vi "Two Parameter.vi"() -> ()   [LabVIEW 2015]
uses:
  <vilib>/Platform/TimedLoop/XDataNode/timing_clust.ctl
  <vilib>/Platform/TimedLoop/XDataNode/nitl_modes.ctl
  <vilib>/Platform/TimedLoop/XDataNode/wakeup.ctl
  <vilib>/DAQmx/read.llb/DAQmx Read (Analog DBL 1Chan 1Samp).vi
  <vilib>/DAQmx/read.llb/DAQmx Read (Analog 1D DBL NChan 1Samp).vi
  <vilib>/DAQmx/create/channels.llb/DAQmx Create Channel (AI-Voltage-Basic).vi
  <vilib>/Enthought/Python Integration Toolkit/api/Unpack Double.vi
  <vilib>/DAQmx/miscellaneous.llb/DAQmx Fill In Error Info.vi
  <vilib>/Platform/TimedLoop/XDataNode/XDataNode.xnode
  Program Files/neMESYS_SDK/neMESYS LabVIEW Kit/neMESYS LabVIEW Integration Kit.lvlib
  <vilib>/Platform/TimedLoop/XDataNode/XDNodeRunTimeDep.lvlib
  Conor/Temp CN7500/Omega CN7500/Omega CN7500.lvlib
  <vilib>/Enthought/Python Integration Toolkit/Python Integration Toolkit.lvlib
panel:
  out "Exp 2":bool
  out "C EB 1":dbl
  out "C BAcid 1":dbl
  out "t ref 8":dbl
  out "t 2 8":dbl
  out "t 1 8":dbl
  out "t ref 7":dbl
  out "t 2 7":dbl
  out "t 1 7":dbl
  out "t ref 6":dbl
  out "t 2 6":dbl
  out "t 1 6":dbl
  out "t ref 5":dbl
  out "t 2 5":dbl
  out "t 1 5":dbl
  out "t ref 4":dbl
  out "t 2 4":dbl
  out "t 1 4":dbl
  out "t ref 3":dbl
  out "t 2 3":dbl
  out "t 1 3":dbl
  out "t ref 2":dbl
  out "t 2 2":dbl
  out "t 1 2":dbl
  out "Exp 9":bool
  out "Liquid Inlet Pressure (bar g)":dbl
  in  "Liquid P sensor Terminal Configuration":i32(ring)=-1 items=["default"=-1, "RSE"=10083, "NRSE"=10078, "Differential"=10106, "Pseudodifferential"=12529]
  in  "Liquid P sensor Physical Channel":tag="Dev1/ai0"
  in  "Temp 2":dbl
  in  "Conc 2":dbl
  in  "Flow 2":dbl
  out "C Int 2 8":dbl
  out "C Int 1 8":dbl
  out "C Int 2 7":dbl
  out "C Int 1 7":dbl
  out "C Int 2 6":dbl
  out "C Int 1 6":dbl
  out "C Int 2 5":dbl
  out "C Int 1 5":dbl
  out "C Int 2 4":dbl
  out "C Int 1 4":dbl
  out "C Int 2 3":dbl
  out "C Int 1 3":dbl
  out "C Int 2 2":dbl
  out "C Int 1 2":dbl
  out "Exp 8":bool
  out "Exp 7":bool
  out "Exp 6":bool
  out "Exp 5":bool
  out "Exp 4":bool
  out "Exp 3":bool
  out "Exp 1":bool
  out "Exp 0":bool
  out "Number Read":dbl
  out "Param 1 8":dbl
  out "Param 2 8":dbl
  out "Chi  8":dbl
  out "Chi ref 8":dbl
  out "C BAcid 8":dbl
  out "C EB 8":dbl
  in  "Flow 8":dbl
  in  "Conc 8":dbl
  in  "Temp 8":dbl
  out "Temp 8":dbl
  out "Flow 8":dbl
  out "Conc 8":dbl
  out "Param 1 7":dbl
  out "Param 2 7":dbl
  out "Chi  7":dbl
  out "Chi ref 7":dbl
  out "C BAcid 7":dbl
  out "C EB 7":dbl
  in  "Flow 7":dbl
  in  "Conc 7":dbl
  in  "Temp 7":dbl
  out "Temp 7":dbl
  out "Flow 7":dbl
  out "Conc 7":dbl
  out "Param 1 6":dbl
  out "Param 2 6":dbl
  out "Chi  6":dbl
  out "Chi ref 6":dbl
  out "C BAcid 6":dbl
  out "C EB 6":dbl
  in  "Flow 6":dbl
  in  "Conc 6":dbl
  in  "Temp 6":dbl
  out "Temp 6":dbl
  out "Flow 6":dbl
  out "Conc 6":dbl
  out "Param 1 5":dbl
  out "Param 2 5":dbl
  out "Chi  5":dbl
  out "Chi ref 5":dbl
  out "C BAcid 5":dbl
  out "C EB 5":dbl
  in  "Flow 5":dbl
  in  "Conc 5":dbl
  in  "Temp 5":dbl
  out "Temp 5":dbl
  out "Flow 5":dbl
  out "Conc 5":dbl
  out "Param 1 4":dbl
  out "Param 2 4":dbl
  out "Chi  4":dbl
  out "Chi ref 4":dbl
  out "C BAcid 4":dbl
  out "C EB 4":dbl
  out "Conc 1":dbl
  out "Flow 1":dbl
  out "Temp 1":dbl
  out "Conc 2":dbl
  out "Flow 2":dbl
  out "Temp 2":dbl
  in  "Flow 4":dbl
  in  "Conc 4":dbl
  in  "Temp 4":dbl
  out "Temp 4":dbl
  out "Flow 4":dbl
  out "Conc 4":dbl
  out "Param 1 3":dbl
  out "Param 2 3":dbl
  out "Chi  3":dbl
  out "Chi ref 3":dbl
  out "C BAcid 3":dbl
  out "C EB 3":dbl
  out "Conc 3":dbl
  out "Flow 3":dbl
  out "Temp 3":dbl
  out "Param 1 2":dbl
  out "Param 2 2":dbl
  out "Chi 2":dbl
  out "Chi ref 2":dbl
  out "C BAcid 2":dbl
  out "C EB 2":dbl
  in  "Temp 3":dbl
  in  "Conc 3":dbl
  in  "Flow 3":dbl
  in  "Result file name - dont need path but need extension .xlsx":string
  in  "HPLC file Name -dont need path, dont need extension":string
  out "Desired Conc Not Possible":bool
  in  "Safety or Emergency Syringe Control":bool
  in  "List or MBDoE":bool
  out "Feed Concentration (M)":dbl
  out "Total Flowrate (uL/min)":dbl
  out "Gas Back Pressure (barg)":dbl
  in  "Shut down in empty?\nLeft off, right on":bool
  out "Text Read From Clipboard 4":string
  out "Read error out 4":errorcluster
  out "Write Set Point Status":string
  out "Error Out 4":i32
  out "Write error out 4":errorcluster
  out "Text Read From Clipboard 3":string
  out "Read error out 3":errorcluster
  out "Read Set Point Status":string
  out "Error Out 3":i32
  out "Write error out 3":errorcluster
  in  "Test Gas Communication":bool
  in  "Change New Set Points":bool
  in  "Read Set Points":bool
  out "Text Read From Clipboard 5":string
  out "Read error out 5":cluster{"source":string}
  out "Write Set Point Status 2":string
  in  "Set Point 1":dbl
  in  "Set Point 2":dbl
  in  "Set Point 3":dbl
  in  "Set Point 4":dbl
  out "Text Read From Clipboard":string
  out "Read error out":errorcluster
  out "Test Status":string
  out "Error Out":i32
  out "Write error out":errorcluster
  out "Text Read From Clipboard 2":string
  out "Read error out 2":errorcluster
  out "Read Flow Status":string
  out "Gas Flow 1":dbl
  out "Gas Flow 2":dbl
  out "Gas Flow 3":dbl
  out "Gas Flow 4":dbl
  out "First waste string":string
  out "Rest of string 1":string
  out "Second Number 2":string
  out "Rest of string 3":string
  out "Third Number 3":string
  out "Rest of string 4":string
  out "Fourth Number 3":string
  out "Rest of string 5":string
  out "Error Out 2":i32
  out "Write error out 2":errorcluster
  in  "Clear":bool
  out "Safety Shut Down Pressure (barg)":dbl
  out "Calculated Pressure":dbl[](graph)
  out "Safety Shut Down Temp":dbl
  out "Actual Temp (oC)":dbl
  out "Temperature":dynamicdata(graph)
  out "Temp Set Point (oC)":dbl
  in  "Temp 1":dbl
  in  "Temp 0":dbl
  in  "Update Temperature Set Point":bool
  in  "Automated Experiments or Direct Control":bool
  in  "Set Point (oC)":dbl
  out "loop ind":dbl
  in  "Stop everything":bool
  in  "Skip Exp":bool
  in  "Minutes between Exp":dbl min=0.0 step=0.05
  in  "Refill 4":bool
  in  "Refill 3":bool
  in  "Refill 2":bool
  in  "Refill 1":bool
  in  "Empty 4":bool
  in  "Empty 3":bool
  in  "Empty 2":bool
  in  "Empty 1":bool
  in  "Calibrate 4":bool
  in  "Calibrate 3":bool
  in  "Calibrate 2":bool
  in  "Calibrate 1":bool
  in  "Stop Dose 4":bool
  in  "Stop Dose 3":bool
  in  "Stop Dose 2":bool
  in  "Stop Dose 1":bool
  in  "Flow 1":dbl
  in  "Conc 1":dbl
  in  "Flow 0":dbl
  in  "Conc 0":dbl
  in  "Generate Flow":bool
  in  "Set Flowrate 1":dbl
  in  "Set Flowrate 2":dbl
  in  "Set Flowrate 3":dbl
  in  "Set Flowrate 4":dbl
  in  "High Conc":dbl min=0.0 max=2.0
  in  "Low Conc":dbl min=0.0 max=2.0
  out "Volumetric Fraction Acid":dbl min=0.0 max=1.0
  out "Syringe Level 4":dbl(slide) scale=0.0..5500.0
  out "Syringe Level 3":dbl(slide) scale=0.0..5500.0
  out "Syringe Level 2":dbl(slide) scale=0.0..5500.0
  out "Syringe Level 1":dbl(slide) scale=0.0..5500.0
  out "Flowrate 4 Ethanol":dbl
  out "Flowrate 3 Acid":dbl
  out "Flowrate 2 High":dbl
  out "Flowrate 1 Low":dbl
  # "Pre Planned Experiments"
  # "Conducted Experiments Set Points"
  # "Safety (start and end)"
  # "Current Conditions"
  # "1 & 2 chosen in advance"
  # "(uL/min)"
  # "3 onwards MBDoE"
  # "Coerced to nearest possible"
  # "Reported Values are set point no actual\nso if set point is not possible\ncoercion takes place\nbut actual is not recorded"
  # "Experimental Info"
  # "Acid must be between 0 and 1, normally 0.1 for 10%"
  # "example file name to show correct format is..."
  # "Direct Control"
  # "MBDoE\nC:\\\\Users\\\\User\\\\Documents\\\\LabVIEW Data\\\\2015 Projects\\\\Combined\\Record.xlsx"
  # "Unit of Gas Flow NmL/min"
  # "I swapped syringe 1 and 2, so now 2 is high and 1 is low"
  # "Emergency Syringe Control Below"
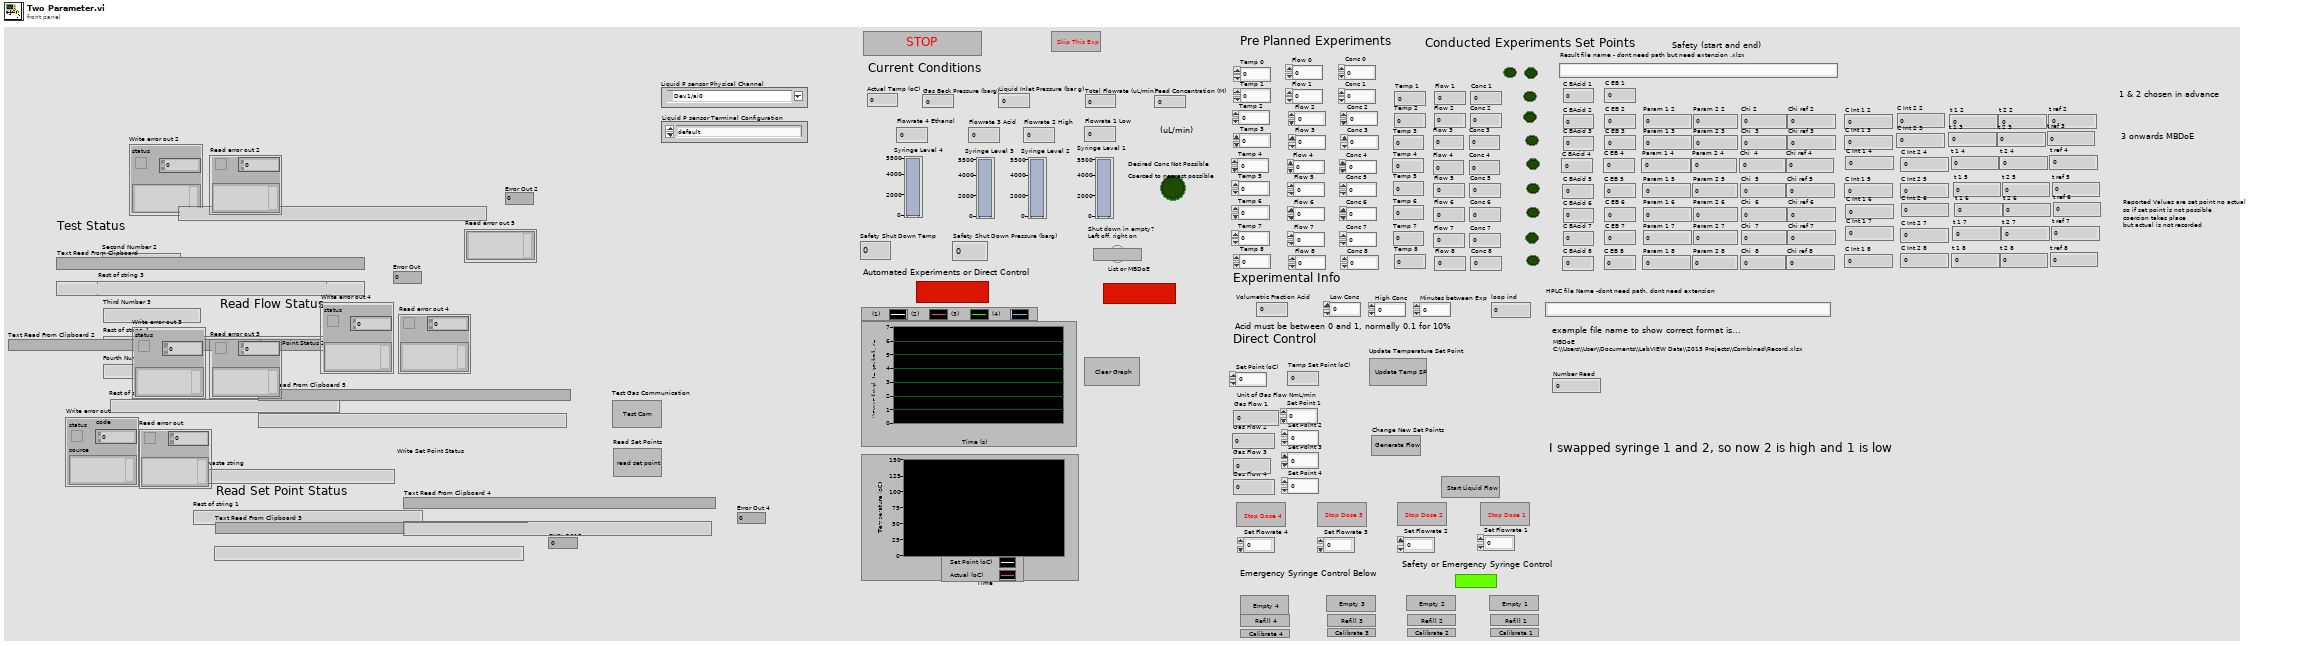
[diagram p1: front panel]
types:
  T1 = typedef "XDNodeRunTimeDep.lvlib/timing_clust.ctl" = cluster{"Expected End [f-1]":u64, "Actual End [f-1]":u64, "Finished Late? [f-1]":bool, "Expected End [i-1]":u64, "Actual End [i-1]":u64, "Finished Late? [i-1]":bool, "Expected Start [i]":u64, "Actual Start [i]":u64, "Expected Start [f]":u64, "Actual Start [f]":u64, "Source Name":string, "Structure Name":string, "Period":i64, "Deadline":i64, "Offset":i64, "Start":i64, "Priority":i32, "Timeout":i32, "Mode":T2, "Wakeup Reason":T3, "Error":errorcluster, "Source Type":string, "Secondary Source Type":string, "Global End Time":u64, "Global Start Time":u64, "Frame Duration":u64, "Iteration Duration":u64, "Assigned CPU":i32, "I/O Scan Engine Mode":u32}
  T2 = typedef "XDNodeRunTimeDep.lvlib/nitl_modes.ctl" = enum32{"No Change", "Process missed periods, maintain original phase", "Discard missed periods, maintain original phase", "Process missed periods, ignore original phase", "Discard missed periods, ignore original phase"}
  T3 = typedef "XDNodeRunTimeDep.lvlib/wakeup.ctl" = enum32{"Normal", "Aborted", "Asynchronous wakeup", "Timing source error", "Timed loop error", "Timeout"}
  T4 = typedef "Python Integration Toolkit.lvlib/Session ID.ctl" = u64
  T5 = typedef "Python Integration Toolkit.lvlib/Python Objects.ctl" = variant
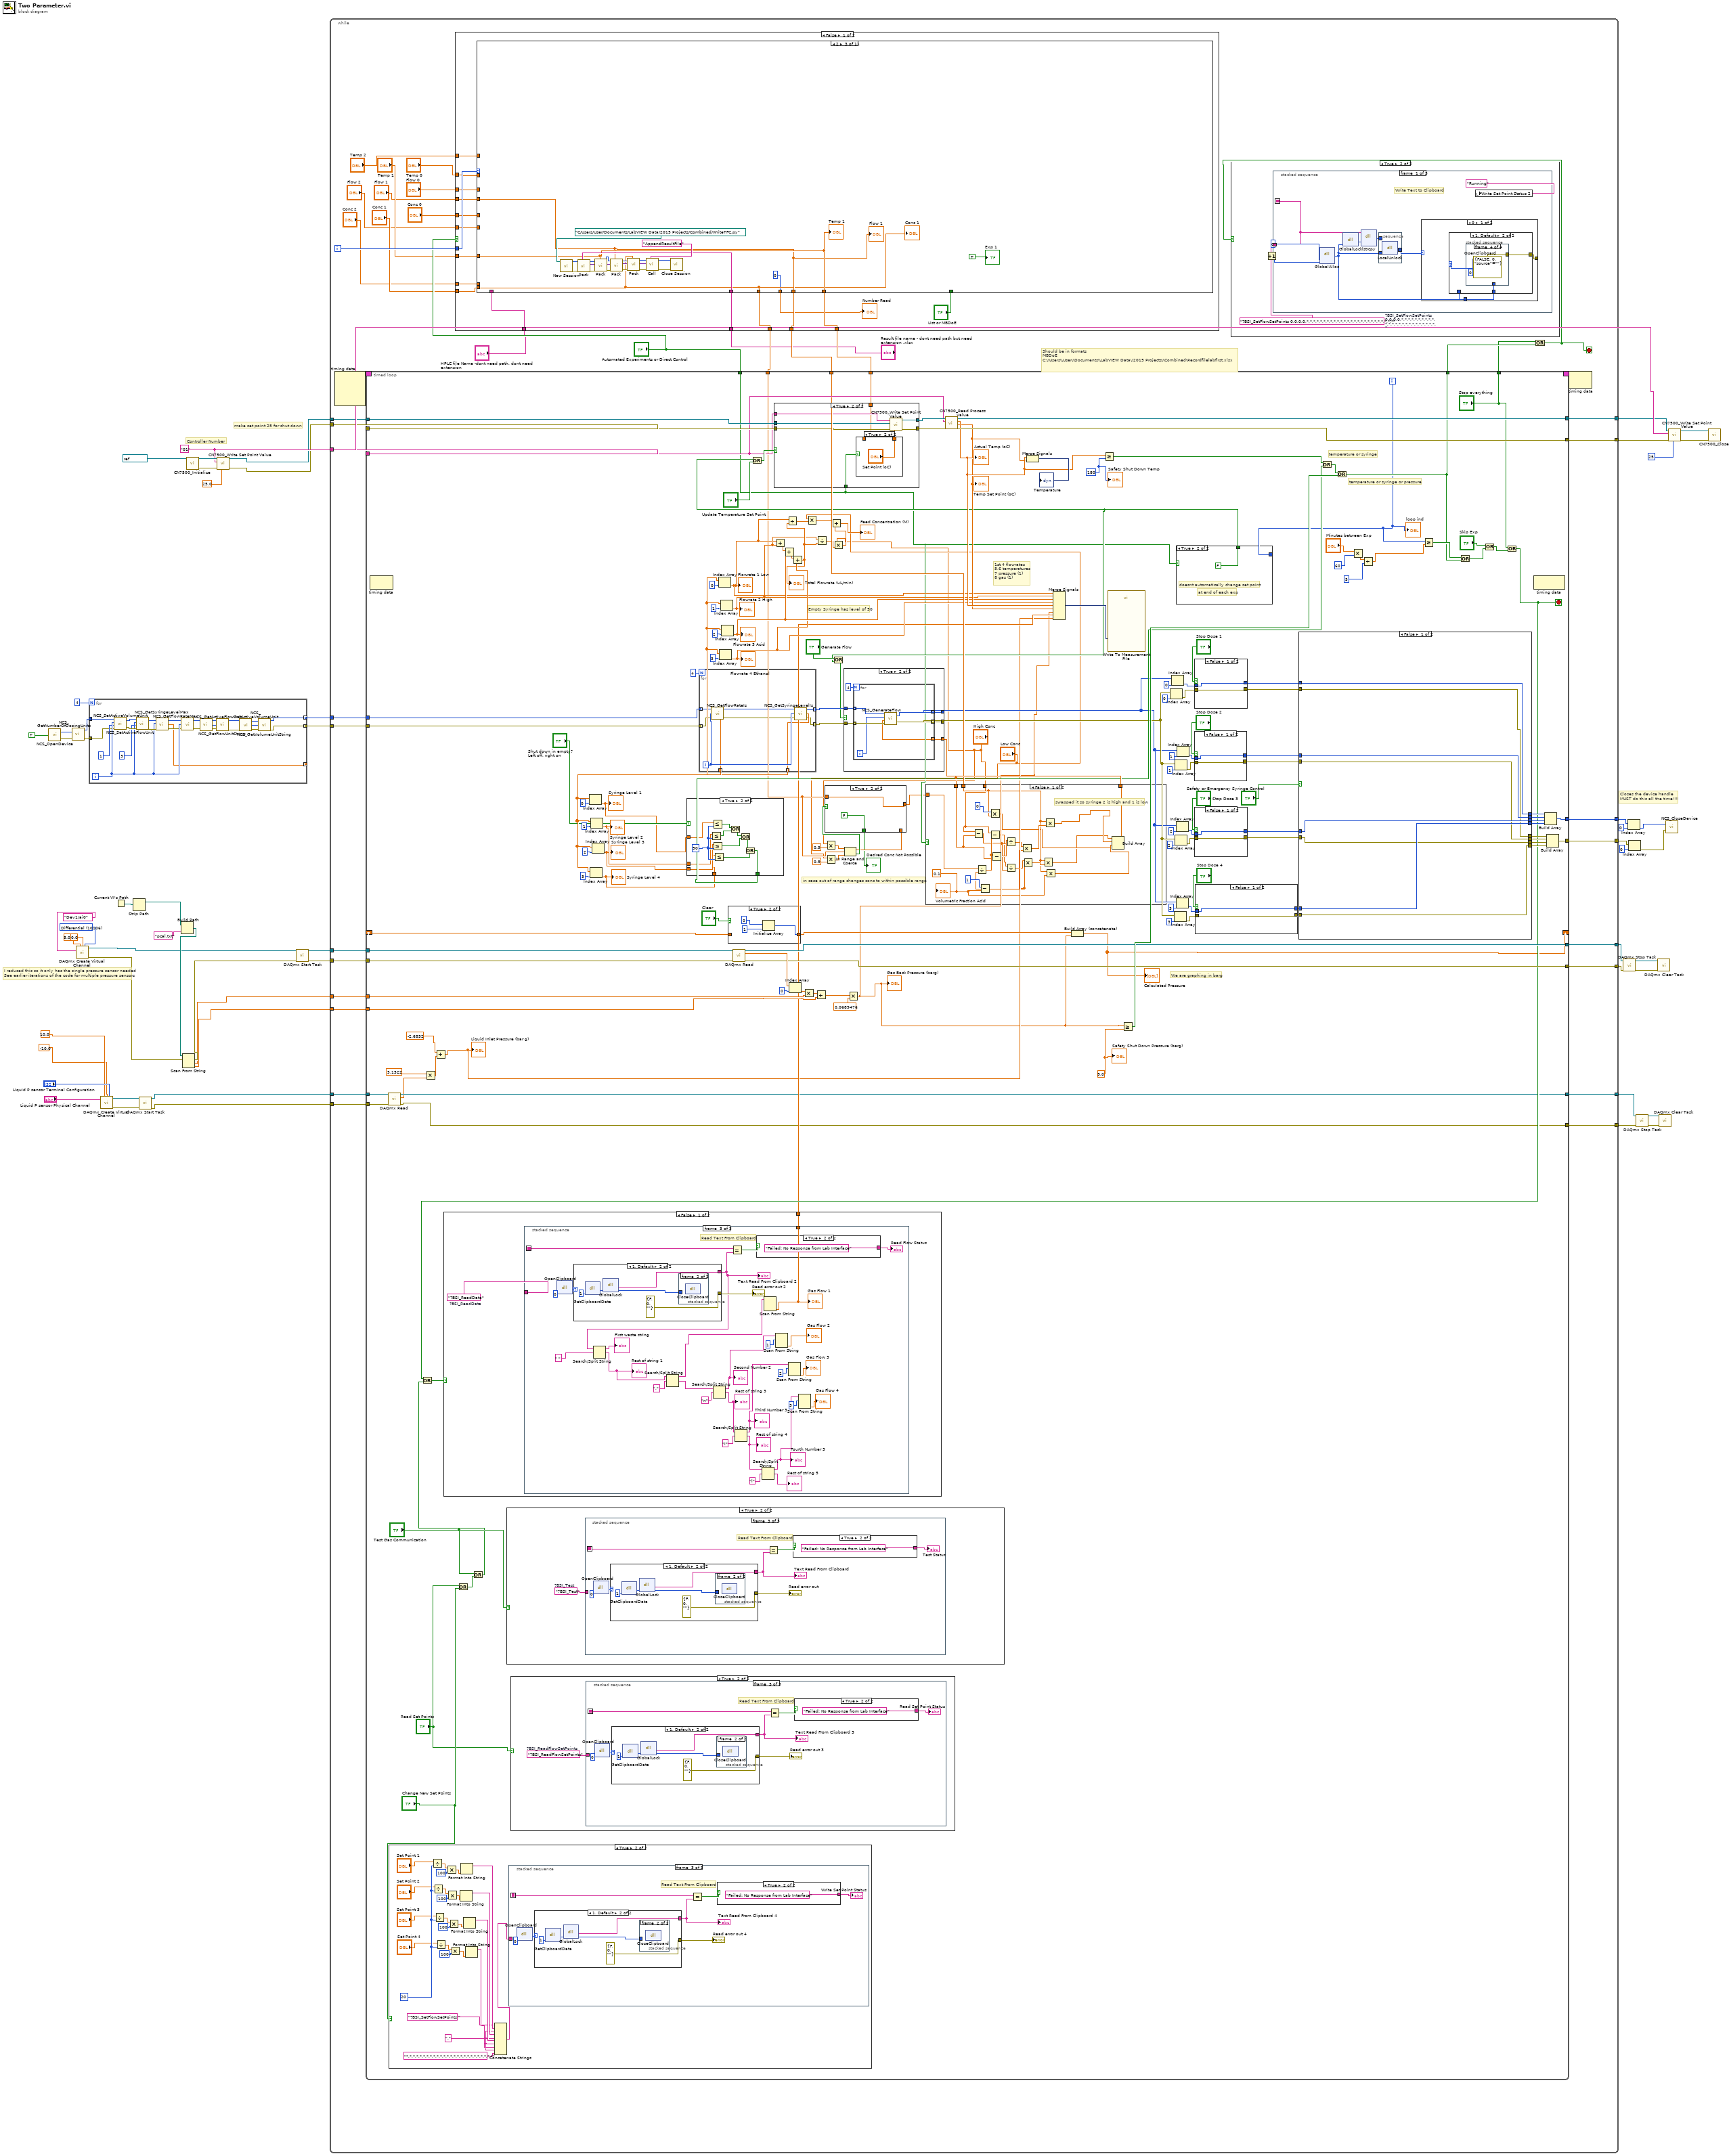
[diagram p0: block diagram]
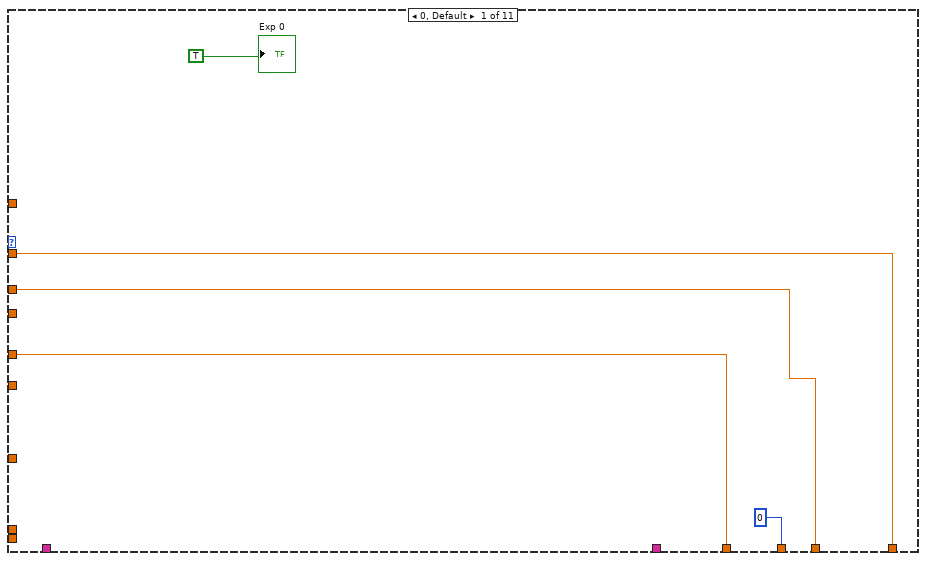
[diagram p2: hidden frame]
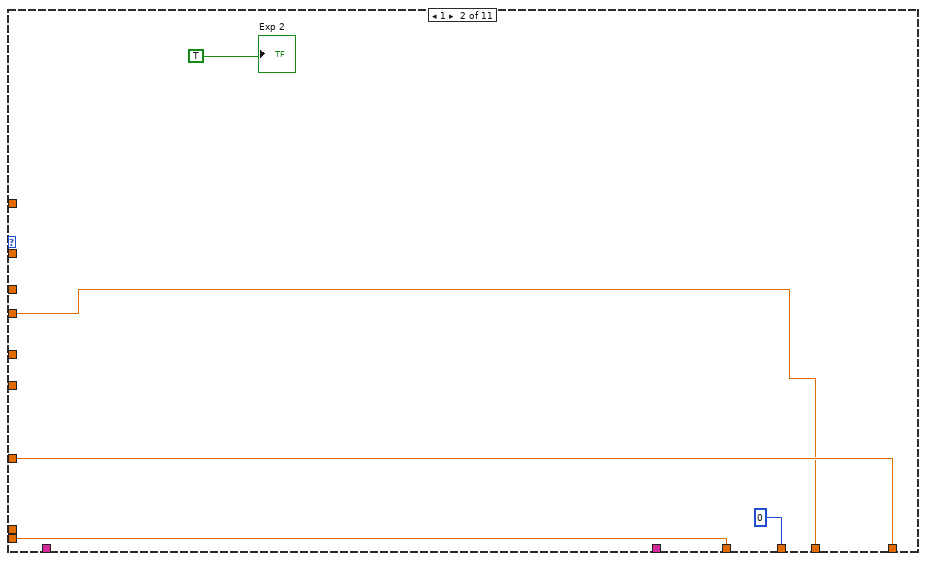
[diagram p3: hidden frame]
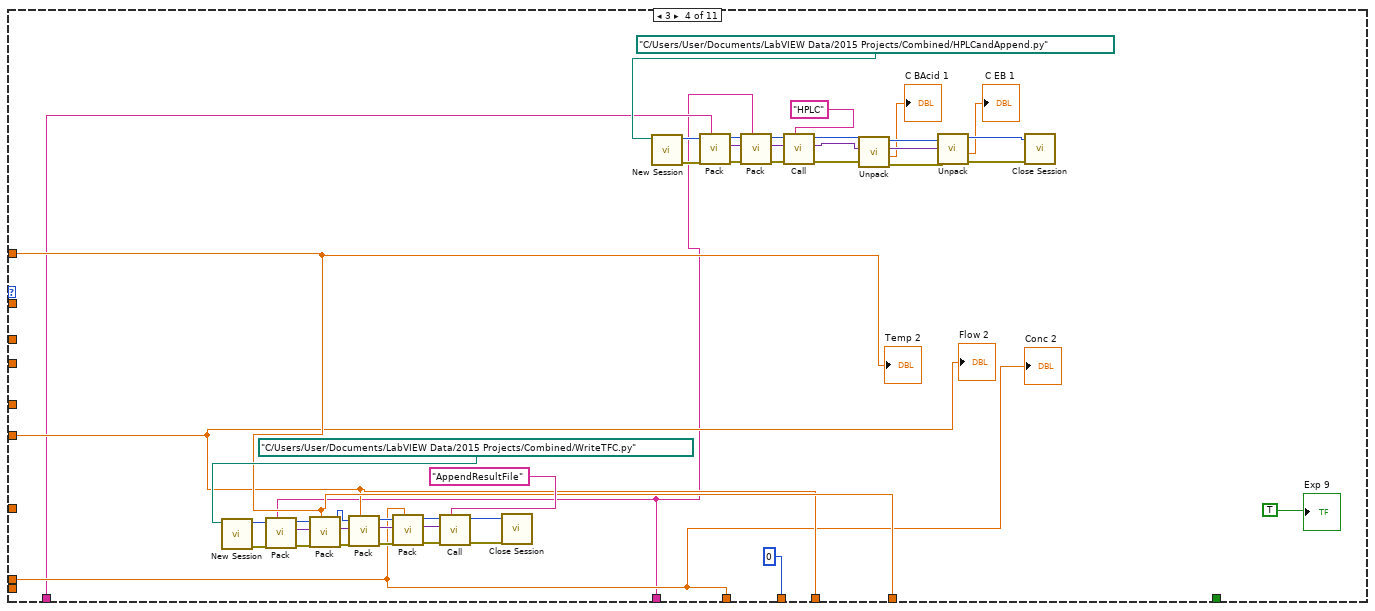
[diagram p4: hidden frame]
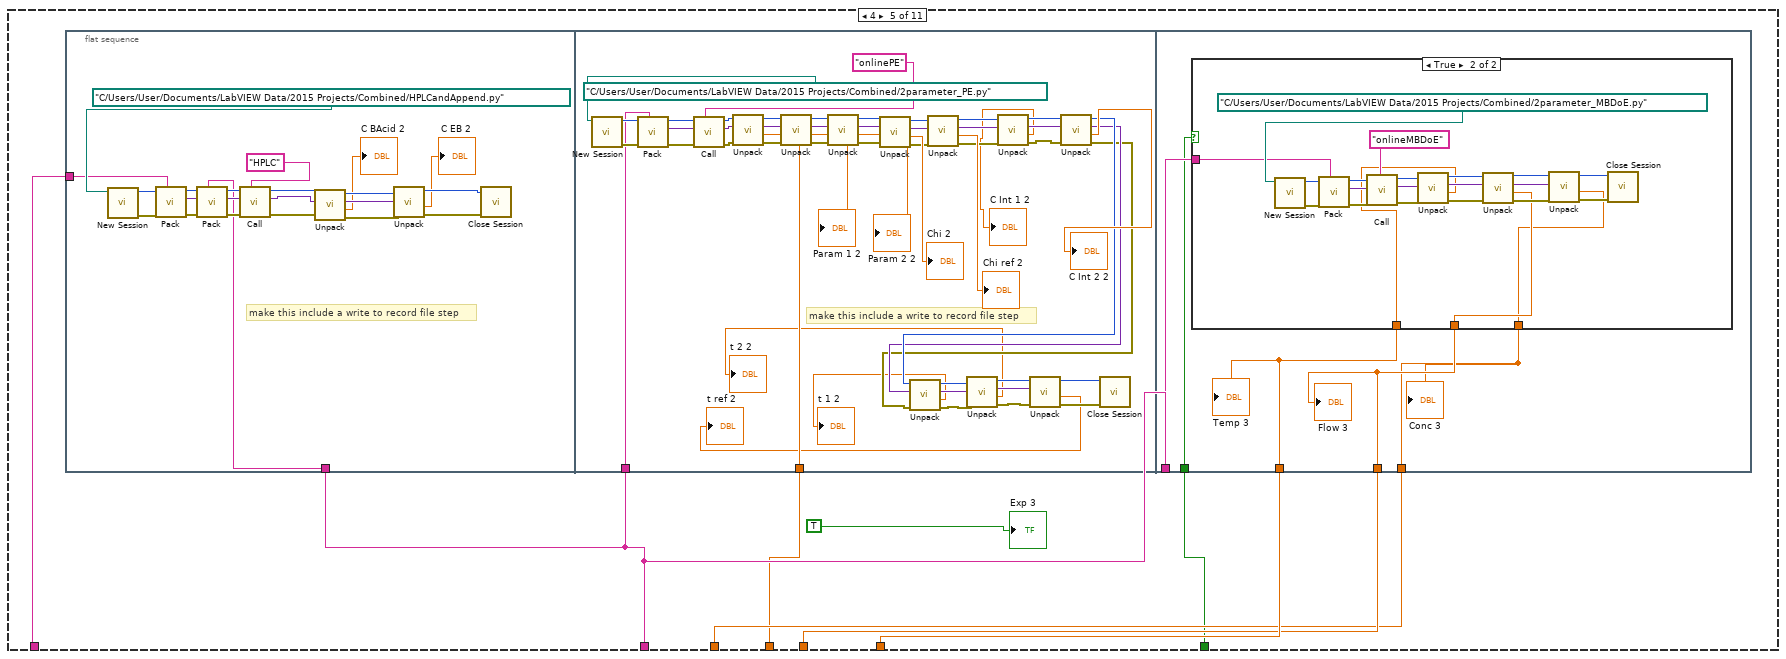
[diagram p5: hidden frame]
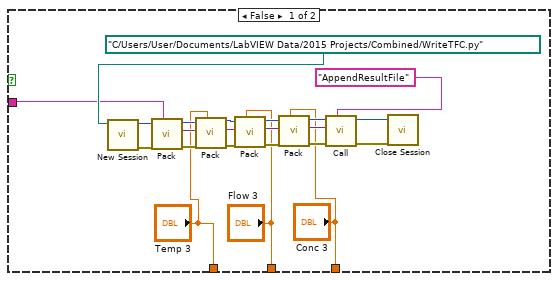
[diagram p6: hidden frame]
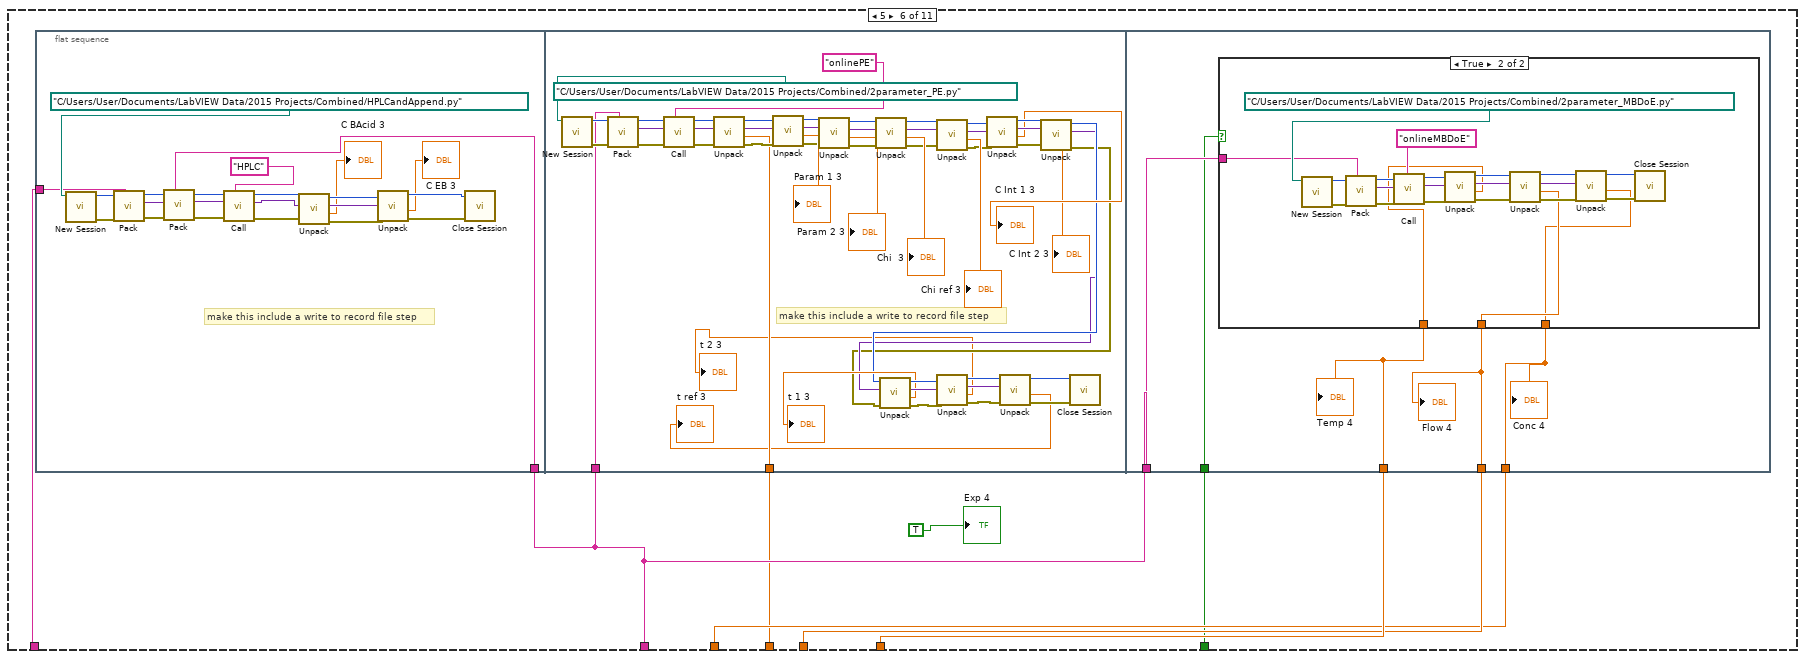
[diagram p7: hidden frame]
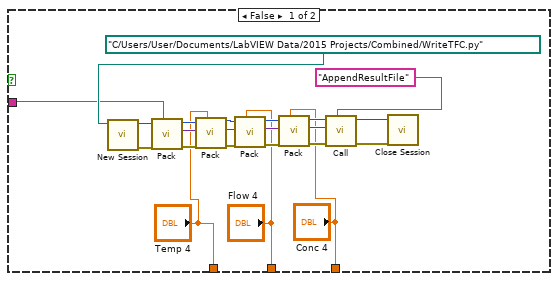
[diagram p8: hidden frame]
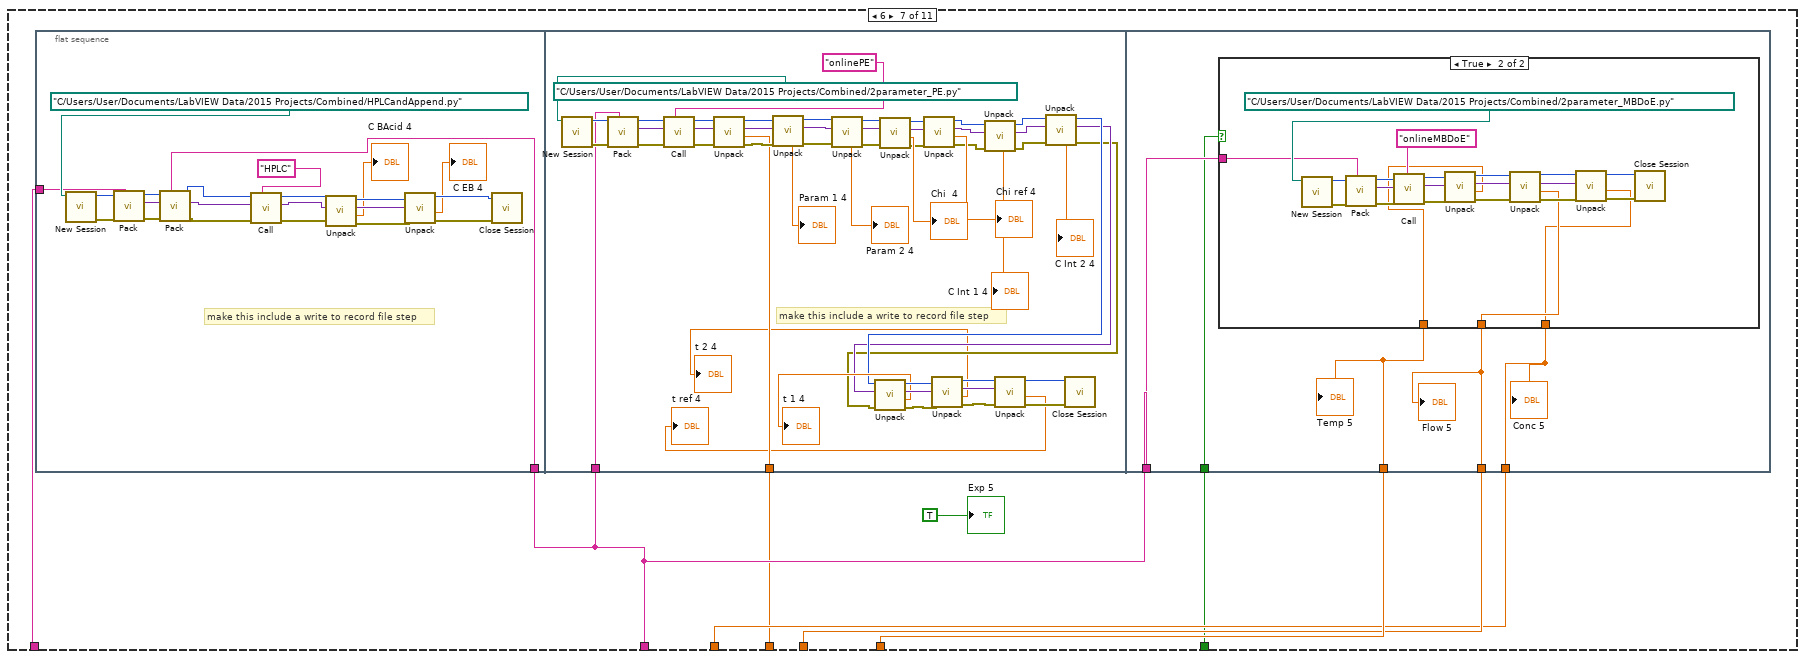
[diagram p9: hidden frame]
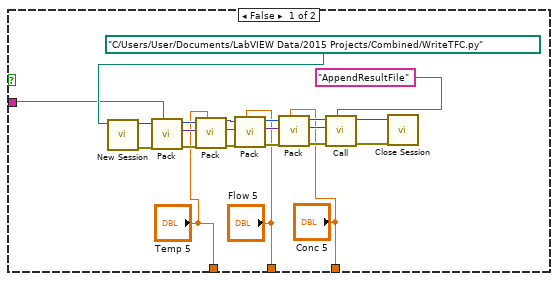
[diagram p10: hidden frame]
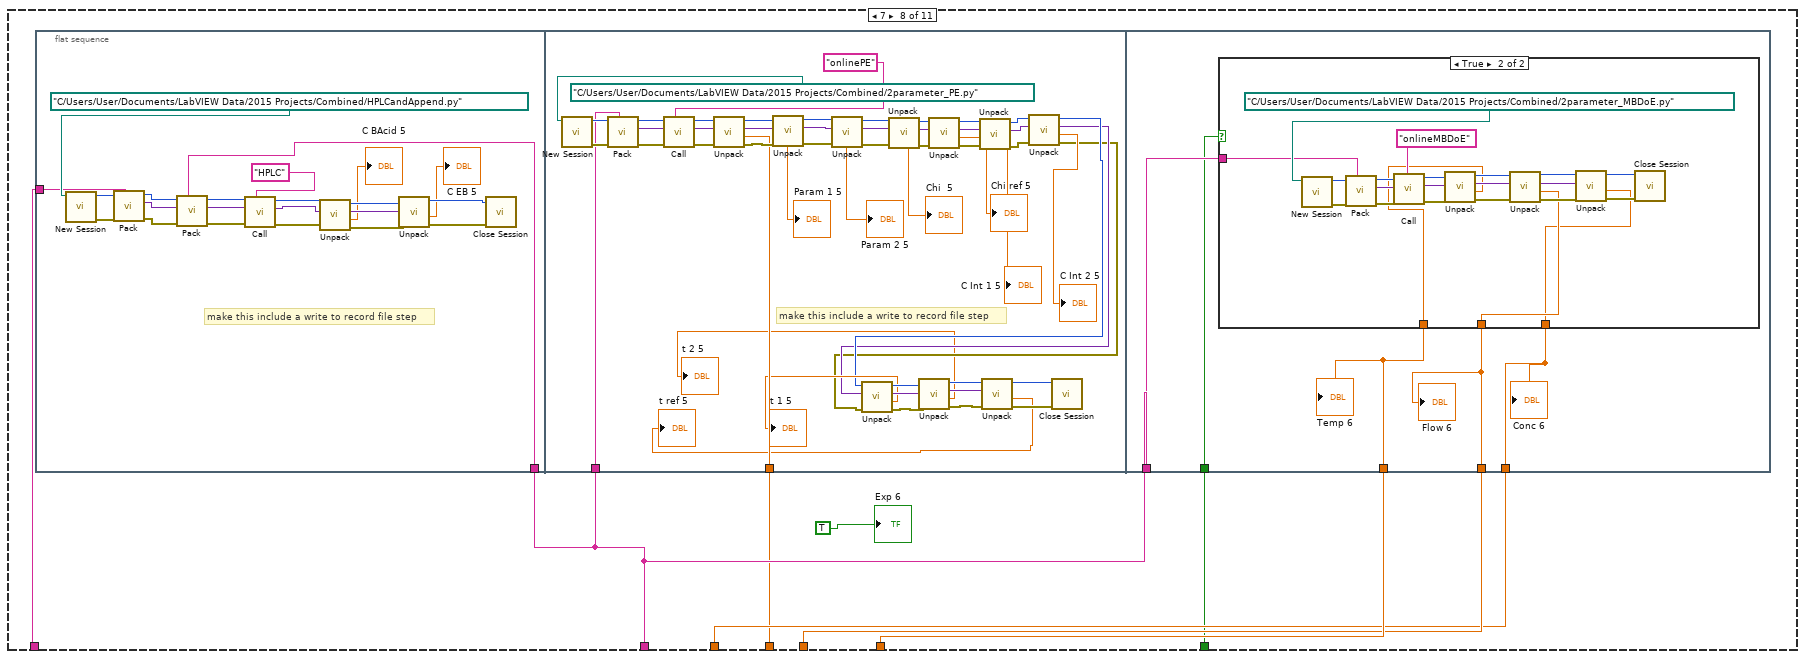
[diagram p11: hidden frame]
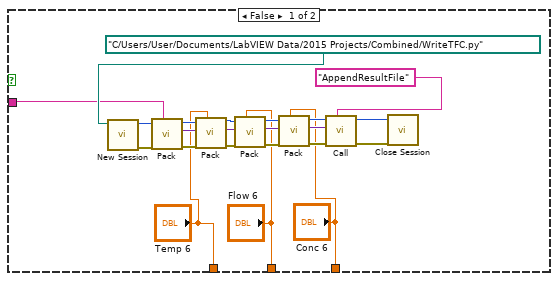
[diagram p12: hidden frame]
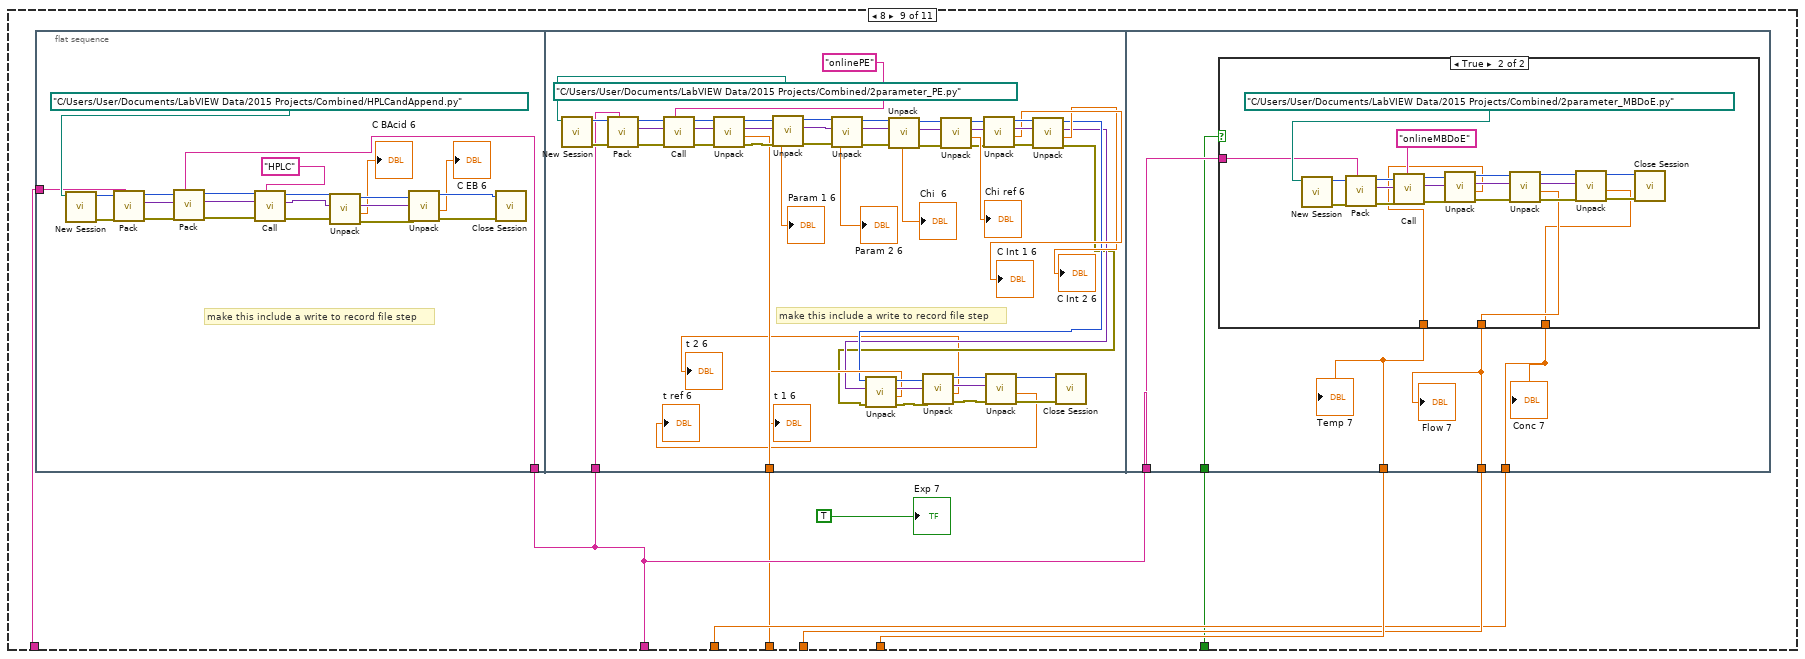
[diagram p13: hidden frame]
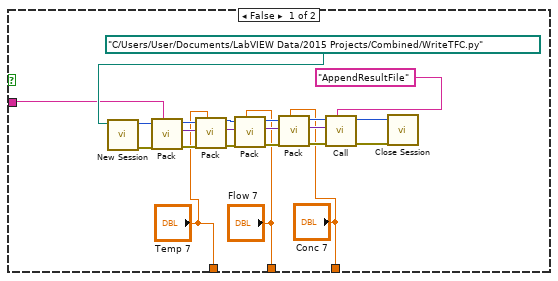
[diagram p14: hidden frame]
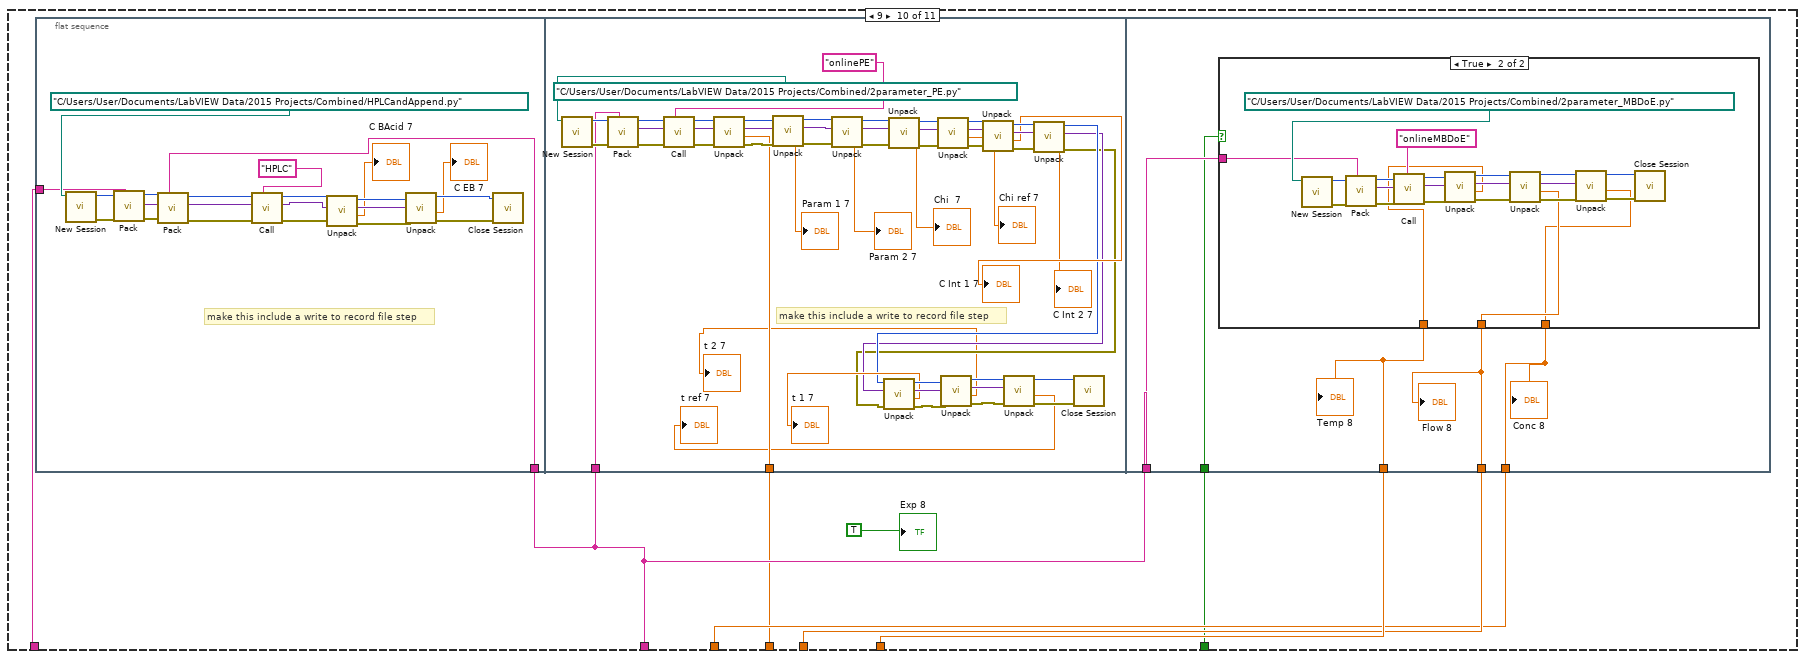
[diagram p15: hidden frame]
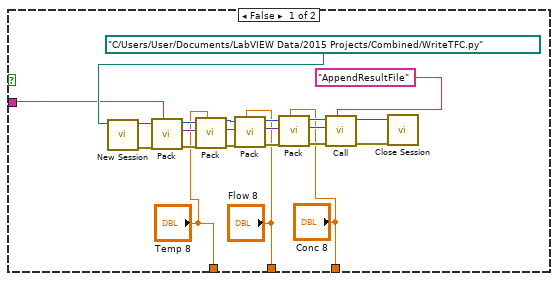
[diagram p16: hidden frame]
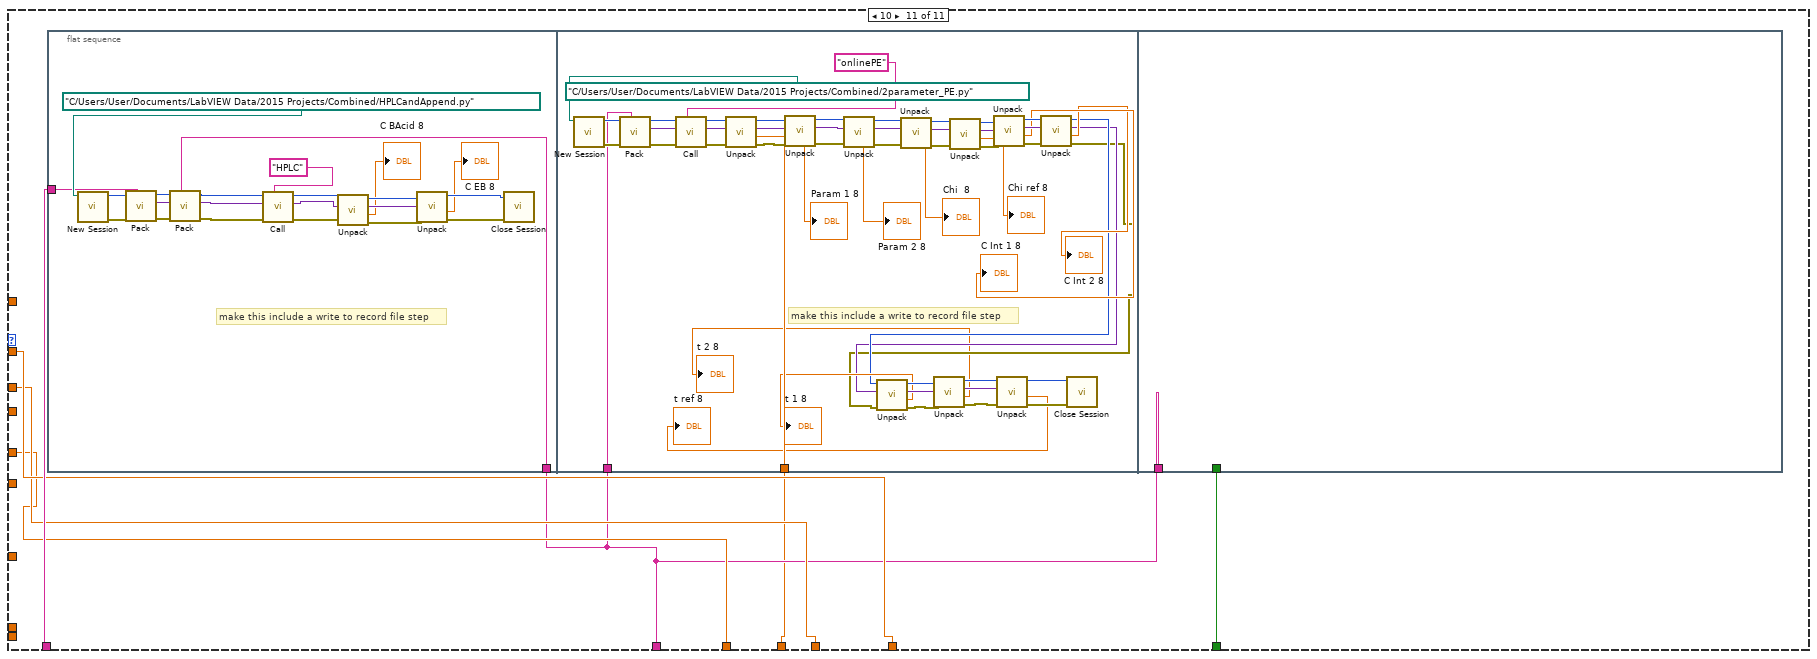
[diagram p17: hidden frame]
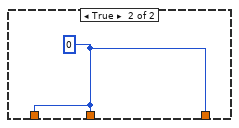
[diagram p18: hidden frame]
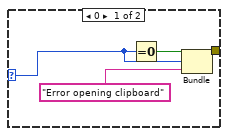
[diagram p20: hidden frame]
diagram:
  w29 = 10106 items=["default"=-1, "RSE"=10083, "NRSE"=10078, "Differential"=10106, "Pseudodifferential"=12529] ("input terminal configuration")
  w36 = "01" ("Controller Number")
  # "I reduced this so it only has the single pressure sensor needed\nSee earlier iterations of the code for multiple pressure sensors"
  # "make set point 25 for shut down"
  # "Controller Number"
  # "Closes the device handle \nMUST do this all the time!!!!"
  n1 = call "NCS_OpenDevice.vi"("show status window"=TRUE) -> ("device handle"=w55:u32, "error out"=w54:errorcluster)
  n2 = call "NCS_GetNumberOfDosingUnits.vi"("device handle in"=w55, "error in (no error)"=w54) -> ("device handle out"=w52:u32, "error out"=w53:errorcluster)  [unwired: 1 out]
  n3 = call-poly <vilib>:"DAQmx Create Virtual Channel.vi"("maximum value"=5.0, "minimum value"=0.0, "input terminal configuration"=w29, "physical channels"=tag "Dev1/ai0") -> ("task out"=w13:refnum<k21>, "error out"=w14:errorcluster)  [unwired: 10 in]
  n4 = for {
    N: 4 -> [_]
    tunnel: [w61] -> w51 mode=indexing
    tunnel: [w60] -> w50 mode=indexing
    tunnel: [w74] -> _ mode=indexing
    tunnel: w53 -> [w59]
    tunnel: w52 -> [w58]
    i -> [w77]
    n5 = call "NCS_SetActiveVolumeUnit.vi"("error in (no error)"=w59, "active volume unit"=1, "dosingunit"=w77, "device handle in"=w58) -> ("error out"=w80:errorcluster, "device handle out"=w81:u32)
    n6 = call "NCS_SetActiveFlowUnit.vi"("error in (no error)"=w80, "active flow unit"=3, "dosingunit"=w77, "device handle in"=w81) -> ("error out"=w78:errorcluster, "device handle out"=w79:u32)
    n7 = call "NCS_GetSyringeLevelMax.vi"("error in (no error)"=w78, "dosingunit"=w77, "device handle in"=w79) -> ("error out"=w75:errorcluster, "syringe level max"=w74:dbl, "device handle out"=w76:u32)  [unwired: 1 out]
    n8 = call "NCS_GetFlowRateMax.vi"("error in (no error)"=w75, "dosingunit"=w77, "device handle in"=w76) -> ("error out"=w62:errorcluster, "device handle out"=w63:u32)  [unwired: 1 out]
    n9 = call "NCS_GetActiveFlowUnit.vi"("error in (no error)"=w62, "device handle in"=w63) -> ("error out"=w70:errorcluster, "active flow unit"=w69:u8, "device handle out"=w71:u32)  [unwired: 1 in]
    n10 = call "NCS_GetFlowUnitString.vi"("device handle in"=w71, "flow unit id"=w69, "error in (no error)"=w70) -> ("device handle out"=w66:u32, "error out"=w65:errorcluster)  [unwired: 2 out]
    n11 = call "NCS_GetActiveVolumeUnit.vi"("error in (no error)"=w65, "device handle in"=w66) -> ("error out"=w67:errorcluster, "active volume unit"=w68:u8, "device handle out"=w64:u32)  [unwired: 1 in]
    n12 = call "NCS_GetVolumeUnitString.vi"("device handle in"=w64, "volume unit id"=w68, "error in (no error)"=w67) -> ("device handle out"=w61:u32, "error out"=w60:errorcluster)  [unwired: 2 out]
  }
  n13 = call-poly <vilib>:"DAQmx Create Virtual Channel.vi"("maximum value"=10.0, "minimum value"=-10.0 ("maximum value"), "input terminal configuration"="Liquid P sensor Terminal Configuration", "physical channels"="Liquid P sensor Physical Channel") -> ("task out"=w9:refnum<k21>, "error out"=w10:errorcluster)  [unwired: 10 in]
  n14 = Current VI's Path() -> (path=w27:path)
  n15 = Strip Path(path=w27) -> (stripped path=w25:path)  [unwired: 1 out]
  n16 = call <vilib>:"DAQmx Start Task.vi"("task/channels in"=w9, "error in"=w10) -> ("task out"=w8:refnum<k21>, "error out"=w7:errorcluster)  [unwired: 12 in]
  n17 = Build Path(base path=w25, name or relative path="pcal.txt") -> (appended path=w26:path)
  n18 = Scan From String(w26, w14) -> (w23:errorcluster, output 1=w20:dbl, output 2=w19:dbl)  [unwired: 3 in, 1 out]
  n19 = call "CN7500_Initialize.vi"("VISA resource name"=refnum<visa-resource-name> "COM8") -> ("error out"=w42:errorcluster, "VISA resource name out"=w43:refnum<visa-resource-name>)  [unwired: 9 in]
  n20 = call "CN7500_Write Set Point Value.vi"("Target Set Point Value"=25.0, "error in (no error)"=w42, "Controller Number"=w36, "VISA In"=w43) -> ("error out"=w34:errorcluster, "VISA Out"=w35:refnum<visa-resource-name>)  [unwired: 6 in]
  n21 = call <vilib>:"DAQmx Start Task.vi"("task/channels in"=w13, "error in"=w23) -> ("task out"=w22:refnum<k21>, "error out"=w21:errorcluster)  [unwired: 12 in]
  n22 = while {
    tunnel: w51 -> [w121]
    tunnel: w50 -> [w120]
    tunnel: [w119] -> w45
    tunnel: [w118] -> w44
    tunnel: w36 -> [w115]
    tunnel: w35 -> [w114]
    tunnel: w34 -> [w113]
    tunnel: [w112] -> w33
    tunnel: [w111] -> w32
    tunnel: w22 -> [w109]
    tunnel: w21 -> [w108]
    tunnel: w20 -> [w107]
    tunnel: w19 -> [w106]
    tunnel: [w105] -> w16
    tunnel: [w104] -> w15
    tunnel: w8 -> [w88]
    tunnel: w7 -> [w87]
    tunnel: [w86] -> w5
    tunnel: [w85] -> w3
    i -> [w98]
    stop <- w103 stop-if-true
    # "Should be in formats \nMBDoE\nC:\\\\Users\\\\User\\\\Documents\\\\LabVIEW Data\\\\2015 Projects\\\\Combined\\Recordfilelabfirst.xlsx"
    n23 = node-c288() -> (w117:T1)  [unwired: 4 in]
    n24 = case shown="False" "Automated Experiments or Direct Control" {
      tunnel: [w135 w1071] -> w101
      tunnel: [w133 w1071] -> w100
      tunnel: [w137 w1071] -> w99
      tunnel: w98 -> [w138 _]
      tunnel: "Conc 0" -> [w136 _]
      tunnel: "Flow 0" -> [w132 _]
      tunnel: "Temp 0" -> [w134 _]
      tunnel: "Temp 1" -> [w130 _]
      tunnel: "Flow 1" -> [w129 _]
      tunnel: "Conc 1" -> [w128 _]
      tunnel: "HPLC file Name -dont need path, dont need extension" -> [w127 _]
      tunnel: "Result file name - dont need path but need extension .xlsx" -> [w131 _]
      tunnel: "Temp 2" -> [w124 _]
      tunnel: "Flow 2" -> [w123 _]
      tunnel: "Conc 2" -> [w122 _]
      frame False {
        n25 = case shown="2" w138 {
          tunnel: [w141 w144 w151 w195 w222 w351 w480 w609 w738 w867 w994] -> w137
          tunnel: w136 -> [w141 _ _ _ _ _ _ _ _ _ w994]
          tunnel: [w143 w146 w153 w197 w224 w353 w482 w611 w740 w869 w996] -> w135
          tunnel: w134 -> [w143 _ _ _ _ _ _ _ _ _ w996]
          tunnel: [w142 w145 w152 w196 w223 w352 w481 w610 w739 w868 w995] -> w133
          tunnel: w132 -> [w142 _ _ _ _ _ _ _ _ _ w995]
          tunnel: w131 -> [_ _ w154 w173 w220 w349 w478 w607 w736 w865 w993]
          tunnel: w130 -> [_ w146 w153 _ _ _ _ _ _ _ _]
          tunnel: w129 -> [_ w145 w152 _ _ _ _ _ _ _ _]
          tunnel: w128 -> [_ w144 w151 _ _ _ _ _ _ _ _]
          tunnel: w127 -> [_ _ _ w174 w225 w354 w483 w612 w741 w870 w998]
          tunnel: "List or MBDoE" -> [_ _ _ _ w221 w350 w479 w608 w737 w866 w997]
          tunnel: [0 0 0 0 w219 w348 w477 w606 w735 w864 w992] -> w125
          tunnel: w124 -> [_ _ _ w197 _ _ _ _ _ _ _]
          tunnel: w123 -> [_ _ _ w196 _ _ _ _ _ _ _]
          tunnel: w122 -> [_ _ _ w195 _ _ _ _ _ _ _]
          frame 0, Default {
            "Exp 0" <- TRUE
          }
          frame 1 {
            "Exp 2" <- TRUE
          }
          frame 2 {
            n26 = call <vilib>:"New Session.vi"("Path to Python Module (.py File)"=path "C:/Users/User/Documents/LabVIEW Data/2015 Projects/Combined/WriteTFC.py") -> ("error out"=w164:errorcluster, "Session ID out"=w163:T4)  [unwired: 9 in]
            n27 = call <vilib>:"Pack.vi"("Argument"=w154, "error in (no error)"=w164, "Session ID"=w163) -> ("error out"=w165:errorcluster, "Python Object References Out"=w169:T5, "Session ID out"=w162:T4)  [unwired: 6 in]
            n28 = call <vilib>:"Pack.vi"("Argument"=w153, "error in (no error)"=w165, "Python Object References In"=w169, "Session ID"=w162) -> ("error out"=w166:errorcluster, "Python Object References Out"=w170:T5, "Session ID out"=w172:T4)  [unwired: 5 in]
            n29 = call <vilib>:"Pack.vi"("Argument"=w152, "error in (no error)"=w166, "Python Object References In"=w170, "Session ID"=w172) -> ("error out"=w167:errorcluster, "Python Object References Out"=w171:T5, "Session ID out"=w158:T4)  [unwired: 5 in]
            n30 = call <vilib>:"Pack.vi"("Argument"=w151, "error in (no error)"=w167, "Python Object References In"=w171, "Session ID"=w158) -> ("error out"=w155:errorcluster, "Python Object References Out"=w156:T5, "Session ID out"=w157:T4)  [unwired: 5 in]
            n31 = call <vilib>:"Call.vi"("Function or Method Name"="AppendResultFile", "error in (no error)"=w155, "Python Object References In"=w156, "Session ID"=w157) -> ("error out"=w168:errorcluster, "Session ID out"=w159:T4)  [unwired: 5 in, 1 out]
            n32 = call <vilib>:"Close Session.vi"("error in (no error)"=w168, "Session ID"=w159) -> ()  [unwired: 9 in, 1 out]
            "Temp 1" <- w153
            "Flow 1" <- w152
            "Conc 1" <- w151
            "Exp 1" <- TRUE
          }
          frame 3 {
            n33 = call <vilib>:"New Session.vi"("Path to Python Module (.py File)"=path "C:/Users/User/Documents/LabVIEW Data/2015 Projects/Combined/WriteTFC.py") -> ("error out"=w209:errorcluster, "Session ID out"=w208:T4)  [unwired: 9 in]
            n34 = call <vilib>:"Pack.vi"("Argument"=w173, "error in (no error)"=w209, "Session ID"=w208) -> ("error out"=w210:errorcluster, "Python Object References Out"=w214:T5, "Session ID out"=w207:T4)  [unwired: 6 in]
            n35 = call <vilib>:"Pack.vi"("Argument"=w197, "error in (no error)"=w210, "Python Object References In"=w214, "Session ID"=w207) -> ("error out"=w211:errorcluster, "Python Object References Out"=w215:T5, "Session ID out"=w217:T4)  [unwired: 5 in]
            n36 = call <vilib>:"Pack.vi"("Argument"=w196, "error in (no error)"=w211, "Python Object References In"=w215, "Session ID"=w217) -> ("error out"=w212:errorcluster, "Python Object References Out"=w216:T5, "Session ID out"=w203:T4)  [unwired: 5 in]
            n37 = call <vilib>:"Pack.vi"("Argument"=w195, "error in (no error)"=w212, "Python Object References In"=w216, "Session ID"=w203) -> ("error out"=w200:errorcluster, "Python Object References Out"=w201:T5, "Session ID out"=w202:T4)  [unwired: 5 in]
            n38 = call <vilib>:"Call.vi"("Function or Method Name"="AppendResultFile", "error in (no error)"=w200, "Python Object References In"=w201, "Session ID"=w202) -> ("error out"=w213:errorcluster, "Session ID out"=w204:T4)  [unwired: 5 in, 1 out]
            n39 = call <vilib>:"Close Session.vi"("error in (no error)"=w213, "Session ID"=w204) -> ()  [unwired: 9 in, 1 out]
            n40 = call <vilib>:"New Session.vi"("Path to Python Module (.py File)"=path "C:/Users/User/Documents/LabVIEW Data/2015 Projects/Combined/HPLCandAppend.py") -> ("error out"=w191:errorcluster, "Session ID out"=w190:T4)  [unwired: 9 in]
            n41 = call <vilib>:"Pack.vi"("Argument"=w174, "error in (no error)"=w191, "Session ID"=w190) -> ("error out"=w176:errorcluster, "Python Object References Out"=w178:T5, "Session ID out"=w180:T4)  [unwired: 6 in]
            n42 = call <vilib>:"Pack.vi"("Argument"=w173, "error in (no error)"=w176, "Python Object References In"=w178, "Session ID"=w180) -> ("error out"=w175:errorcluster, "Python Object References Out"=w177:T5, "Session ID out"=w179:T4)  [unwired: 5 in]
            n43 = call <vilib>:"Call.vi"("Function or Method Name"="HPLC", "error in (no error)"=w175, "Python Object References In"=w177, "Session ID"=w179) -> ("error out"=w192:errorcluster, "Python Object References Out"=w183:T5, "Session ID out"=w184:T4)  [unwired: 5 in]
            n44 = call-poly <vilib>:"Unpack.vi"("error in (no error)"=w192, "Python Object References In"=w183, "Session ID"=w184) -> ("error out"=w193:errorcluster, "Value"=→"C BAcid 1":dbl, "Python Object References Out"=w188:T5, "Session ID out"=w187:T4)  [unwired: 5 in]
            n45 = call-poly <vilib>:"Unpack.vi"("error in (no error)"=w193, "Python Object References In"=w188, "Session ID"=w187) -> ("error out"=w194:errorcluster, "Value"=→"C EB 1":dbl, "Session ID out"=w189:T4)  [unwired: 5 in, 1 out]
            n46 = call <vilib>:"Close Session.vi"("error in (no error)"=w194, "Session ID"=w189) -> ()  [unwired: 9 in, 1 out]
            "Exp 9" <- TRUE
            "Temp 2" <- w197
            "Flow 2" <- w196
            "Conc 2" <- w195
          }
          frame 4 {
            n47 = flat-sequence {
              tunnel: w225 -> [w233]
              tunnel: w220 -> [w226]
              tunnel: w220 -> [w272]
              tunnel: [w270] -> w219
              tunnel: w220 -> [w302]
              tunnel: [w301] -> w224
              tunnel: [w300] -> w223
              tunnel: [w299] -> w222
              tunnel: w221 -> [w298]
              frame #0 {
                # "make this include a write to record file step"
                n48 = call <vilib>:"New Session.vi"("Path to Python Module (.py File)"=path "C:/Users/User/Documents/LabVIEW Data/2015 Projects/Combined/HPLCandAppend.py") -> ("error out"=w244:errorcluster, "Session ID out"=w243:T4)  [unwired: 9 in]
                n49 = call <vilib>:"Pack.vi"("Argument"=w233, "error in (no error)"=w244, "Session ID"=w243) -> ("error out"=w228:errorcluster, "Python Object References Out"=w230:T5, "Session ID out"=w232:T4)  [unwired: 6 in]
                n50 = call <vilib>:"Pack.vi"("Argument"=w226, "error in (no error)"=w228, "Python Object References In"=w230, "Session ID"=w232) -> ("error out"=w227:errorcluster, "Python Object References Out"=w229:T5, "Session ID out"=w231:T4)  [unwired: 5 in]
                n51 = call <vilib>:"Call.vi"("Function or Method Name"="HPLC", "error in (no error)"=w227, "Python Object References In"=w229, "Session ID"=w231) -> ("error out"=w245:errorcluster, "Python Object References Out"=w236:T5, "Session ID out"=w237:T4)  [unwired: 5 in]
                n52 = call-poly <vilib>:"Unpack.vi"("error in (no error)"=w245, "Python Object References In"=w236, "Session ID"=w237) -> ("error out"=w246:errorcluster, "Value"=→"C BAcid 2":dbl, "Python Object References Out"=w241:T5, "Session ID out"=w240:T4)  [unwired: 5 in]
                n53 = call-poly <vilib>:"Unpack.vi"("error in (no error)"=w246, "Python Object References In"=w241, "Session ID"=w240) -> ("error out"=w247:errorcluster, "Value"=→"C EB 2":dbl, "Session ID out"=w242:T4)  [unwired: 5 in, 1 out]
                n54 = call <vilib>:"Close Session.vi"("error in (no error)"=w247, "Session ID"=w242) -> ()  [unwired: 9 in, 1 out]
              }
              frame #1 {
                # "make this include a write to record file step"
                n55 = call <vilib>:"New Session.vi"("Path to Python Module (.py File)"=path "C:/Users/User/Documents/LabVIEW Data/2015 Projects/Combined/2parameter_PE.py") -> ("error out"=w279:errorcluster, "Session ID out"=w276:T4)  [unwired: 9 in]
                n56 = call <vilib>:"Pack.vi"("Argument"=w272, "error in (no error)"=w279, "Session ID"=w276) -> ("error out"=w280:errorcluster, "Python Object References Out"=w278:T5, "Session ID out"=w277:T4)  [unwired: 6 in]
                n57 = call <vilib>:"Call.vi"("Function or Method Name"="onlinePE", "error in (no error)"=w280, "Python Object References In"=w278, "Session ID"=w277) -> ("error out"=w289:errorcluster, "Python Object References Out"=w285:T5, "Session ID out"=w281:T4)  [unwired: 5 in]
                n58 = call-poly <vilib>:"Unpack.vi"("error in (no error)"=w289, "Python Object References In"=w285, "Session ID"=w281) -> ("error out"=w290:errorcluster, "Value"=w270:dbl, "Python Object References Out"=w286:T5, "Session ID out"=w282:T4)  [unwired: 5 in]
                n59 = call-poly <vilib>:"Unpack.vi"("error in (no error)"=w290, "Python Object References In"=w286, "Session ID"=w282) -> ("error out"=w291:errorcluster, "Value"=→"Param 1 2":dbl, "Python Object References Out"=w287:T5, "Session ID out"=w283:T4)  [unwired: 5 in]
                n60 = call-poly <vilib>:"Unpack.vi"("error in (no error)"=w291, "Python Object References In"=w287, "Session ID"=w283) -> ("error out"=w292:errorcluster, "Value"=→"Param 2 2":dbl, "Python Object References Out"=w288:T5, "Session ID out"=w284:T4)  [unwired: 5 in]
                n61 = call-poly <vilib>:"Unpack.vi"("error in (no error)"=w292, "Python Object References In"=w288, "Session ID"=w284) -> ("error out"=w293:errorcluster, "Value"=→"Chi 2":dbl, "Python Object References Out"=w275:T5, "Session ID out"=w274:T4)  [unwired: 5 in]
                n62 = call-poly <vilib>:"Unpack.vi"("error in (no error)"=w293, "Python Object References In"=w275, "Session ID"=w274) -> ("error out"=w265:errorcluster, "Value"=→"Chi ref 2":dbl, "Python Object References Out"=w267:T5, "Session ID out"=w269:T4)  [unwired: 5 in]
                n63 = call-poly <vilib>:"Unpack.vi"("error in (no error)"=w265, "Python Object References In"=w267, "Session ID"=w269) -> ("error out"=w264:errorcluster, "Value"=→"C Int 1 2":dbl, "Python Object References Out"=w266:T5, "Session ID out"=w268:T4)  [unwired: 5 in]
                n64 = call-poly <vilib>:"Unpack.vi"("error in (no error)"=w264, "Python Object References In"=w266, "Session ID"=w268) -> ("error out"=w251:errorcluster, "Value"=→"C Int 2 2":dbl, "Python Object References Out"=w252:T5, "Session ID out"=w253:T4)  [unwired: 5 in]
                n65 = call-poly <vilib>:"Unpack.vi"("error in (no error)"=w251, "Python Object References In"=w252, "Session ID"=w253) -> ("error out"=w256:errorcluster, "Value"=→"t 1 2":dbl, "Python Object References Out"=w255:T5, "Session ID out"=w254:T4)  [unwired: 5 in]
                n66 = call-poly <vilib>:"Unpack.vi"("error in (no error)"=w256, "Python Object References In"=w255, "Session ID"=w254) -> ("error out"=w257:errorcluster, "Value"=→"t 2 2":dbl, "Python Object References Out"=w258:T5, "Session ID out"=w259:T4)  [unwired: 5 in]
                n67 = call-poly <vilib>:"Unpack.vi"("error in (no error)"=w257, "Python Object References In"=w258, "Session ID"=w259) -> ("error out"=w260:errorcluster, "Value"=→"t ref 2":dbl, "Session ID out"=w261:T4)  [unwired: 5 in, 1 out]
                n68 = call <vilib>:"Close Session.vi"("error in (no error)"=w260, "Session ID"=w261) -> ()  [unwired: 9 in, 1 out]
              }
              frame #2 {
                n69 = case shown="True" w298 {
                  tunnel: w302 -> [w306 w342]
                  tunnel: ["Temp 3" w327] -> w301
                  tunnel: ["Flow 3" w326] -> w300
                  tunnel: ["Conc 3" w325] -> w299
                  frame False {
                    n70 = call <vilib>:"New Session.vi"("Path to Python Module (.py File)"=path "C:/Users/User/Documents/LabVIEW Data/2015 Projects/Combined/WriteTFC.py") -> ("error out"=w315:errorcluster, "Session ID out"=w316:T4)  [unwired: 9 in]
                    n71 = call <vilib>:"Pack.vi"("Argument"=w306, "error in (no error)"=w315, "Session ID"=w316) -> ("error out"=w314:errorcluster, "Python Object References Out"=w310:T5, "Session ID out"=w317:T4)  [unwired: 6 in]
                    n72 = call <vilib>:"Pack.vi"("Argument"="Temp 3", "error in (no error)"=w314, "Python Object References In"=w310, "Session ID"=w317) -> ("error out"=w313:errorcluster, "Python Object References Out"=w309:T5, "Session ID out"=w307:T4)  [unwired: 5 in]
                    n73 = call <vilib>:"Pack.vi"("Argument"="Flow 3", "error in (no error)"=w313, "Python Object References In"=w309, "Session ID"=w307) -> ("error out"=w312:errorcluster, "Python Object References Out"=w308:T5, "Session ID out"=w321:T4)  [unwired: 5 in]
                    n74 = call <vilib>:"Pack.vi"("Argument"="Conc 3", "error in (no error)"=w312, "Python Object References In"=w308, "Session ID"=w321) -> ("error out"=w324:errorcluster, "Python Object References Out"=w323:T5, "Session ID out"=w322:T4)  [unwired: 5 in]
                    n75 = call <vilib>:"Call.vi"("Function or Method Name"="AppendResultFile", "error in (no error)"=w324, "Python Object References In"=w323, "Session ID"=w322) -> ("error out"=w311:errorcluster, "Session ID out"=w320:T4)  [unwired: 5 in, 1 out]
                    n76 = call <vilib>:"Close Session.vi"("error in (no error)"=w311, "Session ID"=w320) -> ()  [unwired: 9 in, 1 out]
                  }
                  frame True {
                    n77 = call <vilib>:"New Session.vi"("Path to Python Module (.py File)"=path "C:/Users/User/Documents/LabVIEW Data/2015 Projects/Combined/2parameter_MBDoE.py") -> ("error out"=w343:errorcluster, "Session ID out"=w344:T4)  [unwired: 9 in]
                    n78 = call <vilib>:"Pack.vi"("Argument"=w342, "error in (no error)"=w343, "Session ID"=w344) -> ("error out"=w340:errorcluster, "Python Object References Out"=w339:T5, "Session ID out"=w341:T4)  [unwired: 6 in]
                    n79 = call <vilib>:"Call.vi"("Function or Method Name"="onlineMBDoE", "error in (no error)"=w340, "Python Object References In"=w339, "Session ID"=w341) -> ("error out"=w334:errorcluster, "Python Object References Out"=w330:T5, "Session ID out"=w338:T4)  [unwired: 5 in]
                    n80 = call-poly <vilib>:"Unpack.vi"("error in (no error)"=w334, "Python Object References In"=w330, "Session ID"=w338) -> ("error out"=w333:errorcluster, "Value"=w327:dbl, "Python Object References Out"=w329:T5, "Session ID out"=w337:T4)  [unwired: 5 in]
                    n81 = call-poly <vilib>:"Unpack.vi"("error in (no error)"=w333, "Python Object References In"=w329, "Session ID"=w337) -> ("error out"=w332:errorcluster, "Value"=w326:dbl, "Python Object References Out"=w328:T5, "Session ID out"=w336:T4)  [unwired: 5 in]
                    n82 = call-poly <vilib>:"Unpack.vi"("error in (no error)"=w332, "Python Object References In"=w328, "Session ID"=w336) -> ("error out"=w331:errorcluster, "Value"=w325:dbl, "Session ID out"=w335:T4)  [unwired: 5 in, 1 out]
                    n83 = call <vilib>:"Close Session.vi"("error in (no error)"=w331, "Session ID"=w335) -> ()  [unwired: 9 in, 1 out]
                  }
                }
                "Temp 3" <- w301
                "Flow 3" <- w300
                "Conc 3" <- w299
              }
            }
            "Exp 3" <- TRUE
          }
          frame 5 {
            n84 = flat-sequence {
              tunnel: w354 -> [w362]
              tunnel: w349 -> [w355]
              tunnel: w349 -> [w401]
              tunnel: [w399] -> w348
              tunnel: w349 -> [w431]
              tunnel: [w430] -> w353
              tunnel: [w429] -> w352
              tunnel: [w428] -> w351
              tunnel: w350 -> [w427]
              frame #0 {
                # "make this include a write to record file step"
                n85 = call <vilib>:"New Session.vi"("Path to Python Module (.py File)"=path "C:/Users/User/Documents/LabVIEW Data/2015 Projects/Combined/HPLCandAppend.py") -> ("error out"=w373:errorcluster, "Session ID out"=w372:T4)  [unwired: 9 in]
                n86 = call <vilib>:"Pack.vi"("Argument"=w362, "error in (no error)"=w373, "Session ID"=w372) -> ("error out"=w357:errorcluster, "Python Object References Out"=w359:T5, "Session ID out"=w361:T4)  [unwired: 6 in]
                n87 = call <vilib>:"Pack.vi"("Argument"=w355, "error in (no error)"=w357, "Python Object References In"=w359, "Session ID"=w361) -> ("error out"=w356:errorcluster, "Python Object References Out"=w358:T5, "Session ID out"=w360:T4)  [unwired: 5 in]
                n88 = call <vilib>:"Call.vi"("Function or Method Name"="HPLC", "error in (no error)"=w356, "Python Object References In"=w358, "Session ID"=w360) -> ("error out"=w374:errorcluster, "Python Object References Out"=w365:T5, "Session ID out"=w366:T4)  [unwired: 5 in]
                n89 = call-poly <vilib>:"Unpack.vi"("error in (no error)"=w374, "Python Object References In"=w365, "Session ID"=w366) -> ("error out"=w375:errorcluster, "Value"=→"C BAcid 3":dbl, "Python Object References Out"=w370:T5, "Session ID out"=w369:T4)  [unwired: 5 in]
                n90 = call-poly <vilib>:"Unpack.vi"("error in (no error)"=w375, "Python Object References In"=w370, "Session ID"=w369) -> ("error out"=w376:errorcluster, "Value"=→"C EB 3":dbl, "Session ID out"=w371:T4)  [unwired: 5 in, 1 out]
                n91 = call <vilib>:"Close Session.vi"("error in (no error)"=w376, "Session ID"=w371) -> ()  [unwired: 9 in, 1 out]
              }
              frame #1 {
                # "make this include a write to record file step"
                n92 = call <vilib>:"New Session.vi"("Path to Python Module (.py File)"=path "C:/Users/User/Documents/LabVIEW Data/2015 Projects/Combined/2parameter_PE.py") -> ("error out"=w408:errorcluster, "Session ID out"=w405:T4)  [unwired: 9 in]
                n93 = call <vilib>:"Pack.vi"("Argument"=w401, "error in (no error)"=w408, "Session ID"=w405) -> ("error out"=w409:errorcluster, "Python Object References Out"=w407:T5, "Session ID out"=w406:T4)  [unwired: 6 in]
                n94 = call <vilib>:"Call.vi"("Function or Method Name"="onlinePE", "error in (no error)"=w409, "Python Object References In"=w407, "Session ID"=w406) -> ("error out"=w418:errorcluster, "Python Object References Out"=w414:T5, "Session ID out"=w410:T4)  [unwired: 5 in]
                n95 = call-poly <vilib>:"Unpack.vi"("error in (no error)"=w418, "Python Object References In"=w414, "Session ID"=w410) -> ("error out"=w419:errorcluster, "Value"=w399:dbl, "Python Object References Out"=w415:T5, "Session ID out"=w411:T4)  [unwired: 5 in]
                n96 = call-poly <vilib>:"Unpack.vi"("error in (no error)"=w419, "Python Object References In"=w415, "Session ID"=w411) -> ("error out"=w420:errorcluster, "Value"=→"Param 1 3":dbl, "Python Object References Out"=w416:T5, "Session ID out"=w412:T4)  [unwired: 5 in]
                n97 = call-poly <vilib>:"Unpack.vi"("error in (no error)"=w420, "Python Object References In"=w416, "Session ID"=w412) -> ("error out"=w421:errorcluster, "Value"=→"Param 2 3":dbl, "Python Object References Out"=w417:T5, "Session ID out"=w413:T4)  [unwired: 5 in]
                n98 = call-poly <vilib>:"Unpack.vi"("error in (no error)"=w421, "Python Object References In"=w417, "Session ID"=w413) -> ("error out"=w422:errorcluster, "Value"=→"Chi  3":dbl, "Python Object References Out"=w404:T5, "Session ID out"=w403:T4)  [unwired: 5 in]
                n99 = call-poly <vilib>:"Unpack.vi"("error in (no error)"=w422, "Python Object References In"=w404, "Session ID"=w403) -> ("error out"=w394:errorcluster, "Value"=→"Chi ref 3":dbl, "Python Object References Out"=w396:T5, "Session ID out"=w398:T4)  [unwired: 5 in]
                n100 = call-poly <vilib>:"Unpack.vi"("error in (no error)"=w394, "Python Object References In"=w396, "Session ID"=w398) -> ("error out"=w393:errorcluster, "Value"=→"C Int 1 3":dbl, "Python Object References Out"=w395:T5, "Session ID out"=w397:T4)  [unwired: 5 in]
                n101 = call-poly <vilib>:"Unpack.vi"("error in (no error)"=w393, "Python Object References In"=w395, "Session ID"=w397) -> ("error out"=w379:errorcluster, "Value"=→"C Int 2 3":dbl, "Python Object References Out"=w380:T5, "Session ID out"=w381:T4)  [unwired: 5 in]
                n102 = call-poly <vilib>:"Unpack.vi"("error in (no error)"=w379, "Python Object References In"=w380, "Session ID"=w381) -> ("error out"=w385:errorcluster, "Value"=→"t 1 3":dbl, "Python Object References Out"=w384:T5, "Session ID out"=w383:T4)  [unwired: 5 in]
                n103 = call-poly <vilib>:"Unpack.vi"("error in (no error)"=w385, "Python Object References In"=w384, "Session ID"=w383) -> ("error out"=w386:errorcluster, "Value"=→"t 2 3":dbl, "Python Object References Out"=w387:T5, "Session ID out"=w388:T4)  [unwired: 5 in]
                n104 = call-poly <vilib>:"Unpack.vi"("error in (no error)"=w386, "Python Object References In"=w387, "Session ID"=w388) -> ("error out"=w389:errorcluster, "Value"=→"t ref 3":dbl, "Session ID out"=w390:T4)  [unwired: 5 in, 1 out]
                n105 = call <vilib>:"Close Session.vi"("error in (no error)"=w389, "Session ID"=w390) -> ()  [unwired: 9 in, 1 out]
              }
              frame #2 {
                n106 = case shown="True" w427 {
                  tunnel: w431 -> [w435 w471]
                  tunnel: ["Temp 4" w456] -> w430
                  tunnel: ["Flow 4" w455] -> w429
                  tunnel: ["Conc 4" w454] -> w428
                  frame False {
                    n107 = call <vilib>:"New Session.vi"("Path to Python Module (.py File)"=path "C:/Users/User/Documents/LabVIEW Data/2015 Projects/Combined/WriteTFC.py") -> ("error out"=w444:errorcluster, "Session ID out"=w445:T4)  [unwired: 9 in]
                    n108 = call <vilib>:"Pack.vi"("Argument"=w435, "error in (no error)"=w444, "Session ID"=w445) -> ("error out"=w443:errorcluster, "Python Object References Out"=w439:T5, "Session ID out"=w446:T4)  [unwired: 6 in]
                    n109 = call <vilib>:"Pack.vi"("Argument"="Temp 4", "error in (no error)"=w443, "Python Object References In"=w439, "Session ID"=w446) -> ("error out"=w442:errorcluster, "Python Object References Out"=w438:T5, "Session ID out"=w436:T4)  [unwired: 5 in]
                    n110 = call <vilib>:"Pack.vi"("Argument"="Flow 4", "error in (no error)"=w442, "Python Object References In"=w438, "Session ID"=w436) -> ("error out"=w441:errorcluster, "Python Object References Out"=w437:T5, "Session ID out"=w450:T4)  [unwired: 5 in]
                    n111 = call <vilib>:"Pack.vi"("Argument"="Conc 4", "error in (no error)"=w441, "Python Object References In"=w437, "Session ID"=w450) -> ("error out"=w453:errorcluster, "Python Object References Out"=w452:T5, "Session ID out"=w451:T4)  [unwired: 5 in]
                    n112 = call <vilib>:"Call.vi"("Function or Method Name"="AppendResultFile", "error in (no error)"=w453, "Python Object References In"=w452, "Session ID"=w451) -> ("error out"=w440:errorcluster, "Session ID out"=w449:T4)  [unwired: 5 in, 1 out]
                    n113 = call <vilib>:"Close Session.vi"("error in (no error)"=w440, "Session ID"=w449) -> ()  [unwired: 9 in, 1 out]
                  }
                  frame True {
                    n114 = call <vilib>:"New Session.vi"("Path to Python Module (.py File)"=path "C:/Users/User/Documents/LabVIEW Data/2015 Projects/Combined/2parameter_MBDoE.py") -> ("error out"=w472:errorcluster, "Session ID out"=w473:T4)  [unwired: 9 in]
                    n115 = call <vilib>:"Pack.vi"("Argument"=w471, "error in (no error)"=w472, "Session ID"=w473) -> ("error out"=w469:errorcluster, "Python Object References Out"=w468:T5, "Session ID out"=w470:T4)  [unwired: 6 in]
                    n116 = call <vilib>:"Call.vi"("Function or Method Name"="onlineMBDoE", "error in (no error)"=w469, "Python Object References In"=w468, "Session ID"=w470) -> ("error out"=w463:errorcluster, "Python Object References Out"=w459:T5, "Session ID out"=w467:T4)  [unwired: 5 in]
                    n117 = call-poly <vilib>:"Unpack.vi"("error in (no error)"=w463, "Python Object References In"=w459, "Session ID"=w467) -> ("error out"=w462:errorcluster, "Value"=w456:dbl, "Python Object References Out"=w458:T5, "Session ID out"=w466:T4)  [unwired: 5 in]
                    n118 = call-poly <vilib>:"Unpack.vi"("error in (no error)"=w462, "Python Object References In"=w458, "Session ID"=w466) -> ("error out"=w461:errorcluster, "Value"=w455:dbl, "Python Object References Out"=w457:T5, "Session ID out"=w465:T4)  [unwired: 5 in]
                    n119 = call-poly <vilib>:"Unpack.vi"("error in (no error)"=w461, "Python Object References In"=w457, "Session ID"=w465) -> ("error out"=w460:errorcluster, "Value"=w454:dbl, "Session ID out"=w464:T4)  [unwired: 5 in, 1 out]
                    n120 = call <vilib>:"Close Session.vi"("error in (no error)"=w460, "Session ID"=w464) -> ()  [unwired: 9 in, 1 out]
                  }
                }
                "Temp 4" <- w430
                "Flow 4" <- w429
                "Conc 4" <- w428
              }
            }
            "Exp 4" <- TRUE
          }
          frame 6 {
            n121 = flat-sequence {
              tunnel: w483 -> [w491]
              tunnel: w478 -> [w484]
              tunnel: w478 -> [w530]
              tunnel: [w528] -> w477
              tunnel: w478 -> [w560]
              tunnel: [w559] -> w482
              tunnel: [w558] -> w481
              tunnel: [w557] -> w480
              tunnel: w479 -> [w556]
              frame #0 {
                # "make this include a write to record file step"
                n122 = call <vilib>:"New Session.vi"("Path to Python Module (.py File)"=path "C:/Users/User/Documents/LabVIEW Data/2015 Projects/Combined/HPLCandAppend.py") -> ("error out"=w502:errorcluster, "Session ID out"=w501:T4)  [unwired: 9 in]
                n123 = call <vilib>:"Pack.vi"("Argument"=w491, "error in (no error)"=w502, "Session ID"=w501) -> ("error out"=w488:errorcluster, "Python Object References Out"=w489:T5, "Session ID out"=w490:T4)  [unwired: 6 in]
                n124 = call <vilib>:"Pack.vi"("Argument"=w484, "error in (no error)"=w488, "Python Object References In"=w489, "Session ID"=w490) -> ("error out"=w487:errorcluster, "Python Object References Out"=w486:T5, "Session ID out"=w485:T4)  [unwired: 5 in]
                n125 = call <vilib>:"Call.vi"("Function or Method Name"="HPLC", "error in (no error)"=w487, "Python Object References In"=w486, "Session ID"=w485) -> ("error out"=w503:errorcluster, "Python Object References Out"=w494:T5, "Session ID out"=w495:T4)  [unwired: 5 in]
                n126 = call-poly <vilib>:"Unpack.vi"("error in (no error)"=w503, "Python Object References In"=w494, "Session ID"=w495) -> ("error out"=w504:errorcluster, "Value"=→"C BAcid 4":dbl, "Python Object References Out"=w499:T5, "Session ID out"=w498:T4)  [unwired: 5 in]
                n127 = call-poly <vilib>:"Unpack.vi"("error in (no error)"=w504, "Python Object References In"=w499, "Session ID"=w498) -> ("error out"=w505:errorcluster, "Value"=→"C EB 4":dbl, "Session ID out"=w500:T4)  [unwired: 5 in, 1 out]
                n128 = call <vilib>:"Close Session.vi"("error in (no error)"=w505, "Session ID"=w500) -> ()  [unwired: 9 in, 1 out]
              }
              frame #1 {
                # "make this include a write to record file step"
                n129 = call <vilib>:"New Session.vi"("Path to Python Module (.py File)"=path "C:/Users/User/Documents/LabVIEW Data/2015 Projects/Combined/2parameter_PE.py") -> ("error out"=w537:errorcluster, "Session ID out"=w534:T4)  [unwired: 9 in]
                n130 = call <vilib>:"Pack.vi"("Argument"=w530, "error in (no error)"=w537, "Session ID"=w534) -> ("error out"=w538:errorcluster, "Python Object References Out"=w536:T5, "Session ID out"=w535:T4)  [unwired: 6 in]
                n131 = call <vilib>:"Call.vi"("Function or Method Name"="onlinePE", "error in (no error)"=w538, "Python Object References In"=w536, "Session ID"=w535) -> ("error out"=w547:errorcluster, "Python Object References Out"=w543:T5, "Session ID out"=w539:T4)  [unwired: 5 in]
                n132 = call-poly <vilib>:"Unpack.vi"("error in (no error)"=w547, "Python Object References In"=w543, "Session ID"=w539) -> ("error out"=w548:errorcluster, "Value"=w528:dbl, "Python Object References Out"=w544:T5, "Session ID out"=w540:T4)  [unwired: 5 in]
                n133 = call-poly <vilib>:"Unpack.vi"("error in (no error)"=w548, "Python Object References In"=w544, "Session ID"=w540) -> ("error out"=w549:errorcluster, "Value"=→"Param 1 4":dbl, "Python Object References Out"=w545:T5, "Session ID out"=w541:T4)  [unwired: 5 in]
                n134 = call-poly <vilib>:"Unpack.vi"("error in (no error)"=w549, "Python Object References In"=w545, "Session ID"=w541) -> ("error out"=w550:errorcluster, "Value"=→"Param 2 4":dbl, "Python Object References Out"=w546:T5, "Session ID out"=w542:T4)  [unwired: 5 in]
                n135 = call-poly <vilib>:"Unpack.vi"("error in (no error)"=w550, "Python Object References In"=w546, "Session ID"=w542) -> ("error out"=w551:errorcluster, "Value"=→"Chi  4":dbl, "Python Object References Out"=w533:T5, "Session ID out"=w532:T4)  [unwired: 5 in]
                n136 = call-poly <vilib>:"Unpack.vi"("error in (no error)"=w551, "Python Object References In"=w533, "Session ID"=w532) -> ("error out"=w523:errorcluster, "Value"=→"Chi ref 4":dbl, "Python Object References Out"=w525:T5, "Session ID out"=w527:T4)  [unwired: 5 in]
                n137 = call-poly <vilib>:"Unpack.vi"("error in (no error)"=w523, "Python Object References In"=w525, "Session ID"=w527) -> ("error out"=w522:errorcluster, "Value"=→"C Int 1 4":dbl, "Python Object References Out"=w524:T5, "Session ID out"=w526:T4)  [unwired: 5 in]
                n138 = call-poly <vilib>:"Unpack.vi"("error in (no error)"=w522, "Python Object References In"=w524, "Session ID"=w526) -> ("error out"=w508:errorcluster, "Value"=→"C Int 2 4":dbl, "Python Object References Out"=w509:T5, "Session ID out"=w510:T4)  [unwired: 5 in]
                n139 = call-poly <vilib>:"Unpack.vi"("error in (no error)"=w508, "Python Object References In"=w509, "Session ID"=w510) -> ("error out"=w514:errorcluster, "Value"=→"t 1 4":dbl, "Python Object References Out"=w513:T5, "Session ID out"=w512:T4)  [unwired: 5 in]
                n140 = call-poly <vilib>:"Unpack.vi"("error in (no error)"=w514, "Python Object References In"=w513, "Session ID"=w512) -> ("error out"=w515:errorcluster, "Value"=→"t 2 4":dbl, "Python Object References Out"=w516:T5, "Session ID out"=w517:T4)  [unwired: 5 in]
                n141 = call-poly <vilib>:"Unpack.vi"("error in (no error)"=w515, "Python Object References In"=w516, "Session ID"=w517) -> ("error out"=w518:errorcluster, "Value"=→"t ref 4":dbl, "Session ID out"=w519:T4)  [unwired: 5 in, 1 out]
                n142 = call <vilib>:"Close Session.vi"("error in (no error)"=w518, "Session ID"=w519) -> ()  [unwired: 9 in, 1 out]
              }
              frame #2 {
                n143 = case shown="True" w556 {
                  tunnel: w560 -> [w564 w600]
                  tunnel: ["Temp 5" w585] -> w559
                  tunnel: ["Flow 5" w584] -> w558
                  tunnel: ["Conc 5" w583] -> w557
                  frame False {
                    n144 = call <vilib>:"New Session.vi"("Path to Python Module (.py File)"=path "C:/Users/User/Documents/LabVIEW Data/2015 Projects/Combined/WriteTFC.py") -> ("error out"=w573:errorcluster, "Session ID out"=w574:T4)  [unwired: 9 in]
                    n145 = call <vilib>:"Pack.vi"("Argument"=w564, "error in (no error)"=w573, "Session ID"=w574) -> ("error out"=w572:errorcluster, "Python Object References Out"=w568:T5, "Session ID out"=w575:T4)  [unwired: 6 in]
                    n146 = call <vilib>:"Pack.vi"("Argument"="Temp 5", "error in (no error)"=w572, "Python Object References In"=w568, "Session ID"=w575) -> ("error out"=w571:errorcluster, "Python Object References Out"=w567:T5, "Session ID out"=w565:T4)  [unwired: 5 in]
                    n147 = call <vilib>:"Pack.vi"("Argument"="Flow 5", "error in (no error)"=w571, "Python Object References In"=w567, "Session ID"=w565) -> ("error out"=w570:errorcluster, "Python Object References Out"=w566:T5, "Session ID out"=w579:T4)  [unwired: 5 in]
                    n148 = call <vilib>:"Pack.vi"("Argument"="Conc 5", "error in (no error)"=w570, "Python Object References In"=w566, "Session ID"=w579) -> ("error out"=w582:errorcluster, "Python Object References Out"=w581:T5, "Session ID out"=w580:T4)  [unwired: 5 in]
                    n149 = call <vilib>:"Call.vi"("Function or Method Name"="AppendResultFile", "error in (no error)"=w582, "Python Object References In"=w581, "Session ID"=w580) -> ("error out"=w569:errorcluster, "Session ID out"=w578:T4)  [unwired: 5 in, 1 out]
                    n150 = call <vilib>:"Close Session.vi"("error in (no error)"=w569, "Session ID"=w578) -> ()  [unwired: 9 in, 1 out]
                  }
                  frame True {
                    n151 = call <vilib>:"New Session.vi"("Path to Python Module (.py File)"=path "C:/Users/User/Documents/LabVIEW Data/2015 Projects/Combined/2parameter_MBDoE.py") -> ("error out"=w601:errorcluster, "Session ID out"=w602:T4)  [unwired: 9 in]
                    n152 = call <vilib>:"Pack.vi"("Argument"=w600, "error in (no error)"=w601, "Session ID"=w602) -> ("error out"=w598:errorcluster, "Python Object References Out"=w597:T5, "Session ID out"=w599:T4)  [unwired: 6 in]
                    n153 = call <vilib>:"Call.vi"("Function or Method Name"="onlineMBDoE", "error in (no error)"=w598, "Python Object References In"=w597, "Session ID"=w599) -> ("error out"=w592:errorcluster, "Python Object References Out"=w588:T5, "Session ID out"=w596:T4)  [unwired: 5 in]
                    n154 = call-poly <vilib>:"Unpack.vi"("error in (no error)"=w592, "Python Object References In"=w588, "Session ID"=w596) -> ("error out"=w591:errorcluster, "Value"=w585:dbl, "Python Object References Out"=w587:T5, "Session ID out"=w595:T4)  [unwired: 5 in]
                    n155 = call-poly <vilib>:"Unpack.vi"("error in (no error)"=w591, "Python Object References In"=w587, "Session ID"=w595) -> ("error out"=w590:errorcluster, "Value"=w584:dbl, "Python Object References Out"=w586:T5, "Session ID out"=w594:T4)  [unwired: 5 in]
                    n156 = call-poly <vilib>:"Unpack.vi"("error in (no error)"=w590, "Python Object References In"=w586, "Session ID"=w594) -> ("error out"=w589:errorcluster, "Value"=w583:dbl, "Session ID out"=w593:T4)  [unwired: 5 in, 1 out]
                    n157 = call <vilib>:"Close Session.vi"("error in (no error)"=w589, "Session ID"=w593) -> ()  [unwired: 9 in, 1 out]
                  }
                }
                "Temp 5" <- w559
                "Flow 5" <- w558
                "Conc 5" <- w557
              }
            }
            "Exp 5" <- TRUE
          }
          frame 7 {
            n158 = flat-sequence {
              tunnel: w612 -> [w620]
              tunnel: w607 -> [w613]
              tunnel: w607 -> [w659]
              tunnel: [w657] -> w606
              tunnel: w607 -> [w689]
              tunnel: [w688] -> w611
              tunnel: [w687] -> w610
              tunnel: [w686] -> w609
              tunnel: w608 -> [w685]
              frame #0 {
                # "make this include a write to record file step"
                n159 = call <vilib>:"New Session.vi"("Path to Python Module (.py File)"=path "C:/Users/User/Documents/LabVIEW Data/2015 Projects/Combined/HPLCandAppend.py") -> ("error out"=w631:errorcluster, "Session ID out"=w630:T4)  [unwired: 9 in]
                n160 = call <vilib>:"Pack.vi"("Argument"=w620, "error in (no error)"=w631, "Session ID"=w630) -> ("error out"=w617:errorcluster, "Python Object References Out"=w618:T5, "Session ID out"=w619:T4)  [unwired: 6 in]
                n161 = call <vilib>:"Pack.vi"("Argument"=w613, "error in (no error)"=w617, "Python Object References In"=w618, "Session ID"=w619) -> ("error out"=w614:errorcluster, "Python Object References Out"=w615:T5, "Session ID out"=w616:T4)  [unwired: 5 in]
                n162 = call <vilib>:"Call.vi"("Function or Method Name"="HPLC", "error in (no error)"=w614, "Python Object References In"=w615, "Session ID"=w616) -> ("error out"=w632:errorcluster, "Python Object References Out"=w623:T5, "Session ID out"=w624:T4)  [unwired: 5 in]
                n163 = call-poly <vilib>:"Unpack.vi"("error in (no error)"=w632, "Python Object References In"=w623, "Session ID"=w624) -> ("error out"=w633:errorcluster, "Value"=→"C BAcid 5":dbl, "Python Object References Out"=w628:T5, "Session ID out"=w627:T4)  [unwired: 5 in]
                n164 = call-poly <vilib>:"Unpack.vi"("error in (no error)"=w633, "Python Object References In"=w628, "Session ID"=w627) -> ("error out"=w634:errorcluster, "Value"=→"C EB 5":dbl, "Session ID out"=w629:T4)  [unwired: 5 in, 1 out]
                n165 = call <vilib>:"Close Session.vi"("error in (no error)"=w634, "Session ID"=w629) -> ()  [unwired: 9 in, 1 out]
              }
              frame #1 {
                # "make this include a write to record file step"
                n166 = call <vilib>:"New Session.vi"("Path to Python Module (.py File)"=path "C:/Users/User/Documents/LabVIEW Data/2015 Projects/Combined/2parameter_PE.py") -> ("error out"=w666:errorcluster, "Session ID out"=w663:T4)  [unwired: 9 in]
                n167 = call <vilib>:"Pack.vi"("Argument"=w659, "error in (no error)"=w666, "Session ID"=w663) -> ("error out"=w667:errorcluster, "Python Object References Out"=w665:T5, "Session ID out"=w664:T4)  [unwired: 6 in]
                n168 = call <vilib>:"Call.vi"("Function or Method Name"="onlinePE", "error in (no error)"=w667, "Python Object References In"=w665, "Session ID"=w664) -> ("error out"=w676:errorcluster, "Python Object References Out"=w672:T5, "Session ID out"=w668:T4)  [unwired: 5 in]
                n169 = call-poly <vilib>:"Unpack.vi"("error in (no error)"=w676, "Python Object References In"=w672, "Session ID"=w668) -> ("error out"=w677:errorcluster, "Value"=w657:dbl, "Python Object References Out"=w673:T5, "Session ID out"=w669:T4)  [unwired: 5 in]
                n170 = call-poly <vilib>:"Unpack.vi"("error in (no error)"=w677, "Python Object References In"=w673, "Session ID"=w669) -> ("error out"=w678:errorcluster, "Value"=→"Param 1 5":dbl, "Python Object References Out"=w674:T5, "Session ID out"=w670:T4)  [unwired: 5 in]
                n171 = call-poly <vilib>:"Unpack.vi"("error in (no error)"=w678, "Python Object References In"=w674, "Session ID"=w670) -> ("error out"=w679:errorcluster, "Value"=→"Param 2 5":dbl, "Python Object References Out"=w675:T5, "Session ID out"=w671:T4)  [unwired: 5 in]
                n172 = call-poly <vilib>:"Unpack.vi"("error in (no error)"=w679, "Python Object References In"=w675, "Session ID"=w671) -> ("error out"=w680:errorcluster, "Value"=→"Chi  5":dbl, "Python Object References Out"=w662:T5, "Session ID out"=w661:T4)  [unwired: 5 in]
                n173 = call-poly <vilib>:"Unpack.vi"("error in (no error)"=w680, "Python Object References In"=w662, "Session ID"=w661) -> ("error out"=w652:errorcluster, "Value"=→"Chi ref 5":dbl, "Python Object References Out"=w654:T5, "Session ID out"=w656:T4)  [unwired: 5 in]
                n174 = call-poly <vilib>:"Unpack.vi"("error in (no error)"=w652, "Python Object References In"=w654, "Session ID"=w656) -> ("error out"=w651:errorcluster, "Value"=→"C Int 1 5":dbl, "Python Object References Out"=w653:T5, "Session ID out"=w655:T4)  [unwired: 5 in]
                n175 = call-poly <vilib>:"Unpack.vi"("error in (no error)"=w651, "Python Object References In"=w653, "Session ID"=w655) -> ("error out"=w637:errorcluster, "Value"=→"C Int 2 5":dbl, "Python Object References Out"=w638:T5, "Session ID out"=w639:T4)  [unwired: 5 in]
                n176 = call-poly <vilib>:"Unpack.vi"("error in (no error)"=w637, "Python Object References In"=w638, "Session ID"=w639) -> ("error out"=w643:errorcluster, "Value"=→"t 1 5":dbl, "Python Object References Out"=w642:T5, "Session ID out"=w641:T4)  [unwired: 5 in]
                n177 = call-poly <vilib>:"Unpack.vi"("error in (no error)"=w643, "Python Object References In"=w642, "Session ID"=w641) -> ("error out"=w644:errorcluster, "Value"=→"t 2 5":dbl, "Python Object References Out"=w645:T5, "Session ID out"=w646:T4)  [unwired: 5 in]
                n178 = call-poly <vilib>:"Unpack.vi"("error in (no error)"=w644, "Python Object References In"=w645, "Session ID"=w646) -> ("error out"=w647:errorcluster, "Value"=→"t ref 5":dbl, "Session ID out"=w648:T4)  [unwired: 5 in, 1 out]
                n179 = call <vilib>:"Close Session.vi"("error in (no error)"=w647, "Session ID"=w648) -> ()  [unwired: 9 in, 1 out]
              }
              frame #2 {
                n180 = case shown="True" w685 {
                  tunnel: w689 -> [w693 w729]
                  tunnel: ["Temp 6" w714] -> w688
                  tunnel: ["Flow 6" w713] -> w687
                  tunnel: ["Conc 6" w712] -> w686
                  frame False {
                    n181 = call <vilib>:"New Session.vi"("Path to Python Module (.py File)"=path "C:/Users/User/Documents/LabVIEW Data/2015 Projects/Combined/WriteTFC.py") -> ("error out"=w702:errorcluster, "Session ID out"=w703:T4)  [unwired: 9 in]
                    n182 = call <vilib>:"Pack.vi"("Argument"=w693, "error in (no error)"=w702, "Session ID"=w703) -> ("error out"=w701:errorcluster, "Python Object References Out"=w697:T5, "Session ID out"=w704:T4)  [unwired: 6 in]
                    n183 = call <vilib>:"Pack.vi"("Argument"="Temp 6", "error in (no error)"=w701, "Python Object References In"=w697, "Session ID"=w704) -> ("error out"=w700:errorcluster, "Python Object References Out"=w696:T5, "Session ID out"=w694:T4)  [unwired: 5 in]
                    n184 = call <vilib>:"Pack.vi"("Argument"="Flow 6", "error in (no error)"=w700, "Python Object References In"=w696, "Session ID"=w694) -> ("error out"=w699:errorcluster, "Python Object References Out"=w695:T5, "Session ID out"=w708:T4)  [unwired: 5 in]
                    n185 = call <vilib>:"Pack.vi"("Argument"="Conc 6", "error in (no error)"=w699, "Python Object References In"=w695, "Session ID"=w708) -> ("error out"=w711:errorcluster, "Python Object References Out"=w710:T5, "Session ID out"=w709:T4)  [unwired: 5 in]
                    n186 = call <vilib>:"Call.vi"("Function or Method Name"="AppendResultFile", "error in (no error)"=w711, "Python Object References In"=w710, "Session ID"=w709) -> ("error out"=w698:errorcluster, "Session ID out"=w707:T4)  [unwired: 5 in, 1 out]
                    n187 = call <vilib>:"Close Session.vi"("error in (no error)"=w698, "Session ID"=w707) -> ()  [unwired: 9 in, 1 out]
                  }
                  frame True {
                    n188 = call <vilib>:"New Session.vi"("Path to Python Module (.py File)"=path "C:/Users/User/Documents/LabVIEW Data/2015 Projects/Combined/2parameter_MBDoE.py") -> ("error out"=w730:errorcluster, "Session ID out"=w731:T4)  [unwired: 9 in]
                    n189 = call <vilib>:"Pack.vi"("Argument"=w729, "error in (no error)"=w730, "Session ID"=w731) -> ("error out"=w727:errorcluster, "Python Object References Out"=w726:T5, "Session ID out"=w728:T4)  [unwired: 6 in]
                    n190 = call <vilib>:"Call.vi"("Function or Method Name"="onlineMBDoE", "error in (no error)"=w727, "Python Object References In"=w726, "Session ID"=w728) -> ("error out"=w721:errorcluster, "Python Object References Out"=w717:T5, "Session ID out"=w725:T4)  [unwired: 5 in]
                    n191 = call-poly <vilib>:"Unpack.vi"("error in (no error)"=w721, "Python Object References In"=w717, "Session ID"=w725) -> ("error out"=w720:errorcluster, "Value"=w714:dbl, "Python Object References Out"=w716:T5, "Session ID out"=w724:T4)  [unwired: 5 in]
                    n192 = call-poly <vilib>:"Unpack.vi"("error in (no error)"=w720, "Python Object References In"=w716, "Session ID"=w724) -> ("error out"=w719:errorcluster, "Value"=w713:dbl, "Python Object References Out"=w715:T5, "Session ID out"=w723:T4)  [unwired: 5 in]
                    n193 = call-poly <vilib>:"Unpack.vi"("error in (no error)"=w719, "Python Object References In"=w715, "Session ID"=w723) -> ("error out"=w718:errorcluster, "Value"=w712:dbl, "Session ID out"=w722:T4)  [unwired: 5 in, 1 out]
                    n194 = call <vilib>:"Close Session.vi"("error in (no error)"=w718, "Session ID"=w722) -> ()  [unwired: 9 in, 1 out]
                  }
                }
                "Temp 6" <- w688
                "Flow 6" <- w687
                "Conc 6" <- w686
              }
            }
            "Exp 6" <- TRUE
          }
          frame 8 {
            n195 = flat-sequence {
              tunnel: w741 -> [w749]
              tunnel: w736 -> [w742]
              tunnel: w736 -> [w788]
              tunnel: [w786] -> w735
              tunnel: w736 -> [w818]
              tunnel: [w817] -> w740
              tunnel: [w816] -> w739
              tunnel: [w815] -> w738
              tunnel: w737 -> [w814]
              frame #0 {
                # "make this include a write to record file step"
                n196 = call <vilib>:"New Session.vi"("Path to Python Module (.py File)"=path "C:/Users/User/Documents/LabVIEW Data/2015 Projects/Combined/HPLCandAppend.py") -> ("error out"=w760:errorcluster, "Session ID out"=w759:T4)  [unwired: 9 in]
                n197 = call <vilib>:"Pack.vi"("Argument"=w749, "error in (no error)"=w760, "Session ID"=w759) -> ("error out"=w744:errorcluster, "Python Object References Out"=w746:T5, "Session ID out"=w748:T4)  [unwired: 6 in]
                n198 = call <vilib>:"Pack.vi"("Argument"=w742, "error in (no error)"=w744, "Python Object References In"=w746, "Session ID"=w748) -> ("error out"=w743:errorcluster, "Python Object References Out"=w745:T5, "Session ID out"=w747:T4)  [unwired: 5 in]
                n199 = call <vilib>:"Call.vi"("Function or Method Name"="HPLC", "error in (no error)"=w743, "Python Object References In"=w745, "Session ID"=w747) -> ("error out"=w761:errorcluster, "Python Object References Out"=w752:T5, "Session ID out"=w753:T4)  [unwired: 5 in]
                n200 = call-poly <vilib>:"Unpack.vi"("error in (no error)"=w761, "Python Object References In"=w752, "Session ID"=w753) -> ("error out"=w762:errorcluster, "Value"=→"C BAcid 6":dbl, "Python Object References Out"=w757:T5, "Session ID out"=w756:T4)  [unwired: 5 in]
                n201 = call-poly <vilib>:"Unpack.vi"("error in (no error)"=w762, "Python Object References In"=w757, "Session ID"=w756) -> ("error out"=w763:errorcluster, "Value"=→"C EB 6":dbl, "Session ID out"=w758:T4)  [unwired: 5 in, 1 out]
                n202 = call <vilib>:"Close Session.vi"("error in (no error)"=w763, "Session ID"=w758) -> ()  [unwired: 9 in, 1 out]
              }
              frame #1 {
                # "make this include a write to record file step"
                n203 = call <vilib>:"New Session.vi"("Path to Python Module (.py File)"=path "C:/Users/User/Documents/LabVIEW Data/2015 Projects/Combined/2parameter_PE.py") -> ("error out"=w795:errorcluster, "Session ID out"=w792:T4)  [unwired: 9 in]
                n204 = call <vilib>:"Pack.vi"("Argument"=w788, "error in (no error)"=w795, "Session ID"=w792) -> ("error out"=w796:errorcluster, "Python Object References Out"=w794:T5, "Session ID out"=w793:T4)  [unwired: 6 in]
                n205 = call <vilib>:"Call.vi"("Function or Method Name"="onlinePE", "error in (no error)"=w796, "Python Object References In"=w794, "Session ID"=w793) -> ("error out"=w805:errorcluster, "Python Object References Out"=w801:T5, "Session ID out"=w797:T4)  [unwired: 5 in]
                n206 = call-poly <vilib>:"Unpack.vi"("error in (no error)"=w805, "Python Object References In"=w801, "Session ID"=w797) -> ("error out"=w806:errorcluster, "Value"=w786:dbl, "Python Object References Out"=w802:T5, "Session ID out"=w798:T4)  [unwired: 5 in]
                n207 = call-poly <vilib>:"Unpack.vi"("error in (no error)"=w806, "Python Object References In"=w802, "Session ID"=w798) -> ("error out"=w807:errorcluster, "Value"=→"Param 1 6":dbl, "Python Object References Out"=w803:T5, "Session ID out"=w799:T4)  [unwired: 5 in]
                n208 = call-poly <vilib>:"Unpack.vi"("error in (no error)"=w807, "Python Object References In"=w803, "Session ID"=w799) -> ("error out"=w808:errorcluster, "Value"=→"Param 2 6":dbl, "Python Object References Out"=w804:T5, "Session ID out"=w800:T4)  [unwired: 5 in]
                n209 = call-poly <vilib>:"Unpack.vi"("error in (no error)"=w808, "Python Object References In"=w804, "Session ID"=w800) -> ("error out"=w809:errorcluster, "Value"=→"Chi  6":dbl, "Python Object References Out"=w791:T5, "Session ID out"=w790:T4)  [unwired: 5 in]
                n210 = call-poly <vilib>:"Unpack.vi"("error in (no error)"=w809, "Python Object References In"=w791, "Session ID"=w790) -> ("error out"=w781:errorcluster, "Value"=→"Chi ref 6":dbl, "Python Object References Out"=w783:T5, "Session ID out"=w785:T4)  [unwired: 5 in]
                n211 = call-poly <vilib>:"Unpack.vi"("error in (no error)"=w781, "Python Object References In"=w783, "Session ID"=w785) -> ("error out"=w780:errorcluster, "Value"=→"C Int 1 6":dbl, "Python Object References Out"=w782:T5, "Session ID out"=w784:T4)  [unwired: 5 in]
                n212 = call-poly <vilib>:"Unpack.vi"("error in (no error)"=w780, "Python Object References In"=w782, "Session ID"=w784) -> ("error out"=w766:errorcluster, "Value"=→"C Int 2 6":dbl, "Python Object References Out"=w767:T5, "Session ID out"=w768:T4)  [unwired: 5 in]
                n213 = call-poly <vilib>:"Unpack.vi"("error in (no error)"=w766, "Python Object References In"=w767, "Session ID"=w768) -> ("error out"=w772:errorcluster, "Value"=→"t 1 6":dbl, "Python Object References Out"=w771:T5, "Session ID out"=w770:T4)  [unwired: 5 in]
                n214 = call-poly <vilib>:"Unpack.vi"("error in (no error)"=w772, "Python Object References In"=w771, "Session ID"=w770) -> ("error out"=w773:errorcluster, "Value"=→"t 2 6":dbl, "Python Object References Out"=w774:T5, "Session ID out"=w775:T4)  [unwired: 5 in]
                n215 = call-poly <vilib>:"Unpack.vi"("error in (no error)"=w773, "Python Object References In"=w774, "Session ID"=w775) -> ("error out"=w776:errorcluster, "Value"=→"t ref 6":dbl, "Session ID out"=w777:T4)  [unwired: 5 in, 1 out]
                n216 = call <vilib>:"Close Session.vi"("error in (no error)"=w776, "Session ID"=w777) -> ()  [unwired: 9 in, 1 out]
              }
              frame #2 {
                n217 = case shown="True" w814 {
                  tunnel: w818 -> [w822 w858]
                  tunnel: ["Temp 7" w843] -> w817
                  tunnel: ["Flow 7" w842] -> w816
                  tunnel: ["Conc 7" w841] -> w815
                  frame False {
                    n218 = call <vilib>:"New Session.vi"("Path to Python Module (.py File)"=path "C:/Users/User/Documents/LabVIEW Data/2015 Projects/Combined/WriteTFC.py") -> ("error out"=w831:errorcluster, "Session ID out"=w832:T4)  [unwired: 9 in]
                    n219 = call <vilib>:"Pack.vi"("Argument"=w822, "error in (no error)"=w831, "Session ID"=w832) -> ("error out"=w830:errorcluster, "Python Object References Out"=w826:T5, "Session ID out"=w833:T4)  [unwired: 6 in]
                    n220 = call <vilib>:"Pack.vi"("Argument"="Temp 7", "error in (no error)"=w830, "Python Object References In"=w826, "Session ID"=w833) -> ("error out"=w829:errorcluster, "Python Object References Out"=w825:T5, "Session ID out"=w823:T4)  [unwired: 5 in]
                    n221 = call <vilib>:"Pack.vi"("Argument"="Flow 7", "error in (no error)"=w829, "Python Object References In"=w825, "Session ID"=w823) -> ("error out"=w828:errorcluster, "Python Object References Out"=w824:T5, "Session ID out"=w837:T4)  [unwired: 5 in]
                    n222 = call <vilib>:"Pack.vi"("Argument"="Conc 7", "error in (no error)"=w828, "Python Object References In"=w824, "Session ID"=w837) -> ("error out"=w840:errorcluster, "Python Object References Out"=w839:T5, "Session ID out"=w838:T4)  [unwired: 5 in]
                    n223 = call <vilib>:"Call.vi"("Function or Method Name"="AppendResultFile", "error in (no error)"=w840, "Python Object References In"=w839, "Session ID"=w838) -> ("error out"=w827:errorcluster, "Session ID out"=w836:T4)  [unwired: 5 in, 1 out]
                    n224 = call <vilib>:"Close Session.vi"("error in (no error)"=w827, "Session ID"=w836) -> ()  [unwired: 9 in, 1 out]
                  }
                  frame True {
                    n225 = call <vilib>:"New Session.vi"("Path to Python Module (.py File)"=path "C:/Users/User/Documents/LabVIEW Data/2015 Projects/Combined/2parameter_MBDoE.py") -> ("error out"=w859:errorcluster, "Session ID out"=w860:T4)  [unwired: 9 in]
                    n226 = call <vilib>:"Pack.vi"("Argument"=w858, "error in (no error)"=w859, "Session ID"=w860) -> ("error out"=w856:errorcluster, "Python Object References Out"=w855:T5, "Session ID out"=w857:T4)  [unwired: 6 in]
                    n227 = call <vilib>:"Call.vi"("Function or Method Name"="onlineMBDoE", "error in (no error)"=w856, "Python Object References In"=w855, "Session ID"=w857) -> ("error out"=w850:errorcluster, "Python Object References Out"=w846:T5, "Session ID out"=w854:T4)  [unwired: 5 in]
                    n228 = call-poly <vilib>:"Unpack.vi"("error in (no error)"=w850, "Python Object References In"=w846, "Session ID"=w854) -> ("error out"=w849:errorcluster, "Value"=w843:dbl, "Python Object References Out"=w845:T5, "Session ID out"=w853:T4)  [unwired: 5 in]
                    n229 = call-poly <vilib>:"Unpack.vi"("error in (no error)"=w849, "Python Object References In"=w845, "Session ID"=w853) -> ("error out"=w848:errorcluster, "Value"=w842:dbl, "Python Object References Out"=w844:T5, "Session ID out"=w852:T4)  [unwired: 5 in]
                    n230 = call-poly <vilib>:"Unpack.vi"("error in (no error)"=w848, "Python Object References In"=w844, "Session ID"=w852) -> ("error out"=w847:errorcluster, "Value"=w841:dbl, "Session ID out"=w851:T4)  [unwired: 5 in, 1 out]
                    n231 = call <vilib>:"Close Session.vi"("error in (no error)"=w847, "Session ID"=w851) -> ()  [unwired: 9 in, 1 out]
                  }
                }
                "Temp 7" <- w817
                "Flow 7" <- w816
                "Conc 7" <- w815
              }
            }
            "Exp 7" <- TRUE
          }
          frame 9 {
            n232 = flat-sequence {
              tunnel: w870 -> [w878]
              tunnel: w865 -> [w871]
              tunnel: w865 -> [w917]
              tunnel: [w915] -> w864
              tunnel: w865 -> [w947]
              tunnel: [w946] -> w869
              tunnel: [w945] -> w868
              tunnel: [w944] -> w867
              tunnel: w866 -> [w943]
              frame #0 {
                # "make this include a write to record file step"
                n233 = call <vilib>:"New Session.vi"("Path to Python Module (.py File)"=path "C:/Users/User/Documents/LabVIEW Data/2015 Projects/Combined/HPLCandAppend.py") -> ("error out"=w889:errorcluster, "Session ID out"=w888:T4)  [unwired: 9 in]
                n234 = call <vilib>:"Pack.vi"("Argument"=w878, "error in (no error)"=w889, "Session ID"=w888) -> ("error out"=w875:errorcluster, "Python Object References Out"=w876:T5, "Session ID out"=w877:T4)  [unwired: 6 in]
                n235 = call <vilib>:"Pack.vi"("Argument"=w871, "error in (no error)"=w875, "Python Object References In"=w876, "Session ID"=w877) -> ("error out"=w874:errorcluster, "Python Object References Out"=w873:T5, "Session ID out"=w872:T4)  [unwired: 5 in]
                n236 = call <vilib>:"Call.vi"("Function or Method Name"="HPLC", "error in (no error)"=w874, "Python Object References In"=w873, "Session ID"=w872) -> ("error out"=w890:errorcluster, "Python Object References Out"=w881:T5, "Session ID out"=w882:T4)  [unwired: 5 in]
                n237 = call-poly <vilib>:"Unpack.vi"("error in (no error)"=w890, "Python Object References In"=w881, "Session ID"=w882) -> ("error out"=w891:errorcluster, "Value"=→"C BAcid 7":dbl, "Python Object References Out"=w886:T5, "Session ID out"=w885:T4)  [unwired: 5 in]
                n238 = call-poly <vilib>:"Unpack.vi"("error in (no error)"=w891, "Python Object References In"=w886, "Session ID"=w885) -> ("error out"=w892:errorcluster, "Value"=→"C EB 7":dbl, "Session ID out"=w887:T4)  [unwired: 5 in, 1 out]
                n239 = call <vilib>:"Close Session.vi"("error in (no error)"=w892, "Session ID"=w887) -> ()  [unwired: 9 in, 1 out]
              }
              frame #1 {
                # "make this include a write to record file step"
                n240 = call <vilib>:"New Session.vi"("Path to Python Module (.py File)"=path "C:/Users/User/Documents/LabVIEW Data/2015 Projects/Combined/2parameter_PE.py") -> ("error out"=w924:errorcluster, "Session ID out"=w921:T4)  [unwired: 9 in]
                n241 = call <vilib>:"Pack.vi"("Argument"=w917, "error in (no error)"=w924, "Session ID"=w921) -> ("error out"=w925:errorcluster, "Python Object References Out"=w923:T5, "Session ID out"=w922:T4)  [unwired: 6 in]
                n242 = call <vilib>:"Call.vi"("Function or Method Name"="onlinePE", "error in (no error)"=w925, "Python Object References In"=w923, "Session ID"=w922) -> ("error out"=w934:errorcluster, "Python Object References Out"=w930:T5, "Session ID out"=w926:T4)  [unwired: 5 in]
                n243 = call-poly <vilib>:"Unpack.vi"("error in (no error)"=w934, "Python Object References In"=w930, "Session ID"=w926) -> ("error out"=w935:errorcluster, "Value"=w915:dbl, "Python Object References Out"=w931:T5, "Session ID out"=w927:T4)  [unwired: 5 in]
                n244 = call-poly <vilib>:"Unpack.vi"("error in (no error)"=w935, "Python Object References In"=w931, "Session ID"=w927) -> ("error out"=w936:errorcluster, "Value"=→"Param 1 7":dbl, "Python Object References Out"=w932:T5, "Session ID out"=w928:T4)  [unwired: 5 in]
                n245 = call-poly <vilib>:"Unpack.vi"("error in (no error)"=w936, "Python Object References In"=w932, "Session ID"=w928) -> ("error out"=w937:errorcluster, "Value"=→"Param 2 7":dbl, "Python Object References Out"=w933:T5, "Session ID out"=w929:T4)  [unwired: 5 in]
                n246 = call-poly <vilib>:"Unpack.vi"("error in (no error)"=w937, "Python Object References In"=w933, "Session ID"=w929) -> ("error out"=w938:errorcluster, "Value"=→"Chi  7":dbl, "Python Object References Out"=w920:T5, "Session ID out"=w919:T4)  [unwired: 5 in]
                n247 = call-poly <vilib>:"Unpack.vi"("error in (no error)"=w938, "Python Object References In"=w920, "Session ID"=w919) -> ("error out"=w910:errorcluster, "Value"=→"Chi ref 7":dbl, "Python Object References Out"=w912:T5, "Session ID out"=w914:T4)  [unwired: 5 in]
                n248 = call-poly <vilib>:"Unpack.vi"("error in (no error)"=w910, "Python Object References In"=w912, "Session ID"=w914) -> ("error out"=w909:errorcluster, "Value"=→"C Int 1 7":dbl, "Python Object References Out"=w911:T5, "Session ID out"=w913:T4)  [unwired: 5 in]
                n249 = call-poly <vilib>:"Unpack.vi"("error in (no error)"=w909, "Python Object References In"=w911, "Session ID"=w913) -> ("error out"=w895:errorcluster, "Value"=→"C Int 2 7":dbl, "Python Object References Out"=w896:T5, "Session ID out"=w897:T4)  [unwired: 5 in]
                n250 = call-poly <vilib>:"Unpack.vi"("error in (no error)"=w895, "Python Object References In"=w896, "Session ID"=w897) -> ("error out"=w901:errorcluster, "Value"=→"t 1 7":dbl, "Python Object References Out"=w900:T5, "Session ID out"=w899:T4)  [unwired: 5 in]
                n251 = call-poly <vilib>:"Unpack.vi"("error in (no error)"=w901, "Python Object References In"=w900, "Session ID"=w899) -> ("error out"=w902:errorcluster, "Value"=→"t 2 7":dbl, "Python Object References Out"=w903:T5, "Session ID out"=w904:T4)  [unwired: 5 in]
                n252 = call-poly <vilib>:"Unpack.vi"("error in (no error)"=w902, "Python Object References In"=w903, "Session ID"=w904) -> ("error out"=w905:errorcluster, "Value"=→"t ref 7":dbl, "Session ID out"=w906:T4)  [unwired: 5 in, 1 out]
                n253 = call <vilib>:"Close Session.vi"("error in (no error)"=w905, "Session ID"=w906) -> ()  [unwired: 9 in, 1 out]
              }
              frame #2 {
                n254 = case shown="True" w943 {
                  tunnel: w947 -> [w951 w987]
                  tunnel: ["Temp 8" w972] -> w946
                  tunnel: ["Flow 8" w971] -> w945
                  tunnel: ["Conc 8" w970] -> w944
                  frame False {
                    n255 = call <vilib>:"New Session.vi"("Path to Python Module (.py File)"=path "C:/Users/User/Documents/LabVIEW Data/2015 Projects/Combined/WriteTFC.py") -> ("error out"=w960:errorcluster, "Session ID out"=w961:T4)  [unwired: 9 in]
                    n256 = call <vilib>:"Pack.vi"("Argument"=w951, "error in (no error)"=w960, "Session ID"=w961) -> ("error out"=w959:errorcluster, "Python Object References Out"=w955:T5, "Session ID out"=w962:T4)  [unwired: 6 in]
                    n257 = call <vilib>:"Pack.vi"("Argument"="Temp 8", "error in (no error)"=w959, "Python Object References In"=w955, "Session ID"=w962) -> ("error out"=w958:errorcluster, "Python Object References Out"=w954:T5, "Session ID out"=w952:T4)  [unwired: 5 in]
                    n258 = call <vilib>:"Pack.vi"("Argument"="Flow 8", "error in (no error)"=w958, "Python Object References In"=w954, "Session ID"=w952) -> ("error out"=w957:errorcluster, "Python Object References Out"=w953:T5, "Session ID out"=w966:T4)  [unwired: 5 in]
                    n259 = call <vilib>:"Pack.vi"("Argument"="Conc 8", "error in (no error)"=w957, "Python Object References In"=w953, "Session ID"=w966) -> ("error out"=w969:errorcluster, "Python Object References Out"=w968:T5, "Session ID out"=w967:T4)  [unwired: 5 in]
                    n260 = call <vilib>:"Call.vi"("Function or Method Name"="AppendResultFile", "error in (no error)"=w969, "Python Object References In"=w968, "Session ID"=w967) -> ("error out"=w956:errorcluster, "Session ID out"=w965:T4)  [unwired: 5 in, 1 out]
                    n261 = call <vilib>:"Close Session.vi"("error in (no error)"=w956, "Session ID"=w965) -> ()  [unwired: 9 in, 1 out]
                  }
                  frame True {
                    n262 = call <vilib>:"New Session.vi"("Path to Python Module (.py File)"=path "C:/Users/User/Documents/LabVIEW Data/2015 Projects/Combined/2parameter_MBDoE.py") -> ("error out"=w988:errorcluster, "Session ID out"=w989:T4)  [unwired: 9 in]
                    n263 = call <vilib>:"Pack.vi"("Argument"=w987, "error in (no error)"=w988, "Session ID"=w989) -> ("error out"=w985:errorcluster, "Python Object References Out"=w984:T5, "Session ID out"=w986:T4)  [unwired: 6 in]
                    n264 = call <vilib>:"Call.vi"("Function or Method Name"="onlineMBDoE", "error in (no error)"=w985, "Python Object References In"=w984, "Session ID"=w986) -> ("error out"=w979:errorcluster, "Python Object References Out"=w975:T5, "Session ID out"=w983:T4)  [unwired: 5 in]
                    n265 = call-poly <vilib>:"Unpack.vi"("error in (no error)"=w979, "Python Object References In"=w975, "Session ID"=w983) -> ("error out"=w978:errorcluster, "Value"=w972:dbl, "Python Object References Out"=w974:T5, "Session ID out"=w982:T4)  [unwired: 5 in]
                    n266 = call-poly <vilib>:"Unpack.vi"("error in (no error)"=w978, "Python Object References In"=w974, "Session ID"=w982) -> ("error out"=w977:errorcluster, "Value"=w971:dbl, "Python Object References Out"=w973:T5, "Session ID out"=w981:T4)  [unwired: 5 in]
                    n267 = call-poly <vilib>:"Unpack.vi"("error in (no error)"=w977, "Python Object References In"=w973, "Session ID"=w981) -> ("error out"=w976:errorcluster, "Value"=w970:dbl, "Session ID out"=w980:T4)  [unwired: 5 in, 1 out]
                    n268 = call <vilib>:"Close Session.vi"("error in (no error)"=w976, "Session ID"=w980) -> ()  [unwired: 9 in, 1 out]
                  }
                }
                "Temp 8" <- w946
                "Flow 8" <- w945
                "Conc 8" <- w944
              }
            }
            "Exp 8" <- TRUE
          }
          frame 10 {
            n269 = flat-sequence {
              tunnel: w998 -> [w1006]
              tunnel: w993 -> [w999]
              tunnel: w993 -> [w1045]
              tunnel: [w1043] -> w992
              tunnel: w993 -> [_]
              tunnel: w997 -> [_]
              frame #0 {
                # "make this include a write to record file step"
                n270 = call <vilib>:"New Session.vi"("Path to Python Module (.py File)"=path "C:/Users/User/Documents/LabVIEW Data/2015 Projects/Combined/HPLCandAppend.py") -> ("error out"=w1017:errorcluster, "Session ID out"=w1016:T4)  [unwired: 9 in]
                n271 = call <vilib>:"Pack.vi"("Argument"=w1006, "error in (no error)"=w1017, "Session ID"=w1016) -> ("error out"=w1005:errorcluster, "Python Object References Out"=w1004:T5, "Session ID out"=w1003:T4)  [unwired: 6 in]
                n272 = call <vilib>:"Pack.vi"("Argument"=w999, "error in (no error)"=w1005, "Python Object References In"=w1004, "Session ID"=w1003) -> ("error out"=w1000:errorcluster, "Python Object References Out"=w1001:T5, "Session ID out"=w1002:T4)  [unwired: 5 in]
                n273 = call <vilib>:"Call.vi"("Function or Method Name"="HPLC", "error in (no error)"=w1000, "Python Object References In"=w1001, "Session ID"=w1002) -> ("error out"=w1018:errorcluster, "Python Object References Out"=w1009:T5, "Session ID out"=w1010:T4)  [unwired: 5 in]
                n274 = call-poly <vilib>:"Unpack.vi"("error in (no error)"=w1018, "Python Object References In"=w1009, "Session ID"=w1010) -> ("error out"=w1019:errorcluster, "Value"=→"C BAcid 8":dbl, "Python Object References Out"=w1014:T5, "Session ID out"=w1013:T4)  [unwired: 5 in]
                n275 = call-poly <vilib>:"Unpack.vi"("error in (no error)"=w1019, "Python Object References In"=w1014, "Session ID"=w1013) -> ("error out"=w1020:errorcluster, "Value"=→"C EB 8":dbl, "Session ID out"=w1015:T4)  [unwired: 5 in, 1 out]
                n276 = call <vilib>:"Close Session.vi"("error in (no error)"=w1020, "Session ID"=w1015) -> ()  [unwired: 9 in, 1 out]
              }
              frame #1 {
                # "make this include a write to record file step"
                n277 = call <vilib>:"New Session.vi"("Path to Python Module (.py File)"=path "C:/Users/User/Documents/LabVIEW Data/2015 Projects/Combined/2parameter_PE.py") -> ("error out"=w1052:errorcluster, "Session ID out"=w1049:T4)  [unwired: 9 in]
                n278 = call <vilib>:"Pack.vi"("Argument"=w1045, "error in (no error)"=w1052, "Session ID"=w1049) -> ("error out"=w1053:errorcluster, "Python Object References Out"=w1051:T5, "Session ID out"=w1050:T4)  [unwired: 6 in]
                n279 = call <vilib>:"Call.vi"("Function or Method Name"="onlinePE", "error in (no error)"=w1053, "Python Object References In"=w1051, "Session ID"=w1050) -> ("error out"=w1062:errorcluster, "Python Object References Out"=w1058:T5, "Session ID out"=w1054:T4)  [unwired: 5 in]
                n280 = call-poly <vilib>:"Unpack.vi"("error in (no error)"=w1062, "Python Object References In"=w1058, "Session ID"=w1054) -> ("error out"=w1063:errorcluster, "Value"=w1043:dbl, "Python Object References Out"=w1059:T5, "Session ID out"=w1055:T4)  [unwired: 5 in]
                n281 = call-poly <vilib>:"Unpack.vi"("error in (no error)"=w1063, "Python Object References In"=w1059, "Session ID"=w1055) -> ("error out"=w1064:errorcluster, "Value"=→"Param 1 8":dbl, "Python Object References Out"=w1060:T5, "Session ID out"=w1056:T4)  [unwired: 5 in]
                n282 = call-poly <vilib>:"Unpack.vi"("error in (no error)"=w1064, "Python Object References In"=w1060, "Session ID"=w1056) -> ("error out"=w1065:errorcluster, "Value"=→"Param 2 8":dbl, "Python Object References Out"=w1061:T5, "Session ID out"=w1057:T4)  [unwired: 5 in]
                n283 = call-poly <vilib>:"Unpack.vi"("error in (no error)"=w1065, "Python Object References In"=w1061, "Session ID"=w1057) -> ("error out"=w1066:errorcluster, "Value"=→"Chi  8":dbl, "Python Object References Out"=w1048:T5, "Session ID out"=w1047:T4)  [unwired: 5 in]
                n284 = call-poly <vilib>:"Unpack.vi"("error in (no error)"=w1066, "Python Object References In"=w1048, "Session ID"=w1047) -> ("error out"=w1038:errorcluster, "Value"=→"Chi ref 8":dbl, "Python Object References Out"=w1040:T5, "Session ID out"=w1042:T4)  [unwired: 5 in]
                n285 = call-poly <vilib>:"Unpack.vi"("error in (no error)"=w1038, "Python Object References In"=w1040, "Session ID"=w1042) -> ("error out"=w1037:errorcluster, "Value"=→"C Int 1 8":dbl, "Python Object References Out"=w1039:T5, "Session ID out"=w1041:T4)  [unwired: 5 in]
                n286 = call-poly <vilib>:"Unpack.vi"("error in (no error)"=w1037, "Python Object References In"=w1039, "Session ID"=w1041) -> ("error out"=w1023:errorcluster, "Value"=→"C Int 2 8":dbl, "Python Object References Out"=w1024:T5, "Session ID out"=w1025:T4)  [unwired: 5 in]
                n287 = call-poly <vilib>:"Unpack.vi"("error in (no error)"=w1023, "Python Object References In"=w1024, "Session ID"=w1025) -> ("error out"=w1029:errorcluster, "Value"=→"t 1 8":dbl, "Python Object References Out"=w1028:T5, "Session ID out"=w1027:T4)  [unwired: 5 in]
                n288 = call-poly <vilib>:"Unpack.vi"("error in (no error)"=w1029, "Python Object References In"=w1028, "Session ID"=w1027) -> ("error out"=w1030:errorcluster, "Value"=→"t 2 8":dbl, "Python Object References Out"=w1031:T5, "Session ID out"=w1032:T4)  [unwired: 5 in]
                n289 = call-poly <vilib>:"Unpack.vi"("error in (no error)"=w1030, "Python Object References In"=w1031, "Session ID"=w1032) -> ("error out"=w1033:errorcluster, "Value"=→"t ref 8":dbl, "Session ID out"=w1034:T4)  [unwired: 5 in, 1 out]
                n290 = call <vilib>:"Close Session.vi"("error in (no error)"=w1033, "Session ID"=w1034) -> ()  [unwired: 9 in, 1 out]
              }
              frame #2 {
              }
            }
          }
        }
        "Number Read" <- w125
      }
      frame True {
        w1071 = 0
      }
    }
    n291 = timed-loop {
      tunnel: w121 -> [w1275]
      tunnel: w120 -> [w1274]
      tunnel: [w1223] -> w119
      tunnel: [w1222] -> w118
      timing: w117 -> [_]
      timing-out: [_] -> w116
      tunnel: w115 -> [w1209]
      tunnel: w114 -> [w1213]
      tunnel: w113 -> [w1212]
      tunnel: [w1208] -> w112
      tunnel: [w1207] -> w111
      tunnel: [w1187] -> w110
      tunnel: w101 -> [w1204]
      tunnel: w100 -> [w1203]
      tunnel: w99 -> [w1137]
      tunnel: w109 -> [w1192]
      tunnel: w108 -> [w1191]
      tunnel: w107 -> [w1190]
      tunnel: w106 -> [w1189]
      shift-right: [w1142] -> _
      shift-left: _ -> [w1181]
      tunnel: [w1184] -> w105
      tunnel: [w1183] -> w104
      tunnel: ["Stop everything"] -> w102
      tunnel: "Automated Experiments or Direct Control" -> [w1143]
      tunnel: w88 -> [w1132]
      tunnel: w87 -> [w1131]
      tunnel: [w1130] -> w86
      tunnel: [w1129] -> w85
      i -> [w1166]
      stop <- w1174 stop-if-true
      w1188 = 9.0 ("Safety Shut Down Pressure (barg)")
      w1205 = 180
      # "in case out of range changes conc to within possible range"
      # "1st 4 flowrates\n5,6 temperatures\n7 pressure (1)\n8 gas (1)"
      # "temperature or syringe or pressure"
      # "We are graphing in barg"
      # "temperature or syringe"
      # "Empty Syringe has level of 50"
      n292 = node-c288() -> ()  [unwired: 1 in, 1 out]
      n293 = call-poly <vilib>:"DAQmx Read.vi"("task/channels in"=w1132, "error in"=w1131) -> ("task out"=w1130:refnum<k21>, "data"=w1125:dbl, "error out"=w1129:errorcluster)  [unwired: 11 in]
      n294 = case shown="True" "Change New Set Points" {
        frame False {
        }
        frame True {
          w1655 = 20
          w1649 = ","
          n295 = Divide(x="Set Point 1", y=w1655) -> (x/y=w1632:dbl)
          n296 = Divide(x="Set Point 2", y=w1655) -> (x/y=w1634:dbl)
          n297 = Divide(x="Set Point 3", y=w1655) -> (x/y=w1636:dbl)
          n298 = Divide(x="Set Point 4", y=w1655) -> (x/y=w1638:dbl)
          n299 = Multiply(x=w1632, y=100) -> (x*y=w1644:dbl)
          n300 = Multiply(x=w1634, y=100) -> (x*y=w1645:dbl)
          n301 = Multiply(x=w1636, y=100) -> (x*y=w1646:dbl)
          n302 = Multiply(x=w1638, y=100) -> (x*y=w1647:dbl)
          n303 = Format Into String(w1645) -> (resulting string=w1652:string)  [unwired: 3 in, 1 out]
          n304 = Format Into String(w1644) -> (resulting string=w1651:string)  [unwired: 3 in, 1 out]
          n305 = Format Into String(w1646) -> (resulting string=w1653:string)  [unwired: 3 in, 1 out]
          n306 = Format Into String(w1647) -> (resulting string=w1654:string)  [unwired: 3 in, 1 out]
          n307 = Concatenate Strings("?BSI_SetFlowSetPoints ", w1651, w1649, w1652, w1649, w1653, w1649, w1654, w1649, "*,*,*,*,*,*,*,*,*,*,*,*,*,*,*,*,*,*,*,*,*,*,*,*,*,*") -> (w1631:string)
          n308 = stacked-sequence {
            seq-local: [w1656 _ _] -> [_ _ w1689]
            tunnel: w1631 -> [w1656 _ _]
            frame #0 {
              # "Write Text to Clipboard"
              n309 = String Length(string=w1656) -> (length=w1665:i32)
              n310 = Increment(x=w1665) -> (x+1=w1661:i32)
              n311 = dll-call lib="kernel32" fn="GlobalAlloc"("Flags"=i16 0 ("Format"), "Size"=w1661) -> (w1660:i32)  [unwired: 5 in, 2 out]
              n312 = dll-call lib="kernel32" fn="GlobalLock"("hGlobalMemory"=w1660) -> (w1663:i32)  [unwired: 4 in, 2 out]
              n313 = dll-call lib="kernel32" fn="lstrcpy"("Flags"=w1663, "String"=w1656) -> (w1662:i32)  [unwired: 5 in, 2 out]
              n314 = stacked-sequence {
                tunnel: w1662 -> [_]
                tunnel: w1660 -> [w1684]
                tunnel: [w1683] -> w1659
                frame #0 {
                  n315 = dll-call lib="kernel32" fn="LocalUnlock"("hGlobalMemory"=w1684) -> (w1683:i32)  [unwired: 4 in, 2 out]
                }
              }
              "Error Out 4" <- w1659
              n316 = case shown="0" w1659 {
                selector: w1659 -> [_ w1680]
                tunnel: w1660 -> [w1666 _]
                tunnel: [w1667 w1679] -> w1658
                frame 0 {
                  n317 = dll-call lib="user32" fn="OpenClipboard"("owner"=i16 0) -> (w1668:i32)  [unwired: 4 in, 2 out]
                  n318 = case shown="1, Default" w1668 {
                    selector: w1668 -> [w1672 _]
                    tunnel: [w1670 w1675] -> w1667
                    tunnel: w1666 -> [_ w1674]
                    frame 0 {
                      n319 = Equal To 0?(x=w1672) -> (x = 0?=w1673:bool)
                      n320 = Bundle(w1673, w1672, "source"="Error opening clipboard") -> (w1670:cluster{bool, i32, "source":string})  [unwired: 1 in]
                    }
                    frame 1, Default {
                      n321 = stacked-sequence {
                        tunnel: [_ _ _ cluster{bool, i32, "source":string} {FALSE, 0, "source"=""} ("Output Element")] -> w1675
                        tunnel: w1674 -> [_ w1676 _ _]
                        frame #0 {
                          n322 = dll-call lib="user32" fn="EmptyClipboard"() -> ()  [unwired: 4 in, 2 out]
                        }
                        frame #1 {
                          n323 = dll-call lib="user32" fn="SetClipboardData"("Format"=1, "Data"=w1676) -> ()  [unwired: 6 in, 2 out]
                        }
                        frame #2 {
                          n324 = dll-call lib="user32" fn="CloseClipboard"() -> ()  [unwired: 4 in, 2 out]
                        }
                        frame #3 {
                        }
                      }
                    }
                  }
                }
                frame 1, Default {
                  n325 = Not Equal To 0?(x=w1680) -> (x != 0?=w1681:bool)
                  n326 = Bundle(w1681, w1680, "source"="Error copying text to clipboard") -> (w1679:cluster{bool, i32, "source":string})  [unwired: 1 in]
                }
              }
              "Write error out 4" <- w1658
              n327 = local write "Write Set Point Status"("Running" ("Status")) -> ()
            }
            frame #1 {
              # "Wait 500 milliseconds"
              n328 = Wait (ms)(milliseconds to wait=u32 500) -> ()  [unwired: 1 out]
            }
            frame #2 {
              # "Read Text From Clipboard"
              n329 = dll-call lib="user32" fn="OpenClipboard"("owner"=i16 0) -> (w1691:i32)  [unwired: 4 in, 2 out]
              n330 = case shown="1, Default" w1691 {
                selector: w1691 -> [w1697 _]
                tunnel: ["" w1702] -> w1686
                tunnel: [w1695 cluster{bool, i32, "source":string} {FALSE, 0, "source"=""} ("Output Element")] -> w1690
                frame 0 {
                  n331 = Equal To 0?(x=w1697) -> (x = 0?=w1698:bool)
                  n332 = Bundle(w1698, w1697, "source"="No text in clipboard available!") -> (w1695:cluster{bool, i32, "source":string})  [unwired: 1 in]
                }
                frame 1, Default {
                  n333 = dll-call lib="user32" fn="GetClipboardData"("uFormat"=1 ("hGlobalMemory")) -> (w1703:i32)  [unwired: 4 in, 2 out]
                  n334 = dll-call lib="kernel32" fn="GlobalLock"("hGlobalMemory"=w1703) -> (w1702:string, "hGlobalMemory"=w1700:i32)  [unwired: 3 in, 2 out]
                  n335 = stacked-sequence {
                    tunnel: w1700 -> [w1705 _]
                    frame #0 {
                      n336 = dll-call lib="kernel32" fn="LocalUnlock"("hGlobalMemory"=w1705) -> ()  [unwired: 5 in, 2 out]
                    }
                    frame #1 {
                      n337 = dll-call lib="user32" fn="CloseClipboard"() -> ()  [unwired: 4 in, 2 out]
                    }
                  }
                }
              }
              "Text Read From Clipboard 4" <- w1686
              "Read error out 4" <- w1690
              n338 = Equal?(x=w1689, y=w1686) -> (x = y?=w1688:bool)
              n339 = case shown="True" w1688 {
                tunnel: ["Response OK" "Failed: No Response from Lab Interface"] -> w1687
                frame False {
                }
                frame True {
                }
              }
              "Write Set Point Status" <- w1687
            }
          }
        }
      }
      n340 = Multiply(x=5.1522, y=w1125) -> (x*y=w1128:dbl)
      n341 = Add(x=-2.6852, y=w1128) -> (x+y=w1124:dbl)
      "Liquid Inlet Pressure (bar g)" <- w1124
      n342 = Or(x="Read Set Points", y="Change New Set Points") -> (x .or. y?=w1179:bool)
      n343 = Or(x="Test Gas Communication", y=w1179) -> (x .or. y?=w1176:bool)
      n344 = case shown="True" "Test Gas Communication" {
        frame False {
        }
        frame True {
          w1580 = "?BSI_Test"  # ?BSI_Test
          n345 = stacked-sequence {
            seq-local: [w1581 _ _] -> [_ _ w1614]
            tunnel: w1580 -> [w1581 _ _]
            frame #0 {
              # "Write Text to Clipboard"
              n346 = String Length(string=w1581) -> (length=w1590:i32)
              n347 = Increment(x=w1590) -> (x+1=w1586:i32)
              n348 = dll-call lib="kernel32" fn="GlobalAlloc"("Flags"=i16 0 ("Format"), "Size"=w1586) -> (w1585:i32)  [unwired: 5 in, 2 out]
              n349 = dll-call lib="kernel32" fn="GlobalLock"("hGlobalMemory"=w1585) -> (w1588:i32)  [unwired: 4 in, 2 out]
              n350 = dll-call lib="kernel32" fn="lstrcpy"("Flags"=w1588, "String"=w1581) -> (w1587:i32)  [unwired: 5 in, 2 out]
              n351 = stacked-sequence {
                tunnel: w1587 -> [_]
                tunnel: w1585 -> [w1609]
                tunnel: [w1608] -> w1584
                frame #0 {
                  n352 = dll-call lib="kernel32" fn="LocalUnlock"("hGlobalMemory"=w1609) -> (w1608:i32)  [unwired: 4 in, 2 out]
                }
              }
              "Error Out" <- w1584
              n353 = case shown="1, Default" w1584 {
                selector: w1584 -> [_ w1605]
                tunnel: w1585 -> [w1591 _]
                tunnel: [w1592 w1604] -> w1583
                frame 0 {
                  n354 = dll-call lib="user32" fn="OpenClipboard"("owner"=i16 0) -> (w1593:i32)  [unwired: 4 in, 2 out]
                  n355 = case shown="0" w1593 {
                    selector: w1593 -> [w1597 _]
                    tunnel: [w1595 w1600] -> w1592
                    tunnel: w1591 -> [_ w1599]
                    frame 0 {
                      n356 = Equal To 0?(x=w1597) -> (x = 0?=w1598:bool)
                      n357 = Bundle(w1598, w1597, "source"="Error opening clipboard") -> (w1595:cluster{bool, i32, "source":string})  [unwired: 1 in]
                    }
                    frame 1, Default {
                      n358 = stacked-sequence {
                        tunnel: [_ _ _ cluster{bool, i32, "source":string} {FALSE, 0, "source"=""} ("Output Element")] -> w1600
                        tunnel: w1599 -> [_ w1601 _ _]
                        frame #0 {
                          n359 = dll-call lib="user32" fn="EmptyClipboard"() -> ()  [unwired: 4 in, 2 out]
                        }
                        frame #1 {
                          n360 = dll-call lib="user32" fn="SetClipboardData"("Format"=1, "Data"=w1601) -> ()  [unwired: 6 in, 2 out]
                        }
                        frame #2 {
                          n361 = dll-call lib="user32" fn="CloseClipboard"() -> ()  [unwired: 4 in, 2 out]
                        }
                        frame #3 {
                        }
                      }
                    }
                  }
                }
                frame 1, Default {
                  n362 = Not Equal To 0?(x=w1605) -> (x != 0?=w1606:bool)
                  n363 = Bundle(w1606, w1605, "source"="Error copying text to clipboard") -> (w1604:cluster{bool, i32, "source":string})  [unwired: 1 in]
                }
              }
              "Write error out" <- w1583
              n364 = local write "Test Status"("Running" ("Status")) -> ()
            }
            frame #1 {
              # "Wait 500 milliseconds"
              n365 = Wait (ms)(milliseconds to wait=u32 500) -> ()  [unwired: 1 out]
            }
            frame #2 {
              # "Read Text From Clipboard"
              n366 = dll-call lib="user32" fn="OpenClipboard"("owner"=i16 0) -> (w1616:i32)  [unwired: 4 in, 2 out]
              n367 = case shown="1, Default" w1616 {
                selector: w1616 -> [w1622 _]
                tunnel: ["" w1627] -> w1611
                tunnel: [w1620 cluster{bool, i32, "source":string} {FALSE, 0, "source"=""} ("Output Element")] -> w1615
                frame 0 {
                  n368 = Equal To 0?(x=w1622) -> (x = 0?=w1623:bool)
                  n369 = Bundle(w1623, w1622, "source"="No text in clipboard available!") -> (w1620:cluster{bool, i32, "source":string})  [unwired: 1 in]
                }
                frame 1, Default {
                  n370 = dll-call lib="user32" fn="GetClipboardData"("uFormat"=1 ("hGlobalMemory")) -> (w1628:i32)  [unwired: 4 in, 2 out]
                  n371 = dll-call lib="kernel32" fn="GlobalLock"("hGlobalMemory"=w1628) -> (w1627:string, "hGlobalMemory"=w1625:i32)  [unwired: 3 in, 2 out]
                  n372 = stacked-sequence {
                    tunnel: w1625 -> [w1630 _]
                    frame #0 {
                      n373 = dll-call lib="kernel32" fn="LocalUnlock"("hGlobalMemory"=w1630) -> ()  [unwired: 5 in, 2 out]
                    }
                    frame #1 {
                      n374 = dll-call lib="user32" fn="CloseClipboard"() -> ()  [unwired: 4 in, 2 out]
                    }
                  }
                }
              }
              "Text Read From Clipboard" <- w1611
              "Read error out" <- w1615
              n375 = Equal?(x=w1614, y=w1611) -> (x = y?=w1613:bool)
              n376 = case shown="True" w1613 {
                tunnel: ["Response OK" "Failed: No Response from Lab Interface"] -> w1612
                frame False {
                }
                frame True {
                }
              }
              "Test Status" <- w1612
            }
          }
        }
      }
      n377 = case shown="True" "Read Set Points" {
        frame False {
        }
        frame True {
          w1454 = "?BSI_ReadFlowSetPoints"  # ?BSI_ReadFlowSetPoints
          n378 = stacked-sequence {
            seq-local: [w1455 _ _] -> [_ _ w1488]
            tunnel: w1454 -> [w1455 _ _]
            frame #0 {
              # "Write Text to Clipboard"
              n379 = String Length(string=w1455) -> (length=w1464:i32)
              n380 = Increment(x=w1464) -> (x+1=w1460:i32)
              n381 = dll-call lib="kernel32" fn="GlobalAlloc"("Flags"=i16 0 ("Format"), "Size"=w1460) -> (w1459:i32)  [unwired: 5 in, 2 out]
              n382 = dll-call lib="kernel32" fn="GlobalLock"("hGlobalMemory"=w1459) -> (w1462:i32)  [unwired: 4 in, 2 out]
              n383 = dll-call lib="kernel32" fn="lstrcpy"("Flags"=w1462, "String"=w1455) -> (w1461:i32)  [unwired: 5 in, 2 out]
              n384 = stacked-sequence {
                tunnel: w1461 -> [_]
                tunnel: w1459 -> [w1483]
                tunnel: [w1482] -> w1458
                frame #0 {
                  n385 = dll-call lib="kernel32" fn="LocalUnlock"("hGlobalMemory"=w1483) -> (w1482:i32)  [unwired: 4 in, 2 out]
                }
              }
              "Error Out 3" <- w1458
              n386 = case shown="0" w1458 {
                selector: w1458 -> [_ w1479]
                tunnel: w1459 -> [w1465 _]
                tunnel: [w1466 w1478] -> w1457
                frame 0 {
                  n387 = dll-call lib="user32" fn="OpenClipboard"("owner"=i16 0) -> (w1467:i32)  [unwired: 4 in, 2 out]
                  n388 = case shown="1, Default" w1467 {
                    selector: w1467 -> [w1471 _]
                    tunnel: [w1469 w1474] -> w1466
                    tunnel: w1465 -> [_ w1473]
                    frame 0 {
                      n389 = Equal To 0?(x=w1471) -> (x = 0?=w1472:bool)
                      n390 = Bundle(w1472, w1471, "source"="Error opening clipboard") -> (w1469:cluster{bool, i32, "source":string})  [unwired: 1 in]
                    }
                    frame 1, Default {
                      n391 = stacked-sequence {
                        tunnel: [_ _ _ cluster{bool, i32, "source":string} {FALSE, 0, "source"=""} ("Output Element")] -> w1474
                        tunnel: w1473 -> [_ w1475 _ _]
                        frame #0 {
                          n392 = dll-call lib="user32" fn="EmptyClipboard"() -> ()  [unwired: 4 in, 2 out]
                        }
                        frame #1 {
                          n393 = dll-call lib="user32" fn="SetClipboardData"("Format"=1, "Data"=w1475) -> ()  [unwired: 6 in, 2 out]
                        }
                        frame #2 {
                          n394 = dll-call lib="user32" fn="CloseClipboard"() -> ()  [unwired: 4 in, 2 out]
                        }
                        frame #3 {
                        }
                      }
                    }
                  }
                }
                frame 1, Default {
                  n395 = Not Equal To 0?(x=w1479) -> (x != 0?=w1480:bool)
                  n396 = Bundle(w1480, w1479, "source"="Error copying text to clipboard") -> (w1478:cluster{bool, i32, "source":string})  [unwired: 1 in]
                }
              }
              "Write error out 3" <- w1457
              n397 = local write "Read Set Point Status"("Running" ("Status")) -> ()
            }
            frame #1 {
              # "Wait 500 milliseconds"
              n398 = Wait (ms)(milliseconds to wait=u32 500) -> ()  [unwired: 1 out]
            }
            frame #2 {
              # "Read Text From Clipboard"
              n399 = dll-call lib="user32" fn="OpenClipboard"("owner"=i16 0) -> (w1490:i32)  [unwired: 4 in, 2 out]
              n400 = case shown="1, Default" w1490 {
                selector: w1490 -> [w1496 _]
                tunnel: ["" w1501] -> w1485
                tunnel: [w1494 cluster{bool, i32, "source":string} {FALSE, 0, "source"=""} ("Output Element")] -> w1489
                frame 0 {
                  n401 = Equal To 0?(x=w1496) -> (x = 0?=w1497:bool)
                  n402 = Bundle(w1497, w1496, "source"="No text in clipboard available!") -> (w1494:cluster{bool, i32, "source":string})  [unwired: 1 in]
                }
                frame 1, Default {
                  n403 = dll-call lib="user32" fn="GetClipboardData"("uFormat"=1 ("hGlobalMemory")) -> (w1502:i32)  [unwired: 4 in, 2 out]
                  n404 = dll-call lib="kernel32" fn="GlobalLock"("hGlobalMemory"=w1502) -> (w1501:string, "hGlobalMemory"=w1499:i32)  [unwired: 3 in, 2 out]
                  n405 = stacked-sequence {
                    tunnel: w1499 -> [w1504 _]
                    frame #0 {
                      n406 = dll-call lib="kernel32" fn="LocalUnlock"("hGlobalMemory"=w1504) -> ()  [unwired: 5 in, 2 out]
                    }
                    frame #1 {
                      n407 = dll-call lib="user32" fn="CloseClipboard"() -> ()  [unwired: 4 in, 2 out]
                    }
                  }
                }
              }
              "Text Read From Clipboard 3" <- w1485
              "Read error out 3" <- w1489
              n408 = Equal?(x=w1488, y=w1485) -> (x = y?=w1487:bool)
              n409 = case shown="True" w1487 {
                tunnel: ["Response OK" "Failed: No Response from Lab Interface"] -> w1486
                frame False {
                }
                frame True {
                }
              }
              "Read Set Point Status" <- w1486
            }
          }
        }
      }
      n410 = for {
        N: 4 -> [_]
        tunnel: w1275 -> [w1804] mode=indexing
        tunnel: [w1802] -> w1269 mode=indexing
        tunnel: [w1799] -> w1264 mode=indexing
        tunnel: [w1798] -> w1263 mode=indexing
        tunnel: [w1797] -> w1262 mode=indexing
        tunnel: w1274 -> [w1796] mode=indexing
        i -> [w1803]
        n411 = call "NCS_GetFlowRateIs.vi"("error in (no error)"=w1796, "dosingunit"=w1803, "device handle in"=w1804) -> ("error out"=w1800:errorcluster, "flowrate is"=w1802:dbl, "device handle out"=w1801:u32)
        n412 = call "NCS_GetSyringeLevelIs.vi"("error in (no error)"=w1800, "dosingunit"=w1803, "device handle in"=w1801) -> ("error out"=w1797:errorcluster, "syringe level is"=w1799:dbl, "device handle out"=w1798:u32)
      }
      n413 = Index Array(array=w1264, index=0) -> (element=w1170:dbl)
      "Syringe Level 1" <- w1170
      n414 = Index Array(array=w1264, index=3) -> (element=w1167:dbl)
      "Syringe Level 4" <- w1167
      n415 = Index Array(array=w1264, index=1) -> (element=w1169:dbl)
      "Syringe Level 2" <- w1169
      n416 = Index Array(array=w1264, index=2) -> (element=w1168:dbl)
      "Syringe Level 3" <- w1168
      n417 = case shown="True" "Shut down in empty?\nLeft off, right on" {
        tunnel: [FALSE w1446] -> w1171
        tunnel: w1170 -> [_ w1445]
        tunnel: w1169 -> [_ w1444]
        tunnel: w1168 -> [_ w1443]
        tunnel: w1167 -> [_ w1442]
        frame False {
        }
        frame True {
          w1447 = 50
          n418 = Less Or Equal?(x=w1444, y=w1447) -> (x <= y?=w1453:bool)
          n419 = Less Or Equal?(x=w1445, y=w1447) -> (x <= y?=w1448:bool)
          n420 = Less Or Equal?(x=w1443, y=w1447) -> (x <= y?=w1451:bool)
          n421 = Less Or Equal?(x=w1442, y=w1447) -> (x <= y?=w1449:bool)
          n422 = Or(x=w1448, y=w1453) -> (x .or. y?=w1452:bool)
          n423 = Or(x=w1452, y=w1451) -> (x .or. y?=w1450:bool)
          n424 = Or(x=w1450, y=w1449) -> (x .or. y?=w1446:bool)
        }
      }
      n425 = Index Array(array=w1269, index=0) -> (element=w1154:dbl)
      "Flowrate 1 Low" <- w1154
      n426 = Index Array(array=w1269, index=3) -> (element=w1156:dbl)
      "Flowrate 4 Ethanol" <- w1156
      n427 = Index Array(array=w1269, index=1) -> (element=w1153:dbl)
      "Flowrate 2 High" <- w1153
      n428 = Index Array(array=w1269, index=2) -> (element=w1157:dbl)
      "Flowrate 3 Acid" <- w1157
      n429 = case shown="True" "Clear" {
        tunnel: w1181 -> [w1706 _]
        tunnel: [w1706 w1707] -> w1180
        frame False {
        }
        frame True {
          n430 = Initialize Array(0, 1) -> (w1707:i32[])
        }
      }
      n431 = call-poly <vilib>:"DAQmx Read.vi"("task/channels in"=w1192, "error in"=w1191) -> ("task out"=w1184:refnum<k21>, "data"=w1197:dbl[], "error out"=w1183:errorcluster)  [unwired: 11 in]
      n432 = Add(x=w1154, y=w1153) -> (x+y=w1159:dbl)
      n433 = Add(x=w1159, y=w1157) -> (x+y=w1158:dbl)
      n434 = Index Array(array=w1197, index=0) -> (element=w1195:dbl)
      n435 = Add(x=w1158, y=w1156) -> (x+y=w1155:dbl)
      "Total Flowrate (uL/min)" <- w1155
      n436 = Divide(x=w1154, y=w1155) -> (x/y=w1148:dbl)
      n437 = Multiply(x=w1195, y=w1190) -> (x*y=w1196:dbl)
      n438 = Multiply(x="Low Conc", y=w1148) -> (x*y=w1152:dbl)
      n439 = Add(x=w1196, y=w1189) -> (x+y=w1193:dbl)
      n440 = Divide(x=w1153, y=w1155) -> (x/y=w1149:dbl)
      n441 = Multiply(x="High Conc", y=0.9) -> (x*y=w1139:dbl)
      n442 = Multiply(x="Low Conc", y=0.9) -> (x*y=w1138:dbl)
      n443 = Multiply(x="High Conc", y=w1149) -> (x*y=w1151:dbl)
      n444 = Add(x=w1152, y=w1151) -> (x+y=→"Feed Concentration (M)":dbl)
      n445 = In Range and Coerce(upper limit=w1139, x=w1137, lower limit=w1138) -> (coerced(x)=w1134:dbl, In Range?=w1136:bool)
      n446 = case shown="True" w1136 {
        tunnel: [w1278 w1280] -> w1135
        tunnel: w1137 -> [_ w1280]
        tunnel: w1134 -> [w1278 _]
        tunnel: [TRUE FALSE] -> w1133
        frame False {
        }
        frame True {
        }
      }
      "Desired Conc Not Possible" <- w1133
      n447 = Multiply(x=w1193, y=0.0689476) -> (x*y=w1121:dbl)
      "Gas Back Pressure (barg)" <- w1121
      n448 = case shown="False" w1143 {
        tunnel: [w1776 w1777] -> w1260
        tunnel: w1203 -> [w1763 _]
        tunnel: w1135 -> [w1765 _]
        tunnel: "High Conc" -> [w1762 _]
        tunnel: "Low Conc" -> [w1761 _]
        frame False {
          w1760 = 0.1
          # "swapped it so syringe 2 is high and 1 is low"
          n449 = Subtract(x=w1762, y=w1761) -> (x-y=w1772:dbl)
          n450 = Subtract(x=1, y=w1760) -> (x-y=w1768:dbl)
          n451 = Divide(x=w1765, y=w1768) -> (x/y=w1774:dbl)
          n452 = Multiply(x=0, y=w1763) -> (x*y=w1758:dbl)
          n453 = Subtract(x=w1762, y=w1774) -> (x-y=w1771:dbl)
          n454 = Subtract(x=w1774, y=w1761) -> (x-y=w1773:dbl)
          n455 = Divide(x=w1773, y=w1772) -> (x/y=w1770:dbl)
          n456 = Divide(x=w1771, y=w1772) -> (x/y=w1769:dbl)
          n457 = Multiply(x=w1770, y=w1768) -> (x*y=w1767:dbl)
          n458 = Multiply(x=w1769, y=w1768) -> (x*y=w1766:dbl)
          n459 = Multiply(x=w1763, y=w1766) -> (x*y=w1756:dbl)
          n460 = Multiply(x=w1763, y=w1767) -> (x*y=w1757:dbl)
          n461 = Multiply(x=w1763, y=w1760) -> (x*y=w1759:dbl)
          n462 = Build Array(w1756, w1757, w1759, w1758) -> (w1776:dbl[])
          "Volumetric Fraction Acid" <- w1760
        }
        frame True {
          n463 = Build Array("Set Flowrate 1", "Set Flowrate 2", "Set Flowrate 3", "Set Flowrate 4") -> (w1777:dbl[])
        }
      }
      n464 = Build Array (concatenate)(w1180, w1121) -> (w1142:dbl[])
      "Calculated Pressure" <- w1142
      n465 = Greater Or Equal?(x=w1121, y=w1188) -> (x >= y?=w1185:bool)
      n466 = case shown="True" w1143 {
        tunnel: [w1711 FALSE] -> w1146
        tunnel: w1166 -> [w1710 _]
        frame False {
          # "changes set points for each new exp"
          n467 = Equal?(x=w1710, y=0) -> (x = y?=w1711:bool)
        }
        frame True {
          # "at end of each exp"
          # "doesnt automatically change set point"
        }
      }
      n468 = Or(x=w1146, y="Update Temperature Set Point") -> (x .or. y?=w1215:bool)
      n469 = case shown="True" w1215 {
        tunnel: w1213 -> [w1715 w1723]
        tunnel: w1212 -> [w1714 w1722]
        tunnel: [w1715 w1721] -> w1211
        tunnel: [w1714 w1720] -> w1210
        tunnel: w1209 -> [_ w1719]
        tunnel: w1143 -> [_ w1717]
        tunnel: w1204 -> [_ w1716]
        frame False {
        }
        frame True {
          n470 = case shown="True" w1717 {
            tunnel: [w1724 "Set Point (oC)"] -> w1718
            tunnel: w1716 -> [w1724 _]
            frame False {
            }
            frame True {
            }
          }
          n471 = call "CN7500_Write Set Point Value.vi"("Target Set Point Value"=w1718, "error in (no error)"=w1722, "Controller Number"=w1719, "VISA In"=w1723) -> ("error out"=w1720:errorcluster, "VISA Out"=w1721:refnum<visa-resource-name>)  [unwired: 6 in]
        }
      }
      n472 = Or(x="Generate Flow", y=w1146) -> (x .or. y?=w1147:bool)
      n473 = case shown="True" w1147 {
        tunnel: w1263 -> [w1783 w1788]
        tunnel: w1262 -> [w1782 w1787]
        tunnel: [w1782 w1786] -> w1161
        tunnel: [w1783 w1785] -> w1160
        tunnel: w1260 -> [_ w1784]
        frame False {
        }
        frame True {
          n474 = for {
            N: 4 -> [_]
            tunnel: w1788 -> [w1795] mode=indexing
            tunnel: w1787 -> [w1794] mode=indexing
            tunnel: [w1793] -> w1786 mode=indexing
            tunnel: [w1792] -> w1785 mode=indexing
            tunnel: w1784 -> [w1790] mode=indexing
            i -> [w1791]
            n475 = call "NCS_GenerateFlow.vi"("error in (no error)"=w1794, "flowrate"=w1790, "dosingunit"=w1791, "device handle in"=w1795) -> ("error out"=w1793:errorcluster, "device handle out"=w1792:u32)
          }
        }
      }
      n476 = call "CN7500_Read Process Value.vi"("error in (no error)"=w1210, "Controller Number"=w1209, "VISA In"=w1211) -> ("error out"=w1208:errorcluster, "Set Point Value"=w1199:dbl, "Process Value"=w1200:dbl, "VISA Out"=w1207:refnum<visa-resource-name>)  [unwired: 5 in]
      "Temp Set Point (oC)" <- w1199
      "Actual Temp (oC)" <- w1200
      n477 = Merge Signals(w1200, w1199) -> (→"Temperature":dynamicdata)
      n478 = Greater Or Equal?(x=w1200, y=w1205) -> (x >= y?=w1202:bool)
      n479 = Index Array(array=w1161, index=0) -> (element=w1250:errorcluster)
      n480 = Index Array(array=w1160, index=0) -> (element=w1251:u32)
      n481 = Index Array(array=w1161, index=3) -> (element=w1240:errorcluster)
      n482 = Index Array(array=w1161, index=2) -> (element=w1242:errorcluster)
      n483 = Index Array(array=w1161, index=1) -> (element=w1244:errorcluster)
      n484 = Index Array(array=w1160, index=3) -> (element=w1241:u32)
      n485 = Index Array(array=w1160, index=2) -> (element=w1243:u32)
      n486 = Index Array(array=w1160, index=1) -> (element=w1245:u32)
      n487 = case shown="False" "Stop Dose 2" {
        tunnel: w1245 -> [w1743 w1748]
        tunnel: w1244 -> [w1742 w1747]
        tunnel: [w1743 w1746] -> w1237
        tunnel: [w1742 w1745] -> w1236
        frame False {
        }
        frame True {
          n488 = call "NCS_Stop.vi"("error in (no error)"=w1747, "dosingunit"=1, "device handle in"=w1748) -> ("error out"=w1745:errorcluster, "device handle out"=w1746:u32)
        }
      }
      n489 = case shown="False" "Stop Dose 1" {
        tunnel: w1251 -> [w1750 w1755]
        tunnel: w1250 -> [w1749 w1754]
        tunnel: [w1750 w1753] -> w1239
        tunnel: [w1749 w1752] -> w1238
        frame False {
        }
        frame True {
          n490 = call "NCS_Stop.vi"("error in (no error)"=w1754, "dosingunit"=0, "device handle in"=w1755) -> ("error out"=w1752:errorcluster, "device handle out"=w1753:u32)
        }
      }
      n491 = case shown="False" "Stop Dose 3" {
        tunnel: w1243 -> [w1736 w1741]
        tunnel: w1242 -> [w1735 w1740]
        tunnel: [w1736 w1739] -> w1235
        tunnel: [w1735 w1738] -> w1234
        frame False {
        }
        frame True {
          n492 = call "NCS_Stop.vi"("error in (no error)"=w1740, "dosingunit"=2, "device handle in"=w1741) -> ("error out"=w1738:errorcluster, "device handle out"=w1739:u32)
        }
      }
      n493 = case shown="False" "Stop Dose 4" {
        tunnel: w1241 -> [w1729 w1734]
        tunnel: w1240 -> [w1728 w1733]
        tunnel: [w1729 w1732] -> w1233
        tunnel: [w1728 w1731] -> w1232
        frame False {
        }
        frame True {
          n494 = call "NCS_Stop.vi"("error in (no error)"=w1733, "dosingunit"=3, "device handle in"=w1734) -> ("error out"=w1731:errorcluster, "device handle out"=w1732:u32)
        }
      }
      n495 = case shown="False" "Safety or Emergency Syringe Control" {
        tunnel: w1239 -> [w1288 w1329]
        tunnel: w1238 -> [w1284 w1328]
        tunnel: w1237 -> [w1287 w1327]
        tunnel: w1236 -> [w1283 w1326]
        tunnel: w1235 -> [w1286 w1325]
        tunnel: w1234 -> [w1282 w1324]
        tunnel: w1233 -> [w1285 w1323]
        tunnel: w1232 -> [w1281 w1322]
        tunnel: [w1288 w1299] -> w1231
        tunnel: [w1287 w1298] -> w1230
        tunnel: [w1286 w1297] -> w1229
        tunnel: [w1285 w1296] -> w1228
        tunnel: [w1283 w1295] -> w1227
        tunnel: [w1282 w1294] -> w1226
        tunnel: [w1281 w1293] -> w1225
        tunnel: [w1284 w1289] -> w1224
        frame False {
        }
        frame True {
          n496 = case shown="False" "Calibrate 2" {
            tunnel: w1327 -> [w1428 w1433]
            tunnel: w1326 -> [w1427 w1432]
            tunnel: [w1428 w1431] -> w1316
            tunnel: [w1427 w1430] -> w1315
            frame False {
            }
            frame True {
              n497 = call "NCS_Calibrate.vi"("error in (no error)"=w1432, "dosingunit"=1, "device handle in"=w1433) -> ("error out"=w1430:errorcluster, "device handle out"=w1431:u32)
            }
          }
          n498 = case shown="False" "Calibrate 3" {
            tunnel: w1325 -> [w1421 w1426]
            tunnel: w1324 -> [w1420 w1425]
            tunnel: [w1421 w1424] -> w1314
            tunnel: [w1420 w1423] -> w1313
            frame False {
            }
            frame True {
              n499 = call "NCS_Calibrate.vi"("error in (no error)"=w1425, "dosingunit"=2, "device handle in"=w1426) -> ("error out"=w1423:errorcluster, "device handle out"=w1424:u32)
            }
          }
          n500 = case shown="False" "Calibrate 1" {
            tunnel: w1329 -> [w1435 w1440]
            tunnel: w1328 -> [w1434 w1439]
            tunnel: [w1435 w1438] -> w1318
            tunnel: [w1434 w1437] -> w1317
            frame False {
            }
            frame True {
              n501 = call "NCS_Calibrate.vi"("error in (no error)"=w1439, "dosingunit"=0, "device handle in"=w1440) -> ("error out"=w1437:errorcluster, "device handle out"=w1438:u32)
            }
          }
          n502 = case shown="False" "Calibrate 4" {
            tunnel: w1323 -> [w1414 w1419]
            tunnel: w1322 -> [w1413 w1418]
            tunnel: [w1414 w1417] -> w1312
            tunnel: [w1413 w1416] -> w1311
            frame False {
            }
            frame True {
              n503 = call "NCS_Calibrate.vi"("error in (no error)"=w1418, "dosingunit"=3, "device handle in"=w1419) -> ("error out"=w1416:errorcluster, "device handle out"=w1417:u32)
            }
          }
          n504 = case shown="False" "Empty 2" {
            tunnel: w1316 -> [w1394 w1398]
            tunnel: w1315 -> [w1393 w1396]
            tunnel: [w1394 w1397] -> w1302
            tunnel: [w1393 w1395] -> w1303
            frame False {
            }
            frame True {
              w1400 = 1
              n505 = call "NCS_GetFlowRateMax.vi"("error in (no error)"=w1396, "dosingunit"=w1400, "device handle in"=w1398) -> ("error out"=w1401:errorcluster, "flow rate max"=w1399:dbl, "device handle out"=w1402:u32)
              n506 = call "NCS_EmptySyrige.vi"("error in (no error)"=w1401, "flowrate"=w1399, "dosingunit"=w1400, "device handle in"=w1402) -> ("error out"=w1395:errorcluster, "device handle out"=w1397:u32)
            }
          }
          n507 = case shown="False" "Empty 1" {
            tunnel: w1318 -> [w1404 w1412]
            tunnel: w1317 -> [w1403 w1409]
            tunnel: [w1404 w1410] -> w1300
            tunnel: [w1403 w1407] -> w1301
            frame False {
            }
            frame True {
              w1406 = 0
              n508 = call "NCS_GetFlowRateMax.vi"("error in (no error)"=w1409, "dosingunit"=w1406, "device handle in"=w1412) -> ("error out"=w1408:errorcluster, "flow rate max"=w1405:dbl, "device handle out"=w1411:u32)
              n509 = call "NCS_EmptySyrige.vi"("error in (no error)"=w1408, "flowrate"=w1405, "dosingunit"=w1406, "device handle in"=w1411) -> ("error out"=w1407:errorcluster, "device handle out"=w1410:u32)
            }
          }
          n510 = case shown="False" "Empty 3" {
            tunnel: w1314 -> [w1384 w1385]
            tunnel: w1313 -> [w1383 w1386]
            tunnel: [w1384 w1387] -> w1304
            tunnel: [w1383 w1388] -> w1305
            frame False {
            }
            frame True {
              w1390 = 2
              n511 = call "NCS_GetFlowRateMax.vi"("error in (no error)"=w1386, "dosingunit"=w1390, "device handle in"=w1385) -> ("error out"=w1391:errorcluster, "flow rate max"=w1389:dbl, "device handle out"=w1392:u32)
              n512 = call "NCS_EmptySyrige.vi"("error in (no error)"=w1391, "flowrate"=w1389, "dosingunit"=w1390, "device handle in"=w1392) -> ("error out"=w1388:errorcluster, "device handle out"=w1387:u32)
            }
          }
          n513 = case shown="False" "Empty 4" {
            tunnel: w1312 -> [w1374 w1375]
            tunnel: w1311 -> [w1373 w1376]
            tunnel: [w1374 w1378] -> w1306
            tunnel: [w1373 w1377] -> w1307
            frame False {
            }
            frame True {
              w1380 = 3
              n514 = call "NCS_GetFlowRateMax.vi"("error in (no error)"=w1376, "dosingunit"=w1380, "device handle in"=w1375) -> ("error out"=w1381:errorcluster, "flow rate max"=w1379:dbl, "device handle out"=w1382:u32)
              n515 = call "NCS_EmptySyrige.vi"("error in (no error)"=w1381, "flowrate"=w1379, "dosingunit"=w1380, "device handle in"=w1382) -> ("error out"=w1377:errorcluster, "device handle out"=w1378:u32)
            }
          }
          n516 = case shown="False" "Refill 2" {
            tunnel: w1302 -> [w1354 w1358]
            tunnel: w1303 -> [w1353 w1356]
            tunnel: [w1354 w1357] -> w1298
            tunnel: [w1353 w1355] -> w1295
            frame False {
            }
            frame True {
              w1360 = 1
              n517 = call "NCS_GetFlowRateMax.vi"("error in (no error)"=w1356, "dosingunit"=w1360, "device handle in"=w1358) -> ("error out"=w1361:errorcluster, "flow rate max"=w1359:dbl, "device handle out"=w1362:u32)
              n518 = call "NCS_RefillSyrige.vi"("error in (no error)"=w1361, "flowrate"=w1359, "dosingunit"=w1360, "device handle in"=w1362) -> ("error out"=w1355:errorcluster, "device handle out"=w1357:u32)
            }
          }
          n519 = case shown="False" "Refill 1" {
            tunnel: w1300 -> [w1364 w1372]
            tunnel: w1301 -> [w1363 w1369]
            tunnel: [w1364 w1370] -> w1299
            tunnel: [w1363 w1367] -> w1289
            frame False {
            }
            frame True {
              w1366 = 0
              n520 = call "NCS_GetFlowRateMax.vi"("error in (no error)"=w1369, "dosingunit"=w1366, "device handle in"=w1372) -> ("error out"=w1368:errorcluster, "flow rate max"=w1365:dbl, "device handle out"=w1371:u32)
              n521 = call "NCS_RefillSyrige.vi"("error in (no error)"=w1368, "flowrate"=w1365, "dosingunit"=w1366, "device handle in"=w1371) -> ("error out"=w1367:errorcluster, "device handle out"=w1370:u32)
            }
          }
          n522 = case shown="False" "Refill 3" {
            tunnel: w1304 -> [w1344 w1345]
            tunnel: w1305 -> [w1343 w1346]
            tunnel: [w1344 w1347] -> w1297
            tunnel: [w1343 w1348] -> w1294
            frame False {
            }
            frame True {
              w1350 = 2
              n523 = call "NCS_GetFlowRateMax.vi"("error in (no error)"=w1346, "dosingunit"=w1350, "device handle in"=w1345) -> ("error out"=w1351:errorcluster, "flow rate max"=w1349:dbl, "device handle out"=w1352:u32)
              n524 = call "NCS_RefillSyrige.vi"("error in (no error)"=w1351, "flowrate"=w1349, "dosingunit"=w1350, "device handle in"=w1352) -> ("error out"=w1348:errorcluster, "device handle out"=w1347:u32)
            }
          }
          n525 = case shown="False" "Refill 4" {
            tunnel: w1306 -> [w1334 w1335]
            tunnel: w1307 -> [w1333 w1336]
            tunnel: [w1334 w1338] -> w1296
            tunnel: [w1333 w1337] -> w1293
            frame False {
            }
            frame True {
              w1340 = 3
              n526 = call "NCS_GetFlowRateMax.vi"("error in (no error)"=w1336, "dosingunit"=w1340, "device handle in"=w1335) -> ("error out"=w1341:errorcluster, "flow rate max"=w1339:dbl, "device handle out"=w1342:u32)
              n527 = call "NCS_RefillSyrige.vi"("error in (no error)"=w1341, "flowrate"=w1339, "dosingunit"=w1340, "device handle in"=w1342) -> ("error out"=w1337:errorcluster, "device handle out"=w1338:u32)
            }
          }
        }
      }
      n528 = Or(x=w1202, y=w1171) -> (x .or. y?=w1186:bool)
      n529 = Or(x=w1186, y=w1185) -> (x .or. y?=w1187:bool)
      n530 = Multiply(x="Minutes between Exp", y=60) -> (x*y=w1163:dbl)
      n531 = Divide(x=w1163, y=5) -> (x/y=w1164:dbl)
      n532 = Greater Or Equal?(x=w1166, y=w1164) -> (x >= y?=w1217:bool)
      n533 = Or(x=w1217, y=w1187) -> (x .or. y?=w1201:bool)
      n534 = Or(x="Skip Exp", y=w1201) -> (x .or. y?=w1218:bool)
      n535 = Or(x="Stop everything", y=w1218) -> (x .or. y?=w1174:bool)
      n536 = Or(x=w1174, y=w1176) -> (x .or. y?=w1175:bool)
      n537 = case shown="False" w1175 {
        tunnel: [w1505 0] -> w1144
        frame False {
          w1506 = "?BSI_ReadData"  # ?BSI_ReadData
          n538 = stacked-sequence {
            seq-local: [w1507 _ _] -> [_ _ w1562]
            tunnel: w1506 -> [w1507 _ _]
            tunnel: [_ _ w1540] -> w1505
            frame #0 {
              # "Write Text to Clipboard"
              n539 = String Length(string=w1507) -> (length=w1516:i32)
              n540 = Increment(x=w1516) -> (x+1=w1512:i32)
              n541 = dll-call lib="kernel32" fn="GlobalAlloc"("Flags"=i16 0 ("Format"), "Size"=w1512) -> (w1511:i32)  [unwired: 5 in, 2 out]
              n542 = dll-call lib="kernel32" fn="GlobalLock"("hGlobalMemory"=w1511) -> (w1514:i32)  [unwired: 4 in, 2 out]
              n543 = dll-call lib="kernel32" fn="lstrcpy"("Flags"=w1514, "String"=w1507) -> (w1513:i32)  [unwired: 5 in, 2 out]
              n544 = stacked-sequence {
                tunnel: w1513 -> [_]
                tunnel: w1511 -> [w1535]
                tunnel: [w1534] -> w1510
                frame #0 {
                  n545 = dll-call lib="kernel32" fn="LocalUnlock"("hGlobalMemory"=w1535) -> (w1534:i32)  [unwired: 4 in, 2 out]
                }
              }
              "Error Out 2" <- w1510
              n546 = case shown="0" w1510 {
                selector: w1510 -> [_ w1531]
                tunnel: w1511 -> [w1517 _]
                tunnel: [w1518 w1530] -> w1509
                frame 0 {
                  n547 = dll-call lib="user32" fn="OpenClipboard"("owner"=i16 0) -> (w1519:i32)  [unwired: 4 in, 2 out]
                  n548 = case shown="1, Default" w1519 {
                    selector: w1519 -> [w1523 _]
                    tunnel: [w1521 w1526] -> w1518
                    tunnel: w1517 -> [_ w1525]
                    frame 0 {
                      n549 = Equal To 0?(x=w1523) -> (x = 0?=w1524:bool)
                      n550 = Bundle(w1524, w1523, "source"="Error opening clipboard") -> (w1521:cluster{bool, i32, "source":string})  [unwired: 1 in]
                    }
                    frame 1, Default {
                      n551 = stacked-sequence {
                        tunnel: [_ _ _ cluster{bool, i32, "source":string} {FALSE, 0, "source"=""} ("Output Element")] -> w1526
                        tunnel: w1525 -> [_ w1527 _ _]
                        frame #0 {
                          n552 = dll-call lib="user32" fn="EmptyClipboard"() -> ()  [unwired: 4 in, 2 out]
                        }
                        frame #1 {
                          n553 = dll-call lib="user32" fn="SetClipboardData"("Format"=1, "Data"=w1527) -> ()  [unwired: 6 in, 2 out]
                        }
                        frame #2 {
                          n554 = dll-call lib="user32" fn="CloseClipboard"() -> ()  [unwired: 4 in, 2 out]
                        }
                        frame #3 {
                        }
                      }
                    }
                  }
                }
                frame 1, Default {
                  n555 = Not Equal To 0?(x=w1531) -> (x != 0?=w1532:bool)
                  n556 = Bundle(w1532, w1531, "source"="Error copying text to clipboard") -> (w1530:cluster{bool, i32, "source":string})  [unwired: 1 in]
                }
              }
              "Write error out 2" <- w1509
              n557 = local write "Read Flow Status"("Running" ("Status")) -> ()
            }
            frame #1 {
              # "Wait 500 milliseconds"
              n558 = Wait (ms)(milliseconds to wait=u32 500) -> ()  [unwired: 1 out]
            }
            frame #2 {
              # "Read Text From Clipboard"
              n559 = dll-call lib="user32" fn="OpenClipboard"("owner"=i16 0) -> (w1564:i32)  [unwired: 4 in, 2 out]
              n560 = case shown="1, Default" w1564 {
                selector: w1564 -> [w1570 _]
                tunnel: ["" w1575] -> w1555
                tunnel: [w1568 cluster{bool, i32, "source":string} {FALSE, 0, "source"=""} ("Output Element")] -> w1563
                frame 0 {
                  n561 = Equal To 0?(x=w1570) -> (x = 0?=w1571:bool)
                  n562 = Bundle(w1571, w1570, "source"="No text in clipboard available!") -> (w1568:cluster{bool, i32, "source":string})  [unwired: 1 in]
                }
                frame 1, Default {
                  n563 = dll-call lib="user32" fn="GetClipboardData"("uFormat"=1 ("hGlobalMemory")) -> (w1576:i32)  [unwired: 4 in, 2 out]
                  n564 = dll-call lib="kernel32" fn="GlobalLock"("hGlobalMemory"=w1576) -> (w1575:string, "hGlobalMemory"=w1573:i32)  [unwired: 3 in, 2 out]
                  n565 = stacked-sequence {
                    tunnel: w1573 -> [w1578 _]
                    frame #0 {
                      n566 = dll-call lib="kernel32" fn="LocalUnlock"("hGlobalMemory"=w1578) -> ()  [unwired: 5 in, 2 out]
                    }
                    frame #1 {
                      n567 = dll-call lib="user32" fn="CloseClipboard"() -> ()  [unwired: 4 in, 2 out]
                    }
                  }
                }
              }
              "Text Read From Clipboard 2" <- w1555
              "Read error out 2" <- w1563
              n568 = Search/Split String(string=w1555, search string/char (-)=" ") -> (substring before match=→"First waste string":string, match + rest of string=w1557:string)  [unwired: 1 in, 1 out]
              "Rest of string 1" <- w1557
              n569 = Search/Split String(string=w1557, search string/char (-)=",") -> (substring before match=w1552:string, match + rest of string=w1553:string)  [unwired: 1 in, 1 out]
              n570 = Search/Split String(string=w1553, search string/char (-)="n") -> (substring before match=w1550:string, match + rest of string=w1543:string)  [unwired: 1 in, 1 out]
              "Second Number 2" <- w1550
              "Rest of string 3" <- w1543
              n571 = Equal?(x=w1562, y=w1555) -> (x = y?=w1561:bool)
              n572 = Search/Split String(string=w1543, search string/char (-)="i") -> (substring before match=w1541:string, match + rest of string=w1546:string)  [unwired: 1 in, 1 out]
              "Third Number 3" <- w1541
              "Rest of string 4" <- w1546
              n573 = case shown="True" w1561 {
                tunnel: ["Response OK" "Failed: No Response from Lab Interface"] -> w1560
                frame False {
                }
                frame True {
                }
              }
              "Read Flow Status" <- w1560
              n574 = Search/Split String(string=w1546, search string/char (-)="l") -> (substring before match=w1544:string, match + rest of string=→"Rest of string 5":string)  [unwired: 1 in, 1 out]
              "Fourth Number 3" <- w1544
              n575 = Scan From String(input string=w1552) -> (output 1=w1540:dbl)  [unwired: 4 in, 3 out]
              "Gas Flow 1" <- w1540
              n576 = Scan From String(input string=w1550, initial scan location=1) -> (output 1=→"Gas Flow 2":dbl)  [unwired: 3 in, 3 out]
              n577 = Scan From String(input string=w1541, initial scan location=2) -> (output 1=→"Gas Flow 3":dbl)  [unwired: 3 in, 3 out]
              n578 = Scan From String(input string=w1544, initial scan location=3) -> (output 1=→"Gas Flow 4":dbl)  [unwired: 3 in, 3 out]
            }
          }
        }
        frame True {
        }
      }
      n579 = Merge Signals(w1154, w1153, w1157, w1156, w1200, w1199, w1121, w1144, w1124) -> (w1221:dynamicdata)
      n580 = call "Write To Measurement File"("Signals"=w1221) -> ()  [unwired: 16 in, 3 out]
      n581 = node-c288() -> ()  [unwired: 1 in, 1 out]
      n582 = Build Array(w1231, w1230, w1229, w1228) -> (w1223:u32[])
      n583 = Build Array(w1224, w1227, w1226, w1225) -> (w1222:errorcluster[])
      "loop ind" <- w1166
      "Safety Shut Down Temp" <- w1205
      "Safety Shut Down Pressure (barg)" <- w1188
    }
    n584 = Or(x=w102, y=w110) -> (x .or. y?=w103:bool)
    n585 = case shown="True" w103 {
      frame False {
      }
      frame True {
        w1072 = "?BSI_SetFlowSetPoints 0,0,0,0,*,*,*,*,*,*,*,*,*,*,*,*,*,*,*,*,*,*,*,*,*,*,*,*,*,*"  # ?BSI_SetFlowSetPoints 0,0,0,0,*,*,*,*,*,*,*,*,*,*,*,*,*,*,*,*,*,*,*,*,*,*,*,*,*,*
        n586 = stacked-sequence {
          seq-local: [w1073 _ _] -> [_ _ w1105]
          tunnel: w1072 -> [w1073 _ _]
          frame #0 {
            # "Write Text to Clipboard"
            n587 = String Length(string=w1073) -> (length=w1081:i32)
            n588 = Increment(x=w1081) -> (x+1=w1077:i32)
            n589 = dll-call lib="kernel32" fn="GlobalAlloc"("Flags"=i16 0 ("Format"), "Size"=w1077) -> (w1076:i32)  [unwired: 5 in, 2 out]
            n590 = dll-call lib="kernel32" fn="GlobalLock"("hGlobalMemory"=w1076) -> (w1079:i32)  [unwired: 4 in, 2 out]
            n591 = dll-call lib="kernel32" fn="lstrcpy"("Flags"=w1079, "String"=w1073) -> (w1078:i32)  [unwired: 5 in, 2 out]
            n592 = stacked-sequence {
              tunnel: w1078 -> [_]
              tunnel: w1076 -> [w1100]
              tunnel: [w1099] -> w1075
              frame #0 {
                n593 = dll-call lib="kernel32" fn="LocalUnlock"("hGlobalMemory"=w1100) -> (w1099:i32)  [unwired: 4 in, 2 out]
              }
            }
            n594 = case shown="0" w1075 {
              selector: w1075 -> [_ w1096]
              tunnel: w1076 -> [w1082 _]
              tunnel: [w1083 w1095] -> _
              frame 0 {
                n595 = dll-call lib="user32" fn="OpenClipboard"("owner"=i16 0) -> (w1084:i32)  [unwired: 4 in, 2 out]
                n596 = case shown="1, Default" w1084 {
                  selector: w1084 -> [w1088 _]
                  tunnel: [w1086 w1091] -> w1083
                  tunnel: w1082 -> [_ w1090]
                  tunnel: w1082 -> [_ _]
                  frame 0 {
                    n597 = Equal To 0?(x=w1088) -> (x = 0?=w1089:bool)
                    n598 = Bundle(w1089, w1088, "source"="Error opening clipboard") -> (w1086:cluster{bool, i32, "source":string})  [unwired: 1 in]
                  }
                  frame 1, Default {
                    n599 = stacked-sequence {
                      tunnel: [_ _ _ cluster{bool, i32, "source":string} {FALSE, 0, "source"=""} ("Output Element")] -> w1091
                      tunnel: w1090 -> [_ w1092 _ _]
                      frame #0 {
                        n600 = dll-call lib="user32" fn="EmptyClipboard"() -> ()  [unwired: 4 in, 2 out]
                      }
                      frame #1 {
                        n601 = dll-call lib="user32" fn="SetClipboardData"("Format"=1, "Data"=w1092) -> ()  [unwired: 6 in, 2 out]
                      }
                      frame #2 {
                        n602 = dll-call lib="user32" fn="CloseClipboard"() -> ()  [unwired: 4 in, 2 out]
                      }
                      frame #3 {
                      }
                    }
                  }
                }
              }
              frame 1, Default {
                n603 = Not Equal To 0?(x=w1096) -> (x != 0?=w1097:bool)
                n604 = Bundle(w1097, w1096, "source"="Error copying text to clipboard") -> (w1095:cluster{bool, i32, "source":string})  [unwired: 1 in]
              }
            }
            n605 = local write "Write Set Point Status 2"("Running" ("Status")) -> ()
          }
          frame #1 {
            # "Wait 500 milliseconds"
            n606 = Wait (ms)(milliseconds to wait=u32 500) -> ()  [unwired: 1 out]
          }
          frame #2 {
            # "Read Text From Clipboard"
            n607 = dll-call lib="user32" fn="OpenClipboard"("owner"=i16 0) -> (w1106:i32)  [unwired: 4 in, 2 out]
            n608 = case shown="1, Default" w1106 {
              selector: w1106 -> [w1112 _]
              tunnel: ["" w1117] -> w1102
              tunnel: [w1110 cluster{bool, i32, "source":string} {FALSE, 0, "source"=""} ("Output Element")] -> _
              frame 0 {
                n609 = Equal To 0?(x=w1112) -> (x = 0?=w1113:bool)
                n610 = Bundle(w1113, w1112, "source"="No text in clipboard available!") -> (w1110:cluster{bool, i32, "source":string})  [unwired: 1 in]
              }
              frame 1, Default {
                n611 = dll-call lib="user32" fn="GetClipboardData"("uFormat"=1 ("hGlobalMemory")) -> (w1118:i32)  [unwired: 4 in, 2 out]
                n612 = dll-call lib="kernel32" fn="GlobalLock"("hGlobalMemory"=w1118) -> (w1117:string, "hGlobalMemory"=w1115:i32)  [unwired: 3 in, 2 out]
                n613 = stacked-sequence {
                  tunnel: w1115 -> [w1120 _]
                  frame #0 {
                    n614 = dll-call lib="kernel32" fn="LocalUnlock"("hGlobalMemory"=w1120) -> ()  [unwired: 5 in, 2 out]
                  }
                  frame #1 {
                    n615 = dll-call lib="user32" fn="CloseClipboard"() -> ()  [unwired: 4 in, 2 out]
                  }
                }
              }
            }
            "Text Read From Clipboard 5" <- w1102
            n616 = Equal?(x=w1105, y=w1102) -> (x = y?=w1104:bool)
            n617 = case shown="True" w1104 {
              tunnel: ["Response OK" "Failed: No Response from Lab Interface"] -> w1103
              frame False {
              }
              frame True {
              }
            }
            "Write Set Point Status 2" <- w1103
          }
        }
      }
    }
    n618 = node-c288(w116) -> ()  [unwired: 1 out]
  }
  n619 = call <vilib>:"DAQmx Stop Task.vi"("task/channels in"=w16, "error in"=w15) -> ("task out"=w18:refnum<k21>, "error out"=w17:errorcluster)  [unwired: 12 in]
  n620 = Index Array(array=w45, index=0) -> (element=w47:u32)
  n621 = Index Array(array=w44, index=0) -> (element=w46:errorcluster)
  n622 = call <vilib>:"DAQmx Stop Task.vi"("task/channels in"=w5, "error in"=w3) -> ("task out"=w4:refnum<k21>, "error out"=w6:errorcluster)  [unwired: 12 in]
  n623 = call <vilib>:"DAQmx Clear Task.vi"("task in"=w18, "error in"=w17) -> ()  [unwired: 13 in, 1 out]
  n624 = call <vilib>:"DAQmx Clear Task.vi"("task in"=w4, "error in"=w6) -> ()  [unwired: 13 in, 1 out]
  n625 = call "NCS_CloseDevice.vi"("error in (no error)"=w46, "device handle"=w47) -> ()  [unwired: 1 out]
  n626 = call "CN7500_Write Set Point Value.vi"("Target Set Point Value"=25, "error in (no error)"=w33, "Controller Number"=w36, "VISA In"=w32) -> ("error out"=w38:errorcluster, "VISA Out"=w39:refnum<visa-resource-name>)  [unwired: 6 in]
  n627 = call "CN7500_Close.vi"("error in (no error)"=w38, "VISA resource name"=w39) -> ()  [unwired: 9 in, 1 out]
